vi "TI sbRIO Main (RT).vi"() -> ()   [LabVIEW 2013]
uses:
  Type Defs/Restarts Cluster.ctl
  Type Defs/Restarts Limits.ctl
  Type Defs/Controller Names.ctl
  Controls/HMI Mom Buttons.ctl
  Controls/Alarm Config.ctl
  Controls/Alarm Definition.ctl
  Controls/Alarm Profile Config.ctl
  Type Defs/App Config.ctl
  Type Defs/Actual Starts.ctl
  Type Defs/Sequence States.ctl
  Type Defs/CAN Mode.ctl
  Controls/RPi HMI Mode.ctl
  Type Defs/Controller List.ctl
  Type Defs/Pump Data Mode.ctl
  Controls/HMI Tog Buttons.ctl
  Controls/Controller Config.ctl
  SubVIs/TenHzDataArray(Global).vi
  <vilib>/FPGAPlugInAG/sbRIO-9626/niLvFpga_Open_sbRIO-9626.vi
  <vilib>/rvi/interface/common/dynamic/niFpgaDynamicAddResources.vi
  <vilib>/Utility/file.llb/Write To Spreadsheet File (DBL).vi
  SubVIs/Record Period (global).vi
  SubVIs/Record Samples (global).vi
  <vilib>/FPGAPlugInAG/Dynamic/niLvFpga_Reset_Dynamic.vi
  <vilib>/rvi/interface/common/niFpgaWaitOnOcc.vi
  <vilib>/Utility/error.llb/Error Cluster From Error Code.vi
  <vilib>/rvi/errors/niLvFpgaAdjustHostInterfaceError.vi
  <vilib>/FPGAPlugInAG/Dynamic/niLvFpga_Run_Dynamic.vi
  <vilib>/Utility/file.llb/Write To Spreadsheet File (string).vi
  <vilib>/rvi/interface/nirviOpenFPGA/nirviOpenFPGA.xnode
  FPGA/bitfiles/TI sbRIO PWM (FPGA) v1.0.lvbitx
  <vilib>/rvi/interface/nirviMethod/nirviMethod.xnode
  <vilib>/rvi/interface/nirviReadWriteControl/nirviReadWriteControl.xnode
  <vilib>/Utility/config.llb/NI_LVConfig.lvlib
  NiFpgaLv.dll
  <vilib>/NI_Real-Time Target Support.lvlib
  Real-Time/Controls/RT FIFO Mode.ctl
  <vilib>/rvi/interface/nirviCloseFPGA/nirviCloseFPGA.xnode
  Type Defs/JSON_Channel.ctl
  Type Defs/JSON_Pump.ctl
  Type Defs/JSON_Tank.ctl
  Controls/FPGA_Reference.ctl
  <vilib>/FPGAPlugInAG/sbRIO-9626/niLvFpga_Close_sbRIO-9626.vi
  <vilib>/rvi/interface/Simulation/niFpgaSimulationCallBeginRW.vi
  <vilib>/FPGAPlugInAG/sbRIO-9626/niLvFpga_Abort_sbRIO-9626.vi
panel:
  out "HMI Mom Buttons":T1
  out "TenHzPts":i32
  in  "TenHz Path":path=path "u:/TenHz/Try.csv"
  in  "Stop":bool
  in  "Alarm Tab":enum32{"Page 1", "Page 2"}(tab)
  out "Alarm Message":string
  in  "pb.Alarm OK":bool
  in  "Monitoring Tab":enum32{"Page 1", "Page 2"}(tab)
  in  "pb.E Stop":bool
  in  "Ignition Relay":T2
  in  "Power Relay":T2
  out "Voltages":dbl[](array[numeric])=[0.015201568603515625, 0.00335693359375, 0.003021240234375, 0.12260055541992188, 0.06085968017578125, 0.052234649658203125] caption="Pump\nVoltage\n(V)" format="%#.0f"
  out "Ave. Speed":dbl=7.74131899555212 format="%.1f"
  out "Temp2":dbl caption="Tank 2 Temp (C):" format="%#_2g"
  out "Temp1":dbl caption="Tank 1 Temp (C):" format="%#_2g"
  out "Pressure":dbl[](array[numeric])=[0.015201568603515625, 0.00335693359375, 0.003021240234375, 0.12260055541992188, 0.06085968017578125, 0.052234649658203125] caption="Pressure\n(kPa)" format="%#.0f"
  out "Flow":dbl[](array[numeric])=[0.0, 0.0, 0.0, 0.125, 0.0625, 0.0625] caption="Flow\n(L/H)" format="%#.0f"
  out "PumpCurrent":dbl[](array[numeric])=[0.015201568603515625, 0.00335693359375, 0.003021240234375, 0.12260055541992188, 0.06085968017578125, 0.052234649658203125] caption="Pump\nCurrent\n(RMS)" format="%#.1g"
  out "PS Actual (V):":dbl format="%.2f"
  out "ControllerCurrent":dbl[](array[numeric])=[0.015201568603515625, 0.00335693359375, 0.003021240234375, 0.12260055541992188, 0.06085968017578125, 0.052234649658203125] caption="Controller\nCurrent\n(DC)" format="%#.1g"
  out "Speed":dbl[](array[numeric]) caption="Speed\n(RPM)" format="%#_4f"
  in  "Power Supply Cmd (V):":dbl min=0.0 max=20.0 format="%#.2f"
  in  "PressureCMD":dbl caption="Pressure Cmd (kPa):" min=0.0 max=825.0 format="%#.2f"
  in  "Manual\nCMD":dbl[](array[numeric])=[0.0, 0.0, 0.0, 0.0, 0.0, 0.0] min=5.0 max=50.0 step=0.1 format="%#.2f"
  in  "pb.Zero CMDs":bool
  out "CPU Usage:":dbl=7.74131899555212 format="%.1f"
  in  "Pumps Present":T2={"Pump 1"=TRUE, "Pump 2"=TRUE, "Pump 3"=TRUE, "Pump 4"=TRUE, "Pump 5"=TRUE, "Pump 6"=TRUE}
  out "CAN CMD":dbl
  in  "Restarts Tab":enum32{"Page 1", "Page 2"}(tab)
  in  "Restarts Limits":T3={"High Limits:"=[30, 30, 30, 30, 30, 30], "Low Limits:"=[30, 30, 30, 30, 30, 30]}
  in  "pb.Rst Tot Restarts":bool
  in  "pb.Reset Restarts":bool
  in  "Inform:":string="Input email address on Email Handler program on Lab 4 PC."
  out "Restarts Cluster":T4
  out "Client?":bool
  in  "Title Tab":enum32{"Page 1", "Page 2"}(tab)
  in  "Title":string="TI Automotive sbRIO Pulse, v1.2"
  in  "Login":bool
  in  "Set Time Tab":enum32{"Page 1", "Page 2"}(tab)
  in  "pb.Set Time OK":bool
  in  "pb.Set Time Cancel":bool
  in  "New Time":dbl format="%<%H:%M:%S>t"
  in  "Reset Tab":enum32{"Page 1", "Page 2"}(tab)
  in  "pb.Reset OK":bool
  in  "pb.Reset Cancel":bool
  in  "pb.Stop Profile":bool
  in  "Save As Tab":enum32{"Page 1", "Page 2"}(tab)
  in  "New Profile Name:":string
  in  "pb.Save As OK":bool
  in  "pb.Save As Cancel":bool
  in  "Main Tab":enum32{"Main", "Data Stream", "Alarms"}(tab)
  in  "Profile:":string[][](table)=[["1", "2.0", "0.0", "0.0", "0.0", "67.6", "67.6", "67.6"], ["2", "1.0", "0.0", "0.0", "0.0", "10.0", "10.0", "10.0"]]
  in  "Controller Type:":T5
  in  "pb.FuelChange":bool
  in  "Tank 1 Fuel Type":string
  in  "Tank 2 Fuel Type":string
  in  "Stagger Time (ms):":i32
  in  "pb.Time Reset All":bool
  in  "CA Number:":string
  in  "Profile Name:":string(combo)="test"
  in  "pb.Save As":bool
  out "Current Step:":i32=2
  out "Step Time Left:":dbl=0.21101045608520508
  out "Cycles Completed:":u32=17
  in  "pb.Cycle Reset":bool
  out "Location:":string
  in  "pb.Run Profile":bool
  out "Elapsed Time:":dbl[](array[numeric])=[7.1, 7.1, 7.1, 458133.45, 458138.85000000003, 458126.75] format="%<%H:%M:%S>t"
  in  "pb.Resets":bool[](array[boolean])=[FALSE, FALSE, FALSE, FALSE, FALSE, FALSE]
  in  "pb.Sets":bool[](array[boolean])=[FALSE, FALSE, FALSE, FALSE, FALSE, FALSE]
  in  "Serial Numbers":T6
  in  "pb.TenHzSave":bool
  in  "Record Frequency:":i32=10 min=1 max=10 step=1
  in  "pb.Reset Cogs":bool
  in  "Cog Limits:":i32[](array[numeric])=[30, 30, 30, 30, 30, 30] min=0
  out "Cog Events:":i32[](array[numeric])
  out "Graph":dbl[](graph)
  in  "RPMhyst":fxp<+,25,6>=0.20000076293945312
  in  "Solenoid 3":bool caption="Fuel Solenoid 3"
  in  "Solenoid 2":bool caption="Fuel Solenoid 2"
  in  "Solenoid 1":bool caption="Fuel Solenoid 1"
  in  "3 Pulsing":bool caption="Module 3 Pulsing"
  in  "3 Pulse Duty%":dbl=60.0 caption="Module 3 Pulse Duty%" min=0.0 max=100.0 step=0.1 format="%#.2f"
  in  "2 Pulsing":bool caption="Module 2 Pulsing"
  in  "2 Pulse Duty%":dbl=60.0 caption="Module 2 Pulse Duty%" min=0.0 max=100.0 step=0.1 format="%#.2f"
  in  "1 Pulsing":bool caption="Module 1 Pulsing"
  in  "1 Pulse Duty%":dbl=60.0 caption="Module 1 Pulse Duty%" min=0.0 max=100.0 step=0.1 format="%#.2f"
  in  "Pulse Frequency":dbl=20.0 min=0.5 max=40.0 step=0.1 format="%#.2f"
  in  "SubRoutine Profile":i32[][](array[numeric]) caption="Profile #:   Cycles:" min=1 step=1
  in  "pb.Run SubRoutines":bool
  in  "Alarm Config":T7
  # "Manual Control"
  # "Monitoring"
  # "Restarts Monitor"
  # "Enter a new elapsed time."
  # "Are you sure you want to reset?"
  # "Under Development"
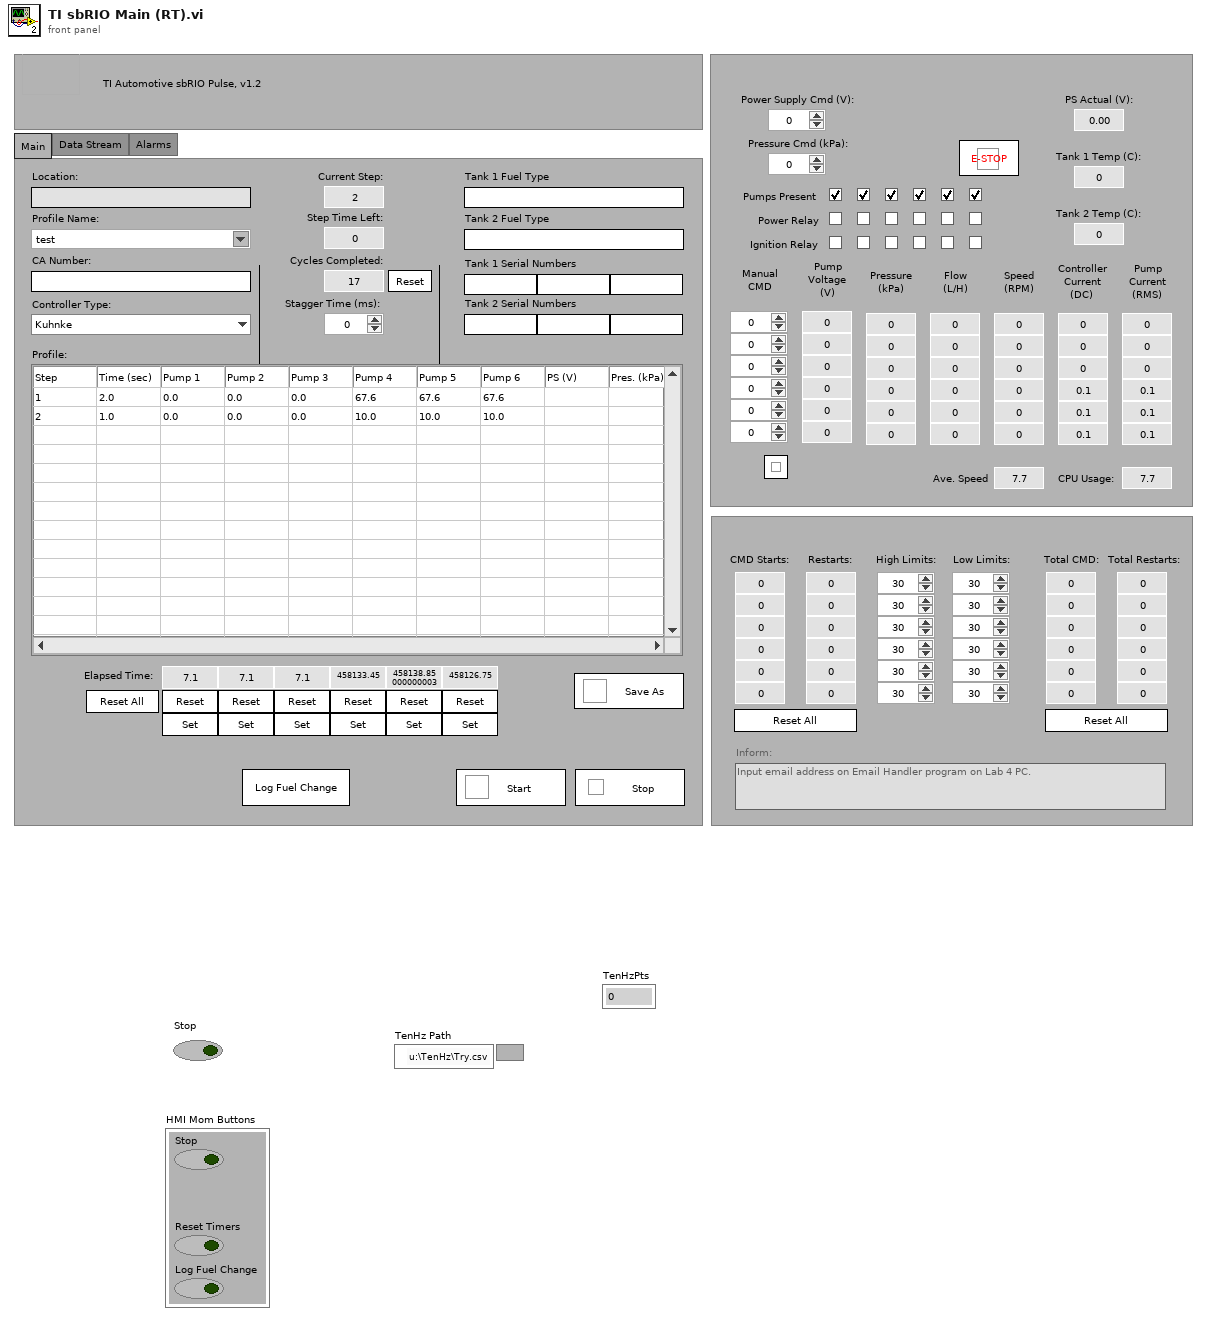
[diagram p1: front panel]
types:
  T1 = typedef "HMI Mom Buttons.ctl" = cluster{"Stop":bool, "Reset Timers":bool, "Log Fuel Change":bool}
  T2 = cluster{"Pump 1":bool, "Pump 2":bool, "Pump 3":bool, "Pump 4":bool, "Pump 5":bool, "Pump 6":bool}
  T3 = typedef "Restarts Limits.ctl" = cluster{"High Limits:":i32[], "Low Limits:":i32[]}
  T4 = typedef "Restarts Cluster.ctl" = cluster{"CMD Starts:":i32[], "Restarts:":i32[], "Total CMD:":i32[], "Total Restarts:":i32[]}
  T5 = typedef "Controller Names.ctl" = enum16{"Kuhnke", "Conti", "Helbako", "TI PWM", "PSA", "Hella Gas", "Hella Diesel", "8 Comm", "10 Comm", "8 Comm Hella", "10 Comm Hella", "8 Comm Omron", "10 Comm Omron", "8 Comm Nissan", "10 Comm Nissan"}
  T6 = cluster{"Position 1 SN":string, "Position 2 SN":string, "Position 3 SN":string, "Position 4 SN":string, "Position 5 SN":string, "Position 6 SN":string}
  T7 = typedef "Alarm Config.ctl" = cluster{"Alarms:":T8[], "Profile Sync:":T9}
  T8 = typedef "Alarm Definition.ctl" = cluster{"Description:":string, "Enabled:":bool, "Data Index:":i32, "Data Type:":string, "Low Limit:":dbl, "High Limit:":dbl, "Trip Time:":u32, "Profile Sync:":bool}
  T9 = typedef "Alarm Profile Config.ctl" = cluster{"Trip Time:":u32, "Consecutive Trips:":i32}
  T10 = typedef "Controller List.ctl" = cluster{"Controller Name":T5, "CommSeg":i32, "PWM?":bool, "Frequency":i32, "Low Command":dbl, "High Command":dbl, "Stop Command":dbl, "Command Step":dbl, "Solenoid Stop?":bool, "Controller?":bool, "Invert PWM":bool}[]
  T11 = cluster{"Controller Name":T5, "CommSeg":i32, "PWM?":bool, "Frequency":i32, "Low Command":dbl, "High Command":dbl, "Stop Command":dbl, "Command Step":dbl, "Solenoid Stop?":bool, "Controller?":bool, "Invert PWM":bool}
  T12 = typedef "RPi HMI Mode.ctl" = enum16{"Init", "Write Data", "Read from RPi", "Write to RPi"}
  T13 = typedef "CAN Mode.ctl" = enum16{"Init", "Read", "Write", "Close"}
  T14 = typedef "Sequence States.ctl" = enum16{"Main", "Init Files", "Init", "Save As", "Start Profile", "Check Step Time", "Alarm", "Run Step", "Stop Profile", "Cycle Reset", "Time Reset", "Time Reset All", "Time Set", "Tare CTs", "Save Profile", "Open Profile", "Get Profiles", "Update Screen", "Save Status", "Set Manual CMD", "Reset Restarts", "Reset Total Restarts", "Reset Cogs", "Disable Background", "Enable Background", "Get/Release Control", "Init AKLH", "Save AKLH", "Log Fuel Change", "Update Data Stream", "Init TenHz", "Read TenHz", "Remote Timer Reset", "Record Frequency Change", "Controller Change", "Get Alarms", "Init Alarms", "Save Alarms", "Init SubRoutine", "Next SubRoutine"}
  T15 = typedef "Actual Starts.ctl" = cluster{"Actual Pump Starts":i32[], "Initial Actual Starts":i32[], "Tot Act Starts":i32[], "Tot Init Act Starts":i32[]}
  T16 = typedef "App Config.ctl" = cluster{"Location":string, "Profiles Path":path, "Current Profile":string, "CA Number":string, "Cycles Completed":u32, "PWM Freq (Hz)":dbl, "Controller Type:":T5, "Inform":string, "Pumps Present":u32, "Stagger Time (ms)":i32, "Tank 1 Fuel":string, "Tank 2 Fuel":string, "Serial Numbers":cluster{"Position 1 SN":string, "Position 2 SN":string, "Poaition 3 SN":string, "Position 4 SN":string, "Position 5 SN":string, "Position 6 SN":string}, "Record TenHz":bool, "VoltCtrlRef":string, "TenHzFrequency":u32}
  T17 = cluster{"Error":errorcluster, "Profile":string[][], "App Config":T16, "Profiles":string[], "Current Step":i32, "Step Time Left":dbl, "Run Profile":bool, "Step Start Time":dbl, "Step Time":dbl, " # of Steps":i32, "Last Update":dbl, "Update Screen":bool, "Last Profile Time":dbl, "Manual CMDs":dbl[], "Client?":bool, "pb.Run Profile":bool, "pb.Resets":bool[], "pb.Sets":bool[], "Last CMDs":dbl[], "Update Profile":bool, "Elapsed Times":dbl[], "Intitial Times":dbl[], "Alarm":bool, "CT Offsets":fxp<+/-,26,7>[], "Pumps Present":cluster{"Pump 1":bool, "Pump 2":bool, "Pump 3":bool, "Pump 4":bool, "Pump 5":bool, "Pump 6":bool}, "Login":bool, "Stagger Counter":i32, "New Step":bool, "Restarts Limits":T3, "Restarts Cluster":T4, "Actual Starts":T15, "AKLH Path":path, "TenHz Path":path, "AKLH Timer":dbl, "TenHz Timer":dbl, "TenHz Active?":bool, "AKLH Last Hour":i32, "Main Tab":enum32{"Page 1", "Page 2"}, "Stop Cmd":dbl, "Tank Data":dbl[], "CogCounters":i32[], "Cog Events":i32[], "Voltage Enable":bool, "Cog Limits:":i32[], "TenHz Day":i32, "Controller":cluster{"Controller Name":T5, "CommSeg":i32, "PWM?":bool, "Frequency":i32, "Low Command":dbl, "High Command":dbl, "Stop Command":dbl, "Command Step":dbl, "Solenoid Stop?":bool, "Controller?":bool, "Invert PWM":bool}, "PS CMD":dbl, "Press CMD":dbl, "Temp CMD":dbl, "Power Relay":cluster{"Pump 1":bool, "Pump 2":bool, "Pump 3":bool, "Pump 4":bool, "Pump 5":bool, "Pump 6":bool}, "Ignition Relay":cluster{"Pump 1":bool, "Pump 2":bool, "Pump 3":bool, "Pump 4":bool, "Pump 5":bool, "Pump 6":bool}, "Controller List":T10, "Alarm Config":T7, "Alarm Config Path":path, "Trip Counters":i32[], "Previous Times":u32[], "Alarm Message":string, "Restart Alarm":bool, "Pulse Frequency":dbl, "1 Pulse Duty%":dbl, "2 Pulse Duty%":dbl, "3 Pulse Duty%":dbl, "1 Pulsing":bool, "Solenoid 1":bool, "2 Pulsing":bool, "Solenoid 2":bool, "3 Pulsing":bool, "Solenoid 3":bool, "SubRoutine Profile":i32[][], "Profile #":i32, "ReqCycles":u32, "Run Subs":bool, "SR Step":u32}
  T18 = typedef "HMI Cluster.ctl" = cluster{"Error":errorcluster, "COM Ref":refnum<visa-resource-name>, "Pump Data":T19, "Tank Data":cluster{"PS Actual (V):":dbl, "Temp1":dbl, "Temp2":dbl}, "Power Relays":cluster{"Pump 1":bool, "Pump 2":bool, "Pump 3":bool, "Pump 4":bool, "Pump 5":bool, "Pump 6":bool}, "Pump CMDs":dbl[], "HMI Header":T20, "Tank CMDs":T21, "HMI Tog Buttons":T22, "In Test":bool, "HMI Command":bool, "HMI Mom Buttons":T1, "Controller Config":T23}
  T19 = typedef "Pump Data.ctl" = cluster{"Voltages":dbl[], "PumpCurrent":dbl[], "Speed":dbl[], "ControllerCurrent":dbl[], "Pressure":dbl[], "Flow":dbl[], "Elapsed Time:":dbl[]}
  T20 = typedef "HMI Header.ctl" = cluster{"Line 1":string, "Line 2":string, "Line 3":string}
  T21 = typedef "Tank CMDs.ctl" = cluster{"PS CMD":dbl, "Press CMD":dbl, "Temp CMD":dbl}
  T22 = typedef "HMI Tog Buttons.ctl" = cluster{"Start Test":bool, "Toggle Spare 1":bool, "Toggle Spare 2":bool, "Toggle Spare 3":bool, "Toggle Spare 4":bool, "Toggle Spare 5":bool}
  T23 = typedef "Controller Config.ctl" = cluster{"Controller List":string, "Controller Type:":T5, "CMD Max":i32, "CMD Inc":i32}
  T24 = typedef "RT FIFO Mode.ctl" = enum16{"Create", "Write", "Read", "Delete"}
  T25 = typedef "FPGA_Reference.ctl" = refnum<k20>
  T26 = typedef "Pump Data Mode.ctl" = enum16{"Read", "Write Data", "Write Cal"}
  T27 = enum8{"Enabled", "Disabled", "Disabled and Grayed Out"}
  T28 = typedef "JSON_Tank.ctl" = cluster{"number":u16, "building":string, "room":string, "ipAddress":string, "profileName":string, "caNumber":string, "ctrlType":string, "mode":string, "channels":T29[], "pumps":T30[]}
  T29 = typedef "JSON_Channel.ctl" = cluster{"name":string, "tag":string, "data":string, "type":string, "unit":string}
  T30 = typedef "JSON_Pump.ctl" = cluster{"position":u8, "enabled":bool, "command":string, "channels":T29[], "elapsedTime":string}
  T31 = cluster{"Position 1 SN":string, "Position 2 SN":string, "Poaition 3 SN":string, "Position 4 SN":string, "Position 5 SN":string, "Position 6 SN":string}
  T32 = typedef "Test Action.ctl" = enum16{"Idle", "Start", "Stop", "Pump Cmd", "Pump 1 Enable", "Pump 2 Enable", "Pump 3 Enable", "Pump 4 Enable", "Pump 5 Enable", "Pump 6 Enable", "Timer 1 Reset", "Timer 2 Reset", "Timer 3 Reset", "Timer 4 Reset", "Timer 5 Reset", "Timer 6 Reset"}
  T33 = cluster{"Boolean array[0]":bool, "Boolean array[1]":bool, "Boolean array[2]":bool, "Boolean array[3]":bool, "Boolean array[4]":bool, "Boolean array[5]":bool}
  T34 = typedef "LVDateTimeRec.ctl" = cluster{"fractional second":dbl, "second":i32, "minute":i32, "hour":i32, "day of month":i32, "month":i32, "year":i32, "day of week":i32, "day of year":i32, "DST":i32}
  T35 = typedef "NI_LVConfig.lvlib/Config Data RefNum.ctl" = refnum<k1>
  T36 = cluster{dbl, dbl, dbl, dbl, dbl, dbl, dbl, dbl, dbl, dbl, dbl, dbl}
  T37 = cluster{"PS Actual (V):":dbl, "Temp1":dbl, "Temp2":dbl}
  T38 = cluster{"Location":string, "Current Profile":string, "CA Number":string}
  T39 = cluster{"PS CMD":dbl, "Press CMD":dbl, "Temp CMD":dbl}
  T40 = typedef "LVRemotePanelConnectionsTypeDef.ctl" = cluster{"VI Name":string, "Remote":string, "UserName":string, "Port":i32, "Status":enum32{"Viewing", "Waiting For Control", "Controlling"}, "Create Time":timestamp, "Status Time":timestamp, "Control End Time":timestamp}[]
  T41 = typedef "NI_Real-Time Target Support.lvlib/RT CPU Load.ctl" = cluster{"Total (%)":dbl, "Time Critical (%)":dbl, "Timed Structures (%)":dbl, "High (%)":dbl, "Above Normal (%)":dbl, "Normal (%)":dbl, "Background (%)":dbl, "Idle (%)":dbl, "ISR (%)":dbl}
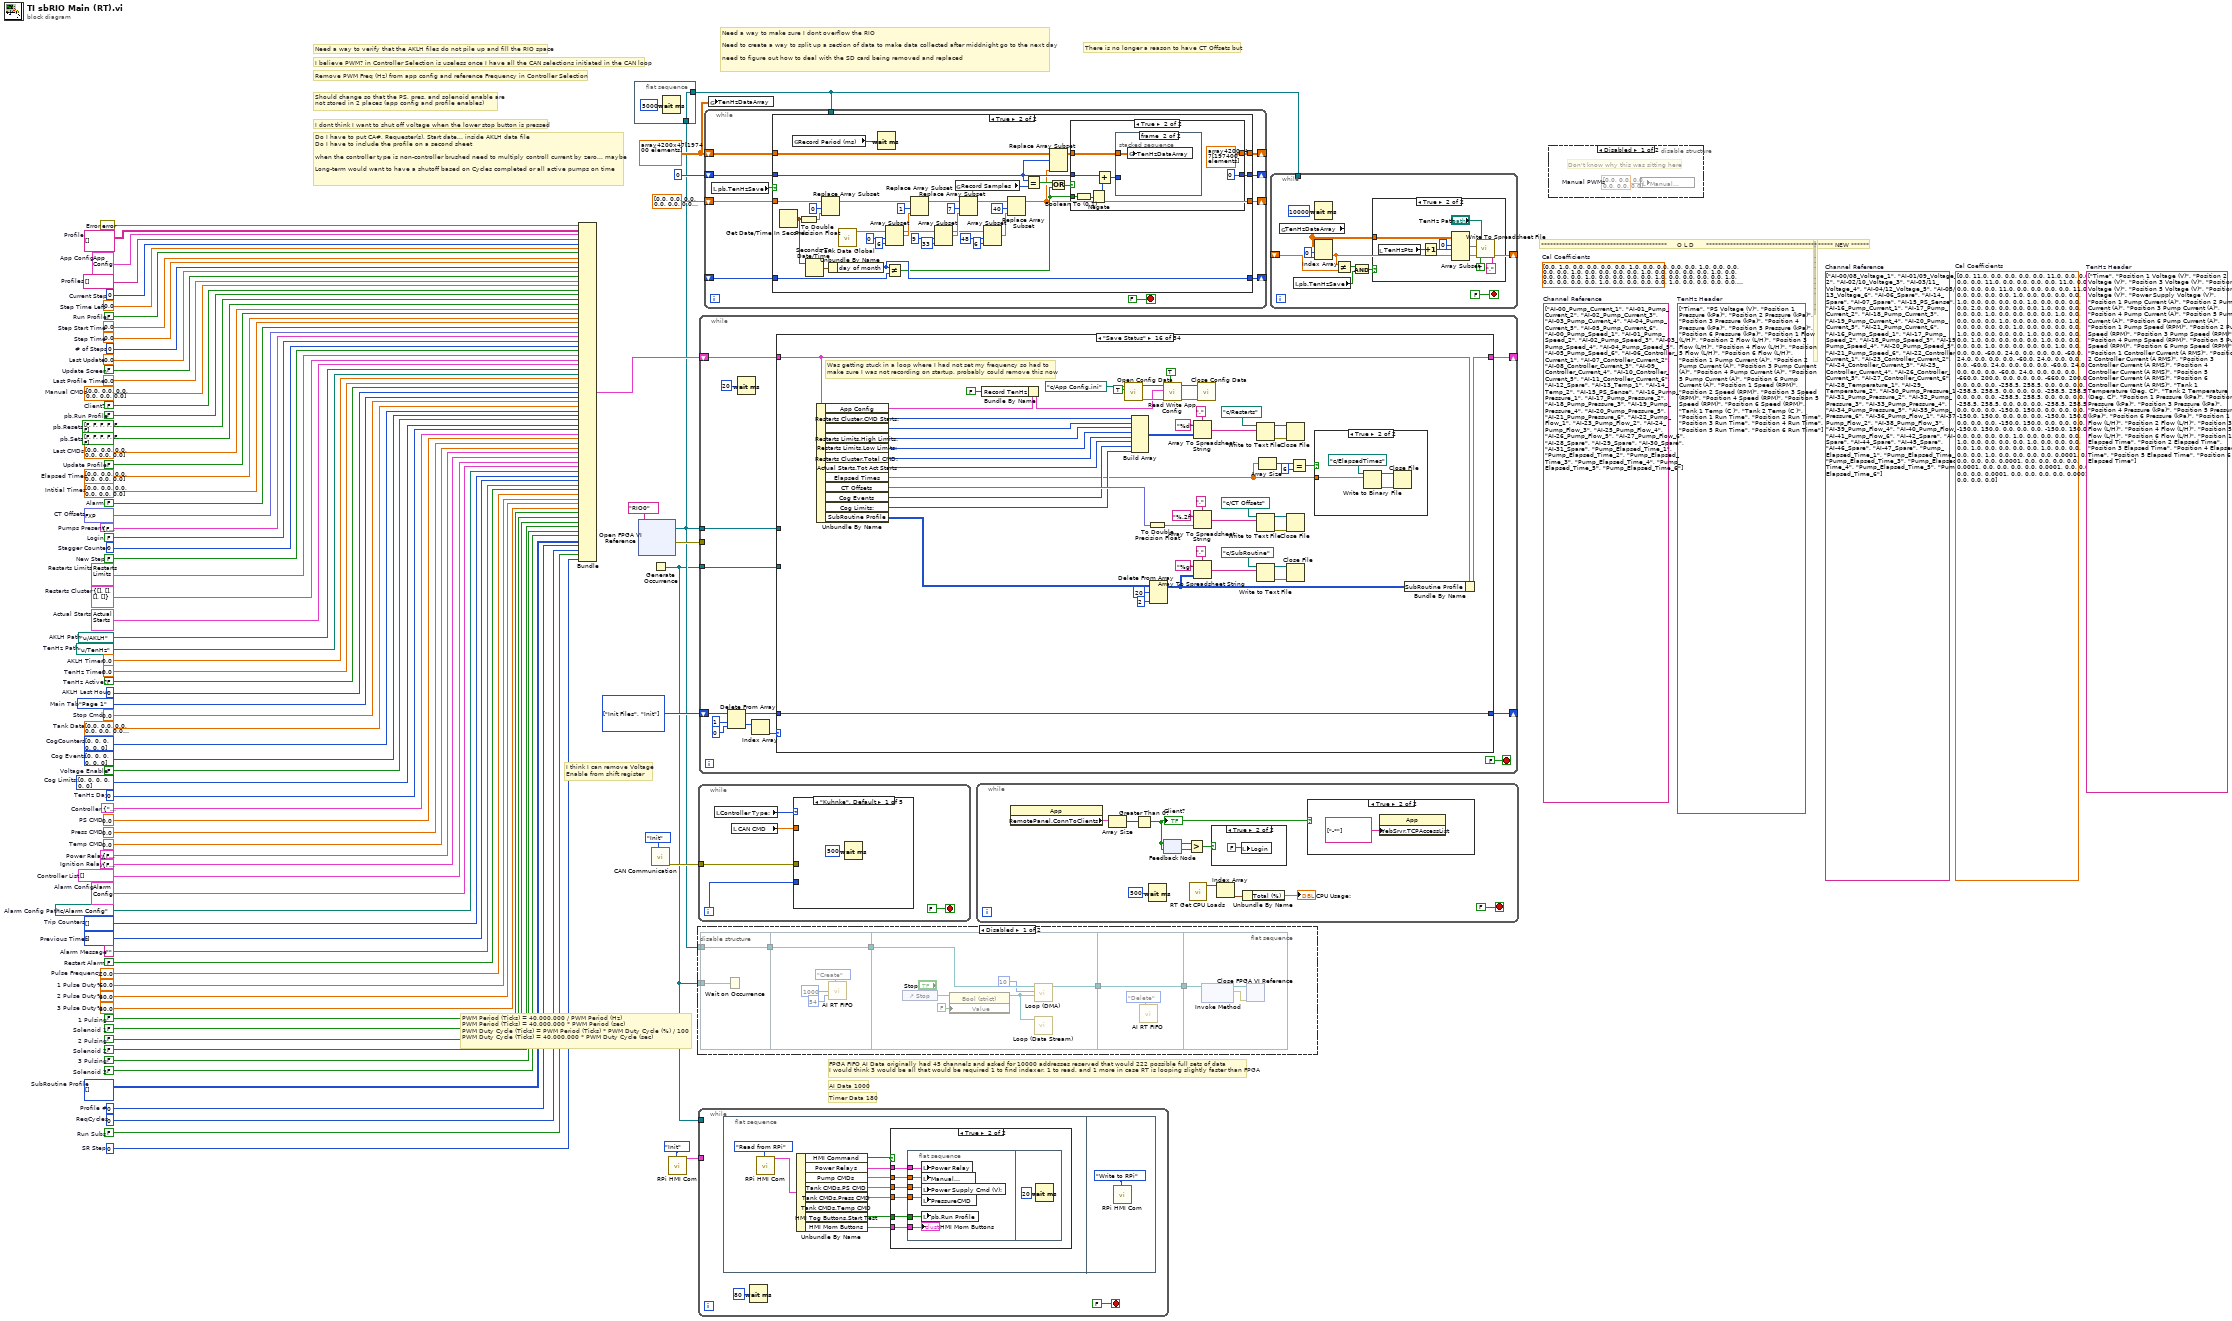
[diagram p0: block diagram]
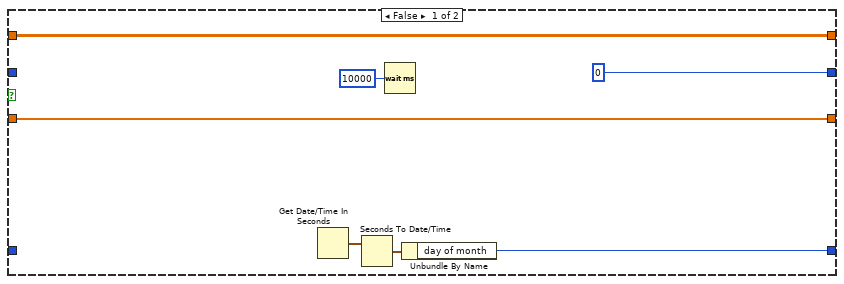
[diagram p5: hidden frame]
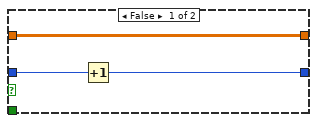
[diagram p6: hidden frame]
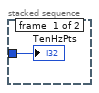
[diagram p7: hidden frame]
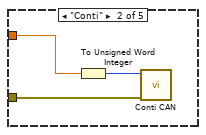
[diagram p8: hidden frame]
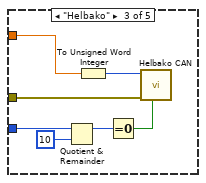
[diagram p9: hidden frame]
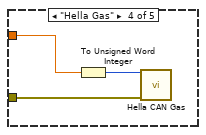
[diagram p10: hidden frame]
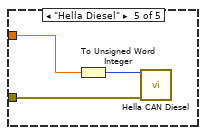
[diagram p11: hidden frame]
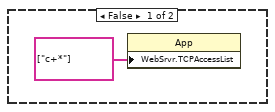
[diagram p12: hidden frame]
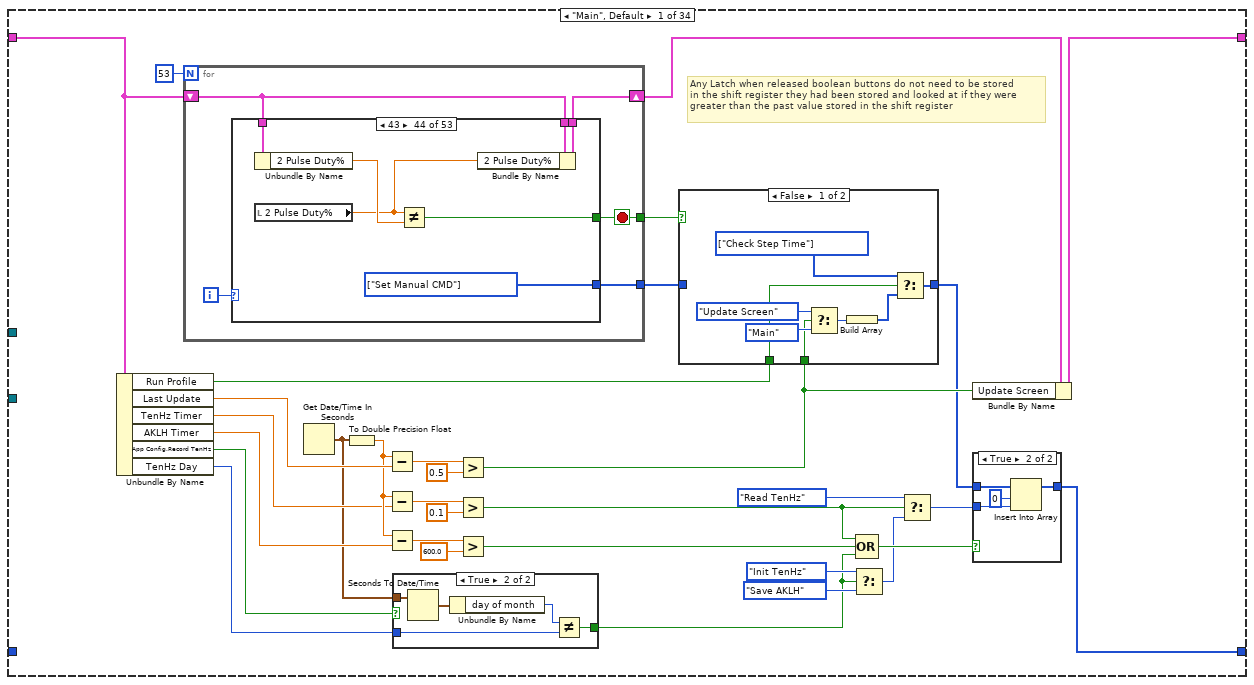
[diagram p15: hidden frame]
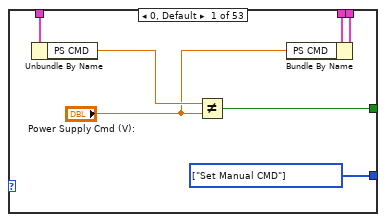
[diagram p18: hidden frame]
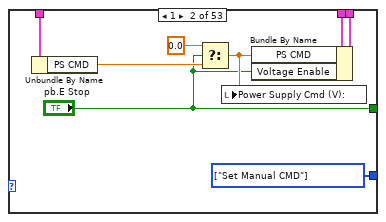
[diagram p19: hidden frame]
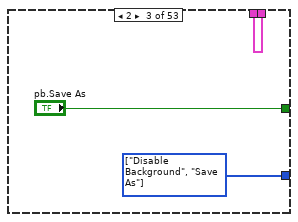
[diagram p20: hidden frame]
diagram:
  w5 = u32 0  # SR Step
  w4 = FALSE  # Run Subs
  w3 = u32 0  # ReqCycles
  w2 = 0  # Profile #
  w1 = i32[][] []  # SubRoutine Profile
  w6 = FALSE  # Solenoid 3
  w7 = FALSE  # 3 Pulsing
  w8 = FALSE  # Solenoid 2
  w9 = FALSE  # 2 Pulsing
  w10 = FALSE  # Solenoid 1
  w11 = FALSE  # 1 Pulsing
  w12 = 60.0  # 3 Pulse Duty%
  w13 = 60.0  # 2 Pulse Duty%
  w14 = 60.0  # 1 Pulse Duty%
  w15 = 20.0  # Pulse Frequency
  w16 = FALSE  # Restart Alarm
  w17 = ""  # Alarm Message
  w18 = u32[] []  # Previous Times
  w19 = i32[] []  # Trip Counters
  w20 = path "c:/Alarm Config"  # Alarm Config Path
  w21 = T7 {"Alarms:"=[{"Description:"="", "Enabled:"=FALSE, "Data Index:"=0, "Data Type:"="", "Low Limit:"=0.0, "High Limit:"=0.0, "Trip Time:"=0, "Profile Sync:"=FALSE}, {"Description:"="", "Enabled:"=FALSE, "Data Index:"=0, "Data Type:"="", "Low Limit:"=0.0, "High Limit:"=0.0, "Trip Time:"=0, "Profile Sync:"=FALSE}, {"Description:"="", "Enabled:"=FALSE, "Data Index:"=0, "Data Type:"="", "Low Limit:"=0.0, "High Limit:"=0.0, "Trip Time:"=0, "Profile Sync:"=FALSE}, {"Description:"="", "Enabled:"=FALSE, "Data Index:"=0, "Data Type:"="", "Low Limit:"=0.0, "High Limit:"=0.0, "Trip Time:"=0, "Profile Sync:"=FALSE}, {"Description:"="", "Enabled:"=FALSE, "Data Index:"=0, "Data Type:"="", "Low Limit:"=0.0, "High Limit:"=0.0, "Trip Time:"=0, "Profile Sync:"=FALSE}, {"Description:"="", "Enabled:"=FALSE, "Data Index:"=0, "Data Type:"="", "Low Limit:"=0.0, "High Limit:"=0.0, "Trip Time:"=0, "Profile Sync:"=FALSE}, {"Description:"="", "Enabled:"=FALSE, "Data Index:"=0, "Data Type:"="", "Low Limit:"=0.0, "High Limit:"=0.0, "Trip Time:"=0, "Profile Sync:"=FALSE}, {"Description:"="", "Enabled:"=FALSE, "Data Index:"=0, "Data Type:"="", "Low Limit:"=0.0, "High Limit:"=0.0, "Trip Time:"=0, "Profile Sync:"=FALSE}], "Profile Sync:"={"Trip Time:"=0, "Consecutive Trips:"=0}}  # Alarm Config
  w22 = T10 []  # Controller List
  w23 = T11 {"Controller Name"=enum."Kuhnke", "CommSeg"=2, "PWM?"=TRUE, "Frequency"=100, "Low Command"=10.0, "High Command"=100.0, "Stop Command"=10.0, "Command Step"=0.1, "Solenoid Stop?"=FALSE, "Controller?"=TRUE, "Invert PWM"=FALSE}  # Controller
  w27 = T2 {"Pump 1"=FALSE, "Pump 2"=FALSE, "Pump 3"=FALSE, "Pump 4"=FALSE, "Pump 5"=FALSE, "Pump 6"=FALSE}  # Ignition Relay
  w28 = T2 {"Pump 1"=FALSE, "Pump 2"=FALSE, "Pump 3"=FALSE, "Pump 4"=FALSE, "Pump 5"=FALSE, "Pump 6"=FALSE}  # Power Relay
  w29 = 0.0  # Temp CMD
  w30 = 0.0  # Press CMD
  w31 = 0.0  # PS CMD
  (unwired) string[] ["Time", "Position 1 Voltage (V)", "Position 2 Voltage (V)", "Position 3 Voltage (V)", "Position 4 Voltage (V)", "Position 5 Voltage (V)", "Position 6 Voltage (V)", "Power Supply Voltage (V)", "Position 1 Pump Current (A)", "Position 2 Pump Current (A)", "Position 3 Pump Current (A)", "Position 4 Pump Current (A)", "Position 5 Pump Current (A)", "Position 6 Pump Current (A)", "Position 1 Pump Speed (RPM)", "Position 2 Pump Speed (RPM)", "Position 3 Pump Speed (RPM)", "Position 4 Pump Speed (RPM)", "Position 5 Pump Speed (RPM)", "Position 6 Pump Speed (RPM)", "Position 1 Controller Current (A RMS)", "Position 2 Controller Current (A RMS)", "Position 3 Controller Current (A RMS)", "Position 4 Controller Current (A RMS)", "Position 5 Controller Current (A RMS)", "Position 6 Controller Current (A RMS)", "Tank 1 Temperature (Deg. C)", "Tank 2 Temperature (Deg. C)", "Position 1 Pressure (kPa)", "Position 2 Pressure (kPa)", "Position 3 Pressure (kPa)", "Position 4 Pressure (kPa)", "Position 5 Pressure (kPa)", "Position 6 Pressure (kPa)", "Position 1 Flow (L/H)", "Position 2 Flow (L/H)", "Position 3 Flow (L/H)", "Position 4 Flow (L/H)", "Position 5 Flow (L/H)", "Position 6 Flow (L/H)", "Position 1 Elapsed Time", "Position 2 Elapsed Time", "Position 3 Elapsed Time", "Position 4 Elapsed Time", "Position 5 Elapsed Time", "Position 6 Elapsed Time"]  # TenHz Header
  (unwired) dbl[][] [[0.0, 11.0, 0.0, 0.0, 0.0], [0.0, 11.0, 0.0, 0.0, 0.0], [0.0, 11.0, 0.0, 0.0, 0.0], [0.0, 11.0, 0.0, 0.0, 0.0], [0.0, 11.0, 0.0, 0.0, 0.0], [0.0, 11.0, 0.0, 0.0, 0.0], [0.0, 1.0, 0.0, 0.0, 0.0], [0.0, 1.0, 0.0, 0.0, 0.0], [0.0, 1.0, 0.0, 0.0, 0.0], [0.0, 2.0, 0.0, 0.0, 0.0], [0.0, 1.0, 0.0, 0.0, 0.0], [0.0, 1.0, 0.0, 0.0, 0.0], [0.0, 1.0, 0.0, 0.0, 0.0], [0.0, 1.0, 0.0, 0.0, 0.0], [0.0, 1.0, 0.0, 0.0, 0.0], [0.0, 1.0, 0.0, 0.0, 0.0], [0.0, 1.0, 0.0, 0.0, 0.0], [0.0, 1.0, 0.0, 0.0, 0.0], [0.0, 1.0, 0.0, 0.0, 0.0], [0.0, 1.0, 0.0, 0.0, 0.0], [0.0, 1.0, 0.0, 0.0, 0.0], [0.0, 1.0, 0.0, 0.0, 0.0], [-60.0, 24.0, 0.0, 0.0, 0.0], [-60.0, 24.0, 0.0, 0.0, 0.0], [-60.0, 24.0, 0.0, 0.0, 0.0], [-60.0, 24.0, 0.0, 0.0, 0.0], [-60.0, 24.0, 0.0, 0.0, 0.0], [-60.0, 24.0, 0.0, 0.0, 0.0], [-660.0, 200.0, 0.0, 0.0, 0.0], [-660.0, 200.0, 0.0, 0.0, 0.0], [-258.5, 258.5, 0.0, 0.0, 0.0], [-258.5, 258.5, 0.0, 0.0, 0.0], [-258.5, 258.5, 0.0, 0.0, 0.0], [-258.5, 258.5, 0.0, 0.0, 0.0], [-258.5, 258.5, 0.0, 0.0, 0.0], [-258.5, 258.5, 0.0, 0.0, 0.0], [-150.0, 150.0, 0.0, 0.0, 0.0], [-150.0, 150.0, 0.0, 0.0, 0.0], [-150.0, 150.0, 0.0, 0.0, 0.0], [-150.0, 150.0, 0.0, 0.0, 0.0], [-150.0, 150.0, 0.0, 0.0, 0.0], [-150.0, 150.0, 0.0, 0.0, 0.0], [0.0, 1.0, 0.0, 0.0, 0.0], [0.0, 1.0, 0.0, 0.0, 0.0], [0.0, 1.0, 0.0, 0.0, 0.0], [0.0, 1.0, 0.0, 0.0, 0.0], [0.0, 1.0, 0.0, 0.0, 0.0], [0.0, 1.0, 0.0, 0.0, 0.0], [0.0, 0.0001, 0.0, 0.0, 0.0], [0.0, 0.0001, 0.0, 0.0, 0.0], [0.0, 0.0001, 0.0, 0.0, 0.0], [0.0, 0.0001, 0.0, 0.0, 0.0], [0.0, 0.0001, 0.0, 0.0, 0.0], [0.0, 0.0001, 0.0, 0.0, 0.0]]  # Cal Coefficients
  (unwired) dbl[][] [[0.0, 1.0, 0.0, 0.0, 0.0], [0.0, 1.0, 0.0, 0.0, 0.0], [0.0, 1.0, 0.0, 0.0, 0.0], [0.0, 1.0, 0.0, 0.0, 0.0], [0.0, 1.0, 0.0, 0.0, 0.0], [0.0, 1.0, 0.0, 0.0, 0.0], [0.0, 1.0, 0.0, 0.0, 0.0], [0.0, 1.0, 0.0, 0.0, 0.0], [0.0, 1.0, 0.0, 0.0, 0.0], [0.0, 1.0, 0.0, 0.0, 0.0], [0.0, 1.0, 0.0, 0.0, 0.0], [0.0, 1.0, 0.0, 0.0, 0.0], [-60.0, 24.0, 0.0, 0.0, 0.0], [-60.0, 24.0, 0.0, 0.0, 0.0], [-60.0, 24.0, 0.0, 0.0, 0.0], [-60.0, 24.0, 0.0, 0.0, 0.0], [-60.0, 24.0, 0.0, 0.0, 0.0], [-60.0, 24.0, 0.0, 0.0, 0.0], [0.0, 1.0, 0.0, 0.0, 0.0], [-660.0, 200.0, 0.0, 0.0, 0.0], [-660.0, 200.0, 0.0, 0.0, 0.0], [0.0, 2.0, 0.0, 0.0, 0.0], [-258.5, 258.5, 0.0, 0.0, 0.0], [-258.5, 258.5, 0.0, 0.0, 0.0], [-258.5, 258.5, 0.0, 0.0, 0.0], [-258.5, 258.5, 0.0, 0.0, 0.0], [-258.5, 258.5, 0.0, 0.0, 0.0], [-258.5, 258.5, 0.0, 0.0, 0.0], [-150.0, 150.0, 0.0, 0.0, 0.0], [-150.0, 150.0, 0.0, 0.0, 0.0], [-150.0, 150.0, 0.0, 0.0, 0.0], [-150.0, 150.0, 0.0, 0.0, 0.0], [-150.0, 150.0, 0.0, 0.0, 0.0], [-150.0, 150.0, 0.0, 0.0, 0.0], [0.0, 1.0, 0.0, 0.0, 0.0], [0.0, 1.0, 0.0, 0.0, 0.0], [0.0, 1.0, 0.0, 0.0, 0.0], [0.0, 1.0, 0.0, 0.0, 0.0], [0.0, 0.0001, 0.0, 0.0, 0.0], [0.0, 0.0001, 0.0, 0.0, 0.0], [0.0, 0.0001, 0.0, 0.0, 0.0], [0.0, 0.0001, 0.0, 0.0, 0.0], [0.0, 0.0001, 0.0, 0.0, 0.0], [0.0, 0.0001, 0.0, 0.0, 0.0]]  # Cal Coefficients
  (unwired) string[] ["AI-00/08_Voltage_1", "AI-01/09_Voltage_2", "AI-02/10_Voltage_3", "AI-03/11_Voltage_4", "AI-04/12_Voltage_5", "AI-05/13_Voltage_6", "AI-06_Spare", "AI-14_Spare", "AI-07_Spare", "AI-15_PS_Sense", "AI-16_Pump_Current_1", "AI-17_Pump_Current_2", "AI-18_Pump_Current_3", "AI-19_Pump_Current_4", "AI-20_Pump_Current_5", "AI-21_Pump_Current_6", "AI-16_Pump_Speed_1", "AI-17_Pump_Speed_2", "AI-18_Pump_Speed_3", "AI-19_Pump_Speed_4", "AI-20_Pump_Speed_5", "AI-21_Pump_Speed_6", "AI-22_Controller_Current_1", "AI-23_Controller_Current_2", "AI-24_Controller_Current_3", "AI-25_Controller_Current_4", "AI-26_Controller_Current_5", "AI-27_Controller_Current_6", "AI-28_Temperature_1", "AI-29_Temperature_2", "AI-30_Pump_Pressure_1", "AI-31_Pump_Pressure_2", "AI-32_Pump_Pressure_3", "AI-33_Pump_Pressure_4", "AI-34_Pump_Pressure_5", "AI-35_Pump_Pressure_6", "AI-36_Pump_Flow_1", "AI-37_Pump_Flow_2", "AI-38_Pump_Flow_3", "AI-39_Pump_Flow_4", "AI-40_Pump_Flow_5", "AI-41_Pump_Flow_6", "AI-42_Spare", "AI-43_Spare", "AI-44_Spare", "AI-45_Spare", "AI-46_Spare", "AI-47_Spare", "Pump_Elapsed_Time_1", "Pump_Elapsed_Time_2", "Pump_Elapsed_Time_3", "Pump_Elapsed_Time_4", "Pump_Elapsed_Time_5", "Pump_Elapsed_Time_6"]  # Channel Reference
  (unwired) string[] ["Time", "PS Voltage (V)", "Position 1 Pressure (kPa)", "Position 2 Pressure (kPa)", "Position 3 Pressure (kPa)", "Position 4 Pressure (kPa)", "Position 5 Pressure (kPa)", "Position 6 Pressure (kPa)", "Position 1 Flow (L/H)", "Position 2 Flow (L/H)", "Position 3 Flow (L/H)", "Position 4 Flow (L/H)", "Position 5 Flow (L/H)", "Position 6 Flow (L/H)", "Position 1 Pump Current (A)", "Position 2 Pump Current (A)", "Position 3 Pump Current (A)", "Position 4 Pump Current (A)", "Position 5 Pump Current (A)", "Position 6 Pump Current (A)", "Position 1 Speed (RPM)", "Position 2 Speed (RPM)", "Position 3 Speed (RPM)", "Position 4 Speed (RPM)", "Position 5 Speed (RPM)", "Position 6 Speed (RPM)", "Tank 1 Temp (C )", "Tank 2 Temp (C )", "Position 1 Run Time", "Position 2 Run Time", "Position 3 Run Time", "Position 4 Run Time", "Position 5 Run Time", "Position 6 Run Time"]  # TenHz Header
  w37 = 0  # TenHz Day
  w38 = dbl[][] array4200x47[197400 elements]
  w41 = i32[] [0, 0, 0, 0, 0, 0]  # Cog Limits:
  w42 = FALSE  # Voltage Enable
  w43 = i32[] [0, 0, 0, 0, 0, 0]  # Cog Events
  w44 = i32[] [0, 0, 0, 0, 0, 0]  # CogCounters
  w46 = dbl[] [0.0, 0.0, 0.0, 0.0, 0.0, 0.0, 0.0, 0.0, 0.0, 0.0, 0.0, 0.0, 0.0, 0.0, 0.0, 0.0, 0.0, 0.0, 0.0, 0.0, 0.0, 0.0, 0.0, 0.0, 0.0, 0.0, 0.0, 0.0, 0.0, 0.0, 0.0, 0.0, 0.0, 0.0, 0.0, 0.0, 0.0, 0.0, 0.0, 0.0, 0.0, 0.0, 0.0, 0.0]  # Tank Data
  (unwired) string[] ["AI-00_Pump_Current_1", "AI-01_Pump_Current_2", "AI-02_Pump_Current_3", "AI-03_Pump_Current_4", "AI-04_Pump_Current_5", "AI-05_Pump_Current_6", "AI-00_Pump_Speed_1", "AI-01_Pump_Speed_2", "AI-02_Pump_Speed_3", "AI-03_Pump_Speed_4", "AI-04_Pump_Speed_5", "AI-05_Pump_Speed_6", "AI-06_Controller_Current_1", "AI-07_Controller_Current_2", "AI-08_Controller_Current_3", "AI-09_Controller_Current_4", "AI-10_Controller_Current_5", "AI-11_Controller_Current_6", "AI-12_Spare", "AI-13_Temp_1", "AI-14_Temp_2", "AI-15_PS_Sense", "AI-16_Pump_Pressure_1", "AI-17_Pump_Pressure_2", "AI-18_Pump_Pressure_3", "AI-19_Pump_Pressure_4", "AI-20_Pump_Pressure_5", "AI-21_Pump_Pressure_6", "AI-22_Pump_Flow_1", "AI-23_Pump_Flow_2", "AI-24_Pump_Flow_3", "AI-25_Pump_Flow_4", "AI-26_Pump_Flow_5", "AI-27_Pump_Flow_6", "AI-28_Spare", "AI-29_Spare", "AI-30_Spare", "AI-31_Spare", "Pump_Elapsed_Time_1", "Pump_Elapsed_Time_2", "Pump_Elapsed_Time_3", "Pump_Elapsed_Time_4", "Pump_Elapsed_Time_5", "Pump_Elapsed_Time_6"]  # Channel Reference
  w47 = 0.0  # Stop Cmd
  w48 = enum32{"Page 1", "Page 2"}."Page 1"  # Main Tab
  w49 = 0  # AKLH Last Hour
  w50 = FALSE  # TenHz Active?
  w51 = 0.0  # TenHz Timer
  w52 = 0.0  # AKLH Timer
  w53 = path "u:/TenHz"  # TenHz Path
  w54 = path "u:/AKLH"  # AKLH Path
  w55 = fxp<+/-,26,7>[] [0.0, 0.0, 0.0, 0.0, 0.0, 0.0]  # CT Offsets
  w56 = T14[] [enum."Init Files", enum."Init"] items=["Main", "Init Files", "Init", "Save As", "Start Profile", "Check Step Time", "Alarm", "Run Step", "Stop Profile", "Cycle Reset", "Time Reset", "Time Reset All", "Time Set", "Tare CTs", "Save Profile", "Open Profile", "Get Profiles", "Update Screen", "Save Status", "Set Manual CMD", "Reset Restarts", "Reset Total Restarts", "Reset Cogs", "Disable Background", "Enable Background", "Get/Release Control", "Init AKLH", "Save AKLH", "Log Fuel Change", "Update Data Stream", "Init TenHz", "Read TenHz", "Remote Timer Reset", "Record Frequency Change", "Controller Change", "Get Alarms", "Init Alarms", "Save Alarms", "Init SubRoutine", "Next SubRoutine"]
  w58 = T15 {"Actual Pump Starts"=[0, 0, 0, 0, 0, 0], "Initial Actual Starts"=[0, 0, 0, 0, 0, 0], "Tot Act Starts"=[0, 0, 0, 0, 0, 0], "Tot Init Act Starts"=[0, 0, 0, 0, 0, 0]}  # Actual Starts
  w59 = T4 {"CMD Starts:"=[], "Restarts:"=[], "Total CMD:"=[], "Total Restarts:"=[]}  # Restarts Cluster
  w60 = T3 {"High Limits:"=[30, 30, 30, 30, 30, 30], "Low Limits:"=[30, 30, 30, 30, 30, 30]}  # Restarts Limits
  w61 = FALSE  # New Step
  w62 = 0  # Stagger Counter
  w63 = FALSE  # Login
  w64 = T2 {"Pump 1"=FALSE, "Pump 2"=FALSE, "Pump 3"=FALSE, "Pump 4"=FALSE, "Pump 5"=FALSE, "Pump 6"=FALSE}  # Pumps Present
  w65 = FALSE  # Alarm
  w66 = dbl[] [0.0, 0.0, 0.0, 0.0, 0.0, 0.0]  # Intitial Times
  w67 = dbl[] [0.0, 0.0, 0.0, 0.0, 0.0, 0.0]  # Elapsed Times
  w68 = FALSE  # Update Profile
  w69 = dbl[] [0.0, 0.0, 0.0, 0.0, 0.0, 0.0]  # Last CMDs
  w70 = bool[] [FALSE, FALSE, FALSE, FALSE, FALSE, FALSE]  # pb.Sets
  w71 = bool[] [FALSE, FALSE, FALSE, FALSE, FALSE, FALSE]  # pb.Resets
  w72 = FALSE  # pb.Run Profile
  w73 = FALSE  # Client?
  w74 = dbl[] [0.0, 0.0, 0.0, 0.0, 0.0, 0.0]  # Manual CMDs
  w75 = 0.0  # Last Profile Time
  w76 = FALSE  # Update Screen
  w77 = 0.0  # Last Update
  w78 = 0  # # of Steps
  w79 = 0.0  # Step Time
  w80 = 0.0  # Step Start Time
  w81 = FALSE  # Run Profile
  w83 = 0  # Current Step
  w82 = 0.0  # Step Time Left
  w84 = string[] []  # Profiles
  w85 = T16 {"Location"="", "Profiles Path"=path "", "Current Profile"="", "CA Number"="", "Cycles Completed"=0, "PWM Freq (Hz)"=0.0, "Controller Type:"=enum."Kuhnke", "Inform"="", "Pumps Present"=0, "Stagger Time (ms)"=0, "Tank 1 Fuel"="", "Tank 2 Fuel"="", "Serial Numbers"={"Position 1 SN"="", "Position 2 SN"="", "Poaition 3 SN"="", "Position 4 SN"="", "Position 5 SN"="", "Position 6 SN"=""}, "Record TenHz"=FALSE, "VoltCtrlRef"="", "TenHzFrequency"=0}  # App Config
  w86 = string[][] []  # Profile
  w87 = errorcluster {"status"=FALSE, "code"=0, "source"=""}  # Error
  # "There is no longer a reason to have CT Offsets but"
  # "***** NEW ******"
  # "|\n|\n|\n|\n|\n|\n|\n|\n|\n|\n|\n|\n|\n|"
  # "******************************************     O L D      ***************************************"
  # "PWM Period (Ticks) = 40,000,000 / PWM Period (Hz)\nPWM Period (Ticks) = 40,000,000 * PWM Period (sec)\nPWM Duty Cycle (Ticks) = PWM Period (Ticks) * PWM Duty Cycle (%) / 100\nPWM Duty Cycle (Ticks) = 40,000,000 * PWM Duty Cycle (sec)"
  # "Need a way to make sure I dont overflow the RIO\n\nNeed to create a way to split up a section of data to make data collected after middnight go to the next day\n\nneed to figure out how to deal with the SD card being removed and replaced"
  # "I think I can remove Voltage\nEnable from shift register"
  # "Need a way to verify that the AKLH files do not pile up and fill the RIO space"
  # "Timer Data 180"
  # "AI Data 1000"
  # "FPGA FIFO AI Data originally had 45 channels and asked for 10000 addresses reserved that would 222 possible full sets of data\nI would think 3 would be all that would be required 1 to find indexer, 1 to read, and 1 more in case RT is looping slightly faster than FPGA"
  # "I dont think I want to shut off voltage when the lower stop button is pressed"
  # "I believe PWM? in Controller Selection is useless once I have all the CAN selections initiated in the CAN loop"
  # "Remove PWM Freq (Hz) from app config and reference Frequency in Controller Selection"
  # "Do I have to put CA#, Requester(s), Start date... inside AKLH data file\nDo I have to include the profile on a second sheet\n\nwhen the controller type is non-controller brushed need to multiply controll current by zero... maybe\n\nLong-term would want to have a shutoff based on Cycles completed or all active pumps on time"
  # "Should change so that the PS, pres, and solenoid enable are\nnot stored in 2 places (app config and profile enables)"
  n1 = Bundle("Error"=w87, "Profile"=w86, "App Config"=w85, "Profiles"=w84, "Current Step"=w83, "Step Time Left"=w82, "Run Profile"=w81, "Step Start Time"=w80, "Step Time"=w79, "# of Steps"=w78, "Last Update"=w77, "Update Screen"=w76, "Last Profile Time"=w75, "Manual CMDs"=w74, "Client?"=w73, "pb.Run Profile"=w72, "pb.Resets"=w71, "pb.Sets"=w70, "Last CMDs"=w69, "Update Profile"=w68, "Elapsed Times"=w67, "Intitial Times"=w66, "Alarm"=w65, "CT Offsets"=w55, "Pumps Present"=w64, "Login"=w63, "Stagger Counter"=w62, "New Step"=w61, "Restarts Limits"=w60, "Restarts Cluster"=w59, "Actual Starts"=w58, "AKLH Path"=w54, "TenHz Path"=w53, "AKLH Timer"=w52, "TenHz Timer"=w51, "TenHz Active?"=w50, "AKLH Last Hour"=w49, "Main Tab"=w48, "Stop Cmd"=w47, "Tank Data"=w46, "CogCounters"=w44, "Cog Events"=w43, "Voltage Enable"=w42, "Cog Limits:"=w41, "TenHz Day"=w37, "Controller"=w23, "PS CMD"=w31, "Press CMD"=w30, "Temp CMD"=w29, "Power Relay"=w28, "Ignition Relay"=w27, "Controller List"=w22, "Alarm Config"=w21, "Alarm Config Path"=w20, "Trip Counters"=w19, "Previous Times"=w18, "Alarm Message"=w17, "Restart Alarm"=w16, "Pulse Frequency"=w15, "1 Pulse Duty%"=w14, "2 Pulse Duty%"=w13, "3 Pulse Duty%"=w12, "1 Pulsing"=w11, "Solenoid 1"=w10, "2 Pulsing"=w9, "Solenoid 2"=w8, "3 Pulsing"=w7, "Solenoid 3"=w6, "SubRoutine Profile"=w1, "Profile #"=w2, "ReqCycles"=w3, "Run Subs"=w4, "SR Step"=w5) -> (w57:T17)  [unwired: 1 in]
  n2 = flat-sequence {
    tunnel: [w88] -> w45
    tunnel: w32 -> [w88]
    frame #0 {
      n3 = Wait (ms)(milliseconds to wait=u32 5000) -> ()  [unwired: 1 out]
    }
  }
  n4 = xnode "Open FPGA VI Reference"("resource name"=tag "RIO0") -> ("FPGA VI Reference Out"=w32:refnum<k20>, "error out"=w36:errorcluster)  [unwired: 1 in]
  n5 = call "CAN Communication.vi"("CAN Mode"=CAN_Mode."Init") -> ("Error OUT"=w34:errorcluster)  [unwired: 10 in]
  n6 = Generate Occurrence() -> (w24:refnum<k4>)
  n7 = call "RPi HMI Com.vi"("RPi HMI Mode"=RPi_HMI_Mode."Init") -> ("HMI Cluster"=w25:T18)  [unwired: 18 in]
  n8 = disable-structure shown="Disabled" {
    disable-tunnel: w32 -> [w91 _]
    disable-tunnel: w24 -> [w90 _]
    frame Disabled {
      n9 = flat-sequence {
        tunnel: w90 -> [w97]
        tunnel: [w96] -> w95
        tunnel: w91 -> [w96]
        tunnel: [w101] -> w94
        tunnel: w95 -> [w101]
        tunnel: w94 -> [w107]
        tunnel: [w106] -> w93
        tunnel: [w109] -> w92
        tunnel: w93 -> [w109]
        tunnel: w92 -> [w112]
        frame #0 {
          n10 = Wait on Occurrence(2:w97) -> ()  [unwired: 2 in, 1 out]
        }
        frame #1 {
          n11 = call "AI RT FIFO.vi"("Mode"=RT_FIFO_Mode."Create", "Buffer Size"=1000, "# of elements"=54) -> ()  [unwired: 10 in, 3 out]
        }
        frame #2 {
          n12 = control-ref of="Stop"() -> (w104:refnum<vi>)
          n13 = property class="Bool (strict)"(reference=w104, "Value"=FALSE) -> (reference out=w103:refnum<vi>)  [unwired: 1 in, 1 out]
          n14 = call "Loop (DMA).vi"("Stop"=w103, "Sample Rate"=u32 10, "FPGA Ref"=w107) -> ("FPGA Ref OUT"=w106:T25)  [unwired: 7 in, 1 out]
          n15 = call "Loop (Data Stream).vi"("Stop"=w103) -> ()  [unwired: 10 in, 1 out]
        }
        frame #3 {
          n16 = call "AI RT FIFO.vi"("Mode"=RT_FIFO_Mode."Delete") -> ()  [unwired: 12 in, 3 out]
        }
        frame #4 {
          n17 = xnode "Invoke Method"("FPGA VI Reference In"=w112) -> ("FPGA VI Reference Out"=w110:T25, "error out"=w111:errorcluster)  [unwired: 1 in]
          n18 = xnode "Close FPGA VI Reference"("FPGA VI Reference In"=w110, "error in"=w111) -> ()  [unwired: 1 out]
        }
      }
    }
    frame Enabled {
    }
  }
  n19 = while {
    tunnel: w34 -> [w116]
    i -> [w113]
    stop <- FALSE stop-if-true
    n20 = local read "Controller Type:"() -> (w114:T5)
    n21 = local read "CAN CMD"() -> (w115:dbl)
    n22 = case shown="\"Kuhnke\", Default" w114 {
      tunnel: w116 -> [_ w121 w126 w130 w134]
      tunnel: w115 -> [_ w120 w128 w131 w132]
      tunnel: w113 -> [_ _ w125 _ _]
      frame "Kuhnke", Default {
        n23 = Wait (ms)(milliseconds to wait=u32 500) -> ()  [unwired: 1 out]
      }
      frame "Conti" {
        n24 = To Unsigned Word Integer(number=w120) -> (unsigned 16bit integer=w119:u16)
        n25 = call "Conti CAN.vi"("Error IN"=w121, "CMD"=w119) -> ()  [unwired: 9 in, 1 out]
      }
      frame "Helbako" {
        n26 = Quotient & Remainder(x=w125, y=10) -> (x-y*floor(x/y)=w123:i32)  [unwired: 1 out]
        n27 = To Unsigned Word Integer(number=w128) -> (unsigned 16bit integer=w127:u16)
        n28 = Equal To 0?(x=w123) -> (x = 0?=w122:bool)
        n29 = call "Helbako CAN.vi"("Split-timer"=w122, "Error IN"=w126, "CMD"=w127) -> ()  [unwired: 8 in, 1 out]
      }
      frame "Hella Gas" {
        n30 = To Unsigned Word Integer(number=w131) -> (unsigned 16bit integer=w129:u16)
        n31 = call "Hella CAN Gas.vi"("Pressure Command (kPa)"=w129, "Error In"=w130) -> ()  [unwired: 12 in, 2 out]
      }
      frame "Hella Diesel" {
        n32 = To Unsigned Word Integer(number=w132) -> (unsigned 16bit integer=w133:u16)
        n33 = call "Hella CAN Diesel.vi"("Command (kPa)"=w133, "Error In"=w134) -> ()  [unwired: 13 in, 1 out]
      }
    }
  }
  n34 = while {
    tunnel: w25 -> [_]
    tunnel: w24 -> [_]
    stop <- FALSE stop-if-true
    n35 = flat-sequence {
      frame #0 {
        n36 = call "RPi HMI Com.vi"("RPi HMI Mode"=RPi_HMI_Mode."Read from RPi") -> ("HMI Cluster"=w144:T18)  [unwired: 18 in]
        n37 = Unbundle By Name(w144) -> ("HMI Command"=w143:bool, "Power Relays"=w142:T2, "Pump CMDs"=w141:dbl[], "Tank CMDs.PS CMD"=w140:dbl, "Tank CMDs.Press CMD"=w139:dbl, "HMI Tog Buttons.Start Test"=w138:bool, "HMI Mom Buttons"=w137:T1)  [unwired: 1 out]
        n38 = case shown="True" w143 {
          tunnel: w142 -> [_ w151]
          tunnel: w141 -> [_ w150]
          tunnel: w140 -> [_ w149]
          tunnel: w139 -> [_ w148]
          tunnel: w138 -> [_ w147]
          tunnel: w137 -> [_ w146]
          frame False {
          }
          frame True {
            n39 = flat-sequence {
              tunnel: w151 -> [w157]
              tunnel: w150 -> [w156]
              tunnel: w149 -> [w155]
              tunnel: w148 -> [w154]
              tunnel: w147 -> [w153]
              tunnel: w146 -> [w152]
              frame #0 {
                n40 = local write "Power Relay"(w157) -> ()
                n41 = local write "Manual\nCMD"(w156) -> ()
                n42 = local write "Power Supply Cmd (V):"(w155) -> ()
                n43 = local write "PressureCMD"(w154) -> ()
                n44 = local write "pb.Run Profile"(w153) -> ()
                "HMI Mom Buttons" <- w152
              }
              frame #1 {
                n45 = Wait (ms)(milliseconds to wait=u32 20) -> ()  [unwired: 1 out]
              }
            }
          }
        }
      }
      frame #1 {
        n46 = call "RPi HMI Com.vi"("RPi HMI Mode"=RPi_HMI_Mode."Write to RPi") -> ()  [unwired: 18 in, 1 out]
      }
    }
    n47 = Wait (ms)(milliseconds to wait=u32 80) -> ()  [unwired: 1 out]
  }
  n48 = while {
    shift-right: [w169] -> _
    shift-left: w56 -> [w167]
    shift-right: [w170] -> _
    shift-left: w57 -> [w171]
    tunnel: w32 -> [w168]
    tunnel: w24 -> [w160]
    tunnel: w36 -> [_]
    stop <- FALSE stop-if-true
    n49 = Delete From Array(array=w167, length=1, index=0 ("length")) -> (deleted portion=w163:T14[], array with subset deleted=w166:T14[])
    n50 = Wait (ms)(milliseconds to wait=u32 20) -> ()  [unwired: 1 out]
    n51 = Index Array(array=w163) -> (element=w162:T14)  [unwired: 1 in]
    n52 = case shown="\"Save Status\"" w162 {
      selector: w162 -> [_ _ _ _ _ _ _ _ _ _ _ _ _ _ _ _ _ _ w1322 _ _ _ _ _ _ _ _ _ _ _ _ _ _ _]
      tunnel: [w204 w661 w791 w854 w874 w894 w902 w918 w933 w953 w976 w1020 w1097 w1210 w1239 w1261 w1312 w1321 w1333 w1401 w1449 w1470 w1525 w1569 w1588 w1627 w1732 w1741 w1756 w1835 w1871 w1884 w1945 w1972] -> w170
      tunnel: w171 -> [w201 w662 w789 w855 w875 w894 w903 w919 w934 w954 w977 w1021 w1167 w1199 w1240 w1262 w1312 w1321 w1323 w1402 w1448 w1467 w1525 w1569 w1589 w1628 w1733 w1741 w1757 w1819 w1871 w1885 w1946 w1973]
      tunnel: [w190 w684 w795 w850 w878 w895 w896 w907 w932 w947 w974 w1003 w1165 w1204 w1241 w1293 w1311 w1317 w1324 w1418 w1438 w1468 w1529 w1567 w1591 w1620 w1720 w1740 w1755 w1834 w1870 w1889 w1941 w1968] -> w169
      tunnel: w168 -> [_ _ w793 _ _ _ _ _ _ _ _ w1011 w1100 w1208 _ _ _ w1320 w1327 _ w1441 w1469 w1519 _ _ _ _ _ _ w1798 _ w1886 _ _]
      tunnel: w166 -> [_ w684 _ w849 w878 w895 w897 w908 _ _ _ w1004 w1164 w1206 _ w1293 w1311 w1318 _ _ _ w1468 w1529 w1567 w1591 w1621 w1721 w1740 w1755 w1834 w1870 w1889 w1941 w1968]
      tunnel: w160 -> [_ _ w779 _ _ _ _ _ _ _ _ _ _ _ _ _ _ _ _ _ _ _ _ _ _ _ _ _ _ _ _ _ _ _]
      frame "Main", Default {
        # "Any Latch when released boolean buttons do not need to be stored\nin the shift register they had been stored and looked at if they were\ngreater than the past value stored in the shift register"
        n53 = Unbundle By Name(w201) -> ("Run Profile"=w199:bool, "Last Update"=w203:dbl, "TenHz Timer"=w187:dbl, "AKLH Timer"=w186:dbl, "App Config.Record TenHz"=w178:bool, "TenHz Day"=w177:i32)
        n54 = for {
          N: 53 -> [_]
          shift-right: [w219] -> w202
          shift-left: w201 -> [w218]
          tunnel: [w217] -> w198
          tunnel: [w216] -> w200
          i -> [w220]
          stop <- w216 stop-if-true
          n55 = case shown="43" w220 {
            tunnel: w218 -> [w227 w234 w236 w244 w247 w249 w257 w264 w272 w279 w286 w294 w297 w305 w312 w319 w326 w327 w333 w334 w344 w351 w358 w360 w369 w370 w374 w377 w384 w391 w398 w406 w414 w416 w420 w512 w518 w526 w530 w539 w549 w558 w565 w572 w579 w586 w593 w600 w607 w614 w621 w626 w639]
            tunnel: [w226 w233 w236 w243 w247 w249 w256 w263 w271 w278 w285 w293 w297 w304 w311 w318 w325 w327 w333 w334 w343 w350 w357 w360 w368 w370 w374 w377 w383 w390 w397 w405 w413 w416 w421 w511 w517 w525 w529 w539 w548 w557 w564 w571 w578 w585 w592 w599 w606 w613 w620 w625 w638] -> w219
            tunnel: [w223 "pb.E Stop" "pb.Save As" w242 "pb.Stop Profile" "pb.Cycle Reset" w255 w262 w268 w275 w282 w287 "pb.Zero CMDs" w301 w308 w315 w322 "pb.Reset Restarts" w331 "pb.Time Reset All" w342 w349 w356 "pb.Rst Tot Restarts" w365 "pb.FuelChange" FALSE ("Restarts Alarm") FALSE ("Restarts Alarm") w379 w388 w393 w403 w409 "pb.Reset Cogs" w419 w509 w514 w522 w532 w535 w551 w556 w563 w570 w577 w584 w591 w598 w605 w612 w619 w631 w643] -> w216
            tunnel: w218 -> [w225 w232 _ w241 _ _ w254 w261 w270 w277 w284 w292 _ w303 w310 w317 w324 _ w332 _ w341 w348 w355 _ w367 _ _ _ w382 w389 w396 w407 w415 _ w423 w510 w519 w524 w531 _ w550 w559 w566 w573 w580 w587 w594 w601 w608 w615 w622 w627 w640]
            tunnel: [w222 w235 w237 w239 w248 w251 w252 w259 w267 w273 w280 w290 w298 w299 w307 w314 w321 w329 w330 w336 w340 w347 w354 w362 w364 w372 w373 w376 w385 w392 w399 w400 w408 w418 w425 w506 w513 w523 w533 w540 w552 w553 w561 w568 w575 w582 w589 w596 w603 w610 w617 w630 w637] -> w217
            frame 0, Default {
              w222 = T14[] [enum."Set Manual CMD"] items=["Main", "Init Files", "Init", "Save As", "Start Profile", "Check Step Time", "Alarm", "Run Step", "Stop Profile", "Cycle Reset", "Time Reset", "Time Reset All", "Time Set", "Tare CTs", "Save Profile", "Open Profile", "Get Profiles", "Update Screen", "Save Status", "Set Manual CMD", "Reset Restarts", "Reset Total Restarts", "Reset Cogs", "Disable Background", "Enable Background", "Get/Release Control", "Init AKLH", "Save AKLH", "Log Fuel Change", "Update Data Stream", "Init TenHz", "Read TenHz", "Remote Timer Reset", "Record Frequency Change", "Controller Change", "Get Alarms", "Init Alarms", "Save Alarms", "Init SubRoutine", "Next SubRoutine"]
              n56 = Unbundle By Name(w225) -> ("PS CMD"=w224:dbl)
              n57 = Not Equal?(x=w224, y="Power Supply Cmd (V):") -> (x != y?=w223:bool)
              n58 = Bundle By Name(cluster=w227, "PS CMD"="Power Supply Cmd (V):") -> (w226:T17)
            }
            frame 1 {
              w235 = T14[] [enum."Set Manual CMD"] items=["Main", "Init Files", "Init", "Save As", "Start Profile", "Check Step Time", "Alarm", "Run Step", "Stop Profile", "Cycle Reset", "Time Reset", "Time Reset All", "Time Set", "Tare CTs", "Save Profile", "Open Profile", "Get Profiles", "Update Screen", "Save Status", "Set Manual CMD", "Reset Restarts", "Reset Total Restarts", "Reset Cogs", "Disable Background", "Enable Background", "Get/Release Control", "Init AKLH", "Save AKLH", "Log Fuel Change", "Update Data Stream", "Init TenHz", "Read TenHz", "Remote Timer Reset", "Record Frequency Change", "Controller Change", "Get Alarms", "Init Alarms", "Save Alarms", "Init SubRoutine", "Next SubRoutine"]
              n59 = Unbundle By Name(w232) -> ("PS CMD"=w231:dbl)
              n60 = Select(t=0.0, s="pb.E Stop", f=w231) -> (s? t:f=w229:dbl)
              n61 = local write "Power Supply Cmd (V):"(w229) -> ()
              n62 = Bundle By Name(cluster=w234, "PS CMD"=w229, "Voltage Enable"="pb.E Stop") -> (w233:T17)
            }
            frame 2 {
              w237 = T14[] [enum."Disable Background", enum."Save As"] items=["Main", "Init Files", "Init", "Save As", "Start Profile", "Check Step Time", "Alarm", "Run Step", "Stop Profile", "Cycle Reset", "Time Reset", "Time Reset All", "Time Set", "Tare CTs", "Save Profile", "Open Profile", "Get Profiles", "Update Screen", "Save Status", "Set Manual CMD", "Reset Restarts", "Reset Total Restarts", "Reset Cogs", "Disable Background", "Enable Background", "Get/Release Control", "Init AKLH", "Save AKLH", "Log Fuel Change", "Update Data Stream", "Init TenHz", "Read TenHz", "Remote Timer Reset", "Record Frequency Change", "Controller Change", "Get Alarms", "Init Alarms", "Save Alarms", "Init SubRoutine", "Next SubRoutine"]
            }
            frame 3 {
              w239 = T14[] [enum."Start Profile"] items=["Main", "Init Files", "Init", "Save As", "Start Profile", "Check Step Time", "Alarm", "Run Step", "Stop Profile", "Cycle Reset", "Time Reset", "Time Reset All", "Time Set", "Tare CTs", "Save Profile", "Open Profile", "Get Profiles", "Update Screen", "Save Status", "Set Manual CMD", "Reset Restarts", "Reset Total Restarts", "Reset Cogs", "Disable Background", "Enable Background", "Get/Release Control", "Init AKLH", "Save AKLH", "Log Fuel Change", "Update Data Stream", "Init TenHz", "Read TenHz", "Remote Timer Reset", "Record Frequency Change", "Controller Change", "Get Alarms", "Init Alarms", "Save Alarms", "Init SubRoutine", "Next SubRoutine"]
              n63 = Unbundle By Name(w241) -> ("pb.Run Profile"=w245:bool)
              n64 = Greater?(x="pb.Run Profile", y=w245) -> (0:w242:bool)
              n65 = Bundle By Name(cluster=w244, "pb.Run Profile"="pb.Run Profile") -> (w243:T17)
            }
            frame 4 {
              w248 = T14[] [enum."Stop Profile"] items=["Main", "Init Files", "Init", "Save As", "Start Profile", "Check Step Time", "Alarm", "Run Step", "Stop Profile", "Cycle Reset", "Time Reset", "Time Reset All", "Time Set", "Tare CTs", "Save Profile", "Open Profile", "Get Profiles", "Update Screen", "Save Status", "Set Manual CMD", "Reset Restarts", "Reset Total Restarts", "Reset Cogs", "Disable Background", "Enable Background", "Get/Release Control", "Init AKLH", "Save AKLH", "Log Fuel Change", "Update Data Stream", "Init TenHz", "Read TenHz", "Remote Timer Reset", "Record Frequency Change", "Controller Change", "Get Alarms", "Init Alarms", "Save Alarms", "Init SubRoutine", "Next SubRoutine"]
            }
            frame 5 {
              w251 = T14[] [enum."Disable Background", enum."Cycle Reset"] items=["Main", "Init Files", "Init", "Save As", "Start Profile", "Check Step Time", "Alarm", "Run Step", "Stop Profile", "Cycle Reset", "Time Reset", "Time Reset All", "Time Set", "Tare CTs", "Save Profile", "Open Profile", "Get Profiles", "Update Screen", "Save Status", "Set Manual CMD", "Reset Restarts", "Reset Total Restarts", "Reset Cogs", "Disable Background", "Enable Background", "Get/Release Control", "Init AKLH", "Save AKLH", "Log Fuel Change", "Update Data Stream", "Init TenHz", "Read TenHz", "Remote Timer Reset", "Record Frequency Change", "Controller Change", "Get Alarms", "Init Alarms", "Save Alarms", "Init SubRoutine", "Next SubRoutine"]
            }
            frame 6 {
              w252 = T14[] [enum."Disable Background", enum."Time Reset"] items=["Main", "Init Files", "Init", "Save As", "Start Profile", "Check Step Time", "Alarm", "Run Step", "Stop Profile", "Cycle Reset", "Time Reset", "Time Reset All", "Time Set", "Tare CTs", "Save Profile", "Open Profile", "Get Profiles", "Update Screen", "Save Status", "Set Manual CMD", "Reset Restarts", "Reset Total Restarts", "Reset Cogs", "Disable Background", "Enable Background", "Get/Release Control", "Init AKLH", "Save AKLH", "Log Fuel Change", "Update Data Stream", "Init TenHz", "Read TenHz", "Remote Timer Reset", "Record Frequency Change", "Controller Change", "Get Alarms", "Init Alarms", "Save Alarms", "Init SubRoutine", "Next SubRoutine"]
              n66 = Unbundle By Name(w254) -> ("pb.Resets"=w258:bool[])
              n67 = Greater?(x="pb.Resets", y=w258) -> (0:w255:bool)
              n68 = Bundle By Name(cluster=w257, "pb.Resets"="pb.Resets") -> (w256:T17)
            }
            frame 7 {
              w259 = T14[] [enum."Disable Background", enum."Time Set"] items=["Main", "Init Files", "Init", "Save As", "Start Profile", "Check Step Time", "Alarm", "Run Step", "Stop Profile", "Cycle Reset", "Time Reset", "Time Reset All", "Time Set", "Tare CTs", "Save Profile", "Open Profile", "Get Profiles", "Update Screen", "Save Status", "Set Manual CMD", "Reset Restarts", "Reset Total Restarts", "Reset Cogs", "Disable Background", "Enable Background", "Get/Release Control", "Init AKLH", "Save AKLH", "Log Fuel Change", "Update Data Stream", "Init TenHz", "Read TenHz", "Remote Timer Reset", "Record Frequency Change", "Controller Change", "Get Alarms", "Init Alarms", "Save Alarms", "Init SubRoutine", "Next SubRoutine"]
              n69 = Unbundle By Name(w261) -> ("pb.Sets"=w265:bool[])
              n70 = Greater?(x="pb.Sets", y=w265) -> (0:w262:bool)
              n71 = Bundle By Name(cluster=w264, "pb.Sets"="pb.Sets") -> (w263:T17)
            }
            frame 8 {
              w267 = T14[] [enum."Save Profile"] items=["Main", "Init Files", "Init", "Save As", "Start Profile", "Check Step Time", "Alarm", "Run Step", "Stop Profile", "Cycle Reset", "Time Reset", "Time Reset All", "Time Set", "Tare CTs", "Save Profile", "Open Profile", "Get Profiles", "Update Screen", "Save Status", "Set Manual CMD", "Reset Restarts", "Reset Total Restarts", "Reset Cogs", "Disable Background", "Enable Background", "Get/Release Control", "Init AKLH", "Save AKLH", "Log Fuel Change", "Update Data Stream", "Init TenHz", "Read TenHz", "Remote Timer Reset", "Record Frequency Change", "Controller Change", "Get Alarms", "Init Alarms", "Save Alarms", "Init SubRoutine", "Next SubRoutine"]
              n72 = Unbundle By Name(w270) -> ("Profile"=w269:string[][])
              n73 = Not Equal?(x=w269, y="Profile:") -> (x != y?=w268:bool)
              n74 = Bundle By Name(cluster=w272, "Profile"="Profile:") -> (w271:T17)
            }
            frame 9 {
              w273 = T14[] [enum."Open Profile"] items=["Main", "Init Files", "Init", "Save As", "Start Profile", "Check Step Time", "Alarm", "Run Step", "Stop Profile", "Cycle Reset", "Time Reset", "Time Reset All", "Time Set", "Tare CTs", "Save Profile", "Open Profile", "Get Profiles", "Update Screen", "Save Status", "Set Manual CMD", "Reset Restarts", "Reset Total Restarts", "Reset Cogs", "Disable Background", "Enable Background", "Get/Release Control", "Init AKLH", "Save AKLH", "Log Fuel Change", "Update Data Stream", "Init TenHz", "Read TenHz", "Remote Timer Reset", "Record Frequency Change", "Controller Change", "Get Alarms", "Init Alarms", "Save Alarms", "Init SubRoutine", "Next SubRoutine"]
              n75 = Unbundle By Name(w277) -> ("App Config.Current Profile"=w276:string)
              n76 = Not Equal?(x=w276, y="Profile Name:") -> (x != y?=w275:bool)
              n77 = Bundle By Name(cluster=w279, "App Config.Current Profile"="Profile Name:") -> (w278:T17)
            }
            frame 10 {
              w280 = T14[] [enum."Set Manual CMD"] items=["Main", "Init Files", "Init", "Save As", "Start Profile", "Check Step Time", "Alarm", "Run Step", "Stop Profile", "Cycle Reset", "Time Reset", "Time Reset All", "Time Set", "Tare CTs", "Save Profile", "Open Profile", "Get Profiles", "Update Screen", "Save Status", "Set Manual CMD", "Reset Restarts", "Reset Total Restarts", "Reset Cogs", "Disable Background", "Enable Background", "Get/Release Control", "Init AKLH", "Save AKLH", "Log Fuel Change", "Update Data Stream", "Init TenHz", "Read TenHz", "Remote Timer Reset", "Record Frequency Change", "Controller Change", "Get Alarms", "Init Alarms", "Save Alarms", "Init SubRoutine", "Next SubRoutine"]
              n78 = Unbundle By Name(w284) -> ("Manual CMDs"=w283:dbl[])
              n79 = Not Equal?(x=w283, y="Manual\nCMD") -> (x != y?=w282:bool)
              n80 = Bundle By Name(cluster=w286, "Manual CMDs"="Manual\nCMD") -> (w285:T17)
            }
            frame 11 {
              w290 = T14[] [enum."Get/Release Control"] items=["Main", "Init Files", "Init", "Save As", "Start Profile", "Check Step Time", "Alarm", "Run Step", "Stop Profile", "Cycle Reset", "Time Reset", "Time Reset All", "Time Set", "Tare CTs", "Save Profile", "Open Profile", "Get Profiles", "Update Screen", "Save Status", "Set Manual CMD", "Reset Restarts", "Reset Total Restarts", "Reset Cogs", "Disable Background", "Enable Background", "Get/Release Control", "Init AKLH", "Save AKLH", "Log Fuel Change", "Update Data Stream", "Init TenHz", "Read TenHz", "Remote Timer Reset", "Record Frequency Change", "Controller Change", "Get Alarms", "Init Alarms", "Save Alarms", "Init SubRoutine", "Next SubRoutine"]
              n81 = Unbundle By Name(w292) -> ("Client?"=w288:bool, "Profiles"=w291:string[])
              n82 = local read "Client?"() -> (w289:bool)
              n83 = Greater?(x=w289, y=w288) -> (0:w287:bool)
              n84 = case shown="True" w287 {
                tunnel: w291 -> [_ w295]
                frame False {
                }
                frame True {
                  n85 = property on="Profile Name:" class="CmbBox"("Strings[]"=w295) -> ()  [unwired: 2 in, 2 out]
                }
              }
              n86 = Bundle By Name(cluster=w294, "Client?"=w289) -> (w293:T17)
            }
            frame 12 {
              w298 = T14[] [enum."Stop Profile"] items=["Main", "Init Files", "Init", "Save As", "Start Profile", "Check Step Time", "Alarm", "Run Step", "Stop Profile", "Cycle Reset", "Time Reset", "Time Reset All", "Time Set", "Tare CTs", "Save Profile", "Open Profile", "Get Profiles", "Update Screen", "Save Status", "Set Manual CMD", "Reset Restarts", "Reset Total Restarts", "Reset Cogs", "Disable Background", "Enable Background", "Get/Release Control", "Init AKLH", "Save AKLH", "Log Fuel Change", "Update Data Stream", "Init TenHz", "Read TenHz", "Remote Timer Reset", "Record Frequency Change", "Controller Change", "Get Alarms", "Init Alarms", "Save Alarms", "Init SubRoutine", "Next SubRoutine"]
            }
            frame 13 {
              w299 = T14[] [enum."Save Status"] items=["Main", "Init Files", "Init", "Save As", "Start Profile", "Check Step Time", "Alarm", "Run Step", "Stop Profile", "Cycle Reset", "Time Reset", "Time Reset All", "Time Set", "Tare CTs", "Save Profile", "Open Profile", "Get Profiles", "Update Screen", "Save Status", "Set Manual CMD", "Reset Restarts", "Reset Total Restarts", "Reset Cogs", "Disable Background", "Enable Background", "Get/Release Control", "Init AKLH", "Save AKLH", "Log Fuel Change", "Update Data Stream", "Init TenHz", "Read TenHz", "Remote Timer Reset", "Record Frequency Change", "Controller Change", "Get Alarms", "Init Alarms", "Save Alarms", "Init SubRoutine", "Next SubRoutine"]
              n87 = Unbundle By Name(w303) -> ("App Config.CA Number"=w302:string)
              n88 = Not Equal?(x=w302, y="CA Number:") -> (x != y?=w301:bool)
              n89 = Bundle By Name(cluster=w305, "App Config.CA Number"="CA Number:") -> (w304:T17)
            }
            frame 14 {
              w307 = T14[] [enum."Save Status", enum."Controller Change"] items=["Main", "Init Files", "Init", "Save As", "Start Profile", "Check Step Time", "Alarm", "Run Step", "Stop Profile", "Cycle Reset", "Time Reset", "Time Reset All", "Time Set", "Tare CTs", "Save Profile", "Open Profile", "Get Profiles", "Update Screen", "Save Status", "Set Manual CMD", "Reset Restarts", "Reset Total Restarts", "Reset Cogs", "Disable Background", "Enable Background", "Get/Release Control", "Init AKLH", "Save AKLH", "Log Fuel Change", "Update Data Stream", "Init TenHz", "Read TenHz", "Remote Timer Reset", "Record Frequency Change", "Controller Change", "Get Alarms", "Init Alarms", "Save Alarms", "Init SubRoutine", "Next SubRoutine"]
              n90 = Unbundle By Name(w310) -> ("App Config.Controller Type:"=w309:T5)
              n91 = Not Equal?(x=w309, y="Controller Type:") -> (x != y?=w308:bool)
              n92 = Bundle By Name(cluster=w312, "App Config.Controller Type:"="Controller Type:") -> (w311:T17)
            }
            frame 15 {
              w314 = T14[] [enum."Save Status"] items=["Main", "Init Files", "Init", "Save As", "Start Profile", "Check Step Time", "Alarm", "Run Step", "Stop Profile", "Cycle Reset", "Time Reset", "Time Reset All", "Time Set", "Tare CTs", "Save Profile", "Open Profile", "Get Profiles", "Update Screen", "Save Status", "Set Manual CMD", "Reset Restarts", "Reset Total Restarts", "Reset Cogs", "Disable Background", "Enable Background", "Get/Release Control", "Init AKLH", "Save AKLH", "Log Fuel Change", "Update Data Stream", "Init TenHz", "Read TenHz", "Remote Timer Reset", "Record Frequency Change", "Controller Change", "Get Alarms", "Init Alarms", "Save Alarms", "Init SubRoutine", "Next SubRoutine"]
              n93 = Unbundle By Name(w317) -> ("Restarts Limits"=w316:T3)
              n94 = Not Equal?(x=w316, y="Restarts Limits") -> (x != y?=w315:bool)
              n95 = Bundle By Name(cluster=w319, "Restarts Limits"="Restarts Limits") -> (w318:T17)
            }
            frame 16 {
              w321 = T14[] [enum."Save Status"] items=["Main", "Init Files", "Init", "Save As", "Start Profile", "Check Step Time", "Alarm", "Run Step", "Stop Profile", "Cycle Reset", "Time Reset", "Time Reset All", "Time Set", "Tare CTs", "Save Profile", "Open Profile", "Get Profiles", "Update Screen", "Save Status", "Set Manual CMD", "Reset Restarts", "Reset Total Restarts", "Reset Cogs", "Disable Background", "Enable Background", "Get/Release Control", "Init AKLH", "Save AKLH", "Log Fuel Change", "Update Data Stream", "Init TenHz", "Read TenHz", "Remote Timer Reset", "Record Frequency Change", "Controller Change", "Get Alarms", "Init Alarms", "Save Alarms", "Init SubRoutine", "Next SubRoutine"]
              n96 = Unbundle By Name(w324) -> ("App Config.Inform"=w323:string)
              n97 = Not Equal?(x=w323, y="Inform:") -> (x != y?=w322:bool)
              n98 = Bundle By Name(cluster=w326, "App Config.Inform"="Inform:") -> (w325:T17)
            }
            frame 17 {
              w329 = T14[] [enum."Disable Background", enum."Reset Restarts"] items=["Main", "Init Files", "Init", "Save As", "Start Profile", "Check Step Time", "Alarm", "Run Step", "Stop Profile", "Cycle Reset", "Time Reset", "Time Reset All", "Time Set", "Tare CTs", "Save Profile", "Open Profile", "Get Profiles", "Update Screen", "Save Status", "Set Manual CMD", "Reset Restarts", "Reset Total Restarts", "Reset Cogs", "Disable Background", "Enable Background", "Get/Release Control", "Init AKLH", "Save AKLH", "Log Fuel Change", "Update Data Stream", "Init TenHz", "Read TenHz", "Remote Timer Reset", "Record Frequency Change", "Controller Change", "Get Alarms", "Init Alarms", "Save Alarms", "Init SubRoutine", "Next SubRoutine"]
            }
            frame 18 {
              w330 = T14[] [enum."Stop Profile", enum."Disable Background", enum."Alarm"] items=["Main", "Init Files", "Init", "Save As", "Start Profile", "Check Step Time", "Alarm", "Run Step", "Stop Profile", "Cycle Reset", "Time Reset", "Time Reset All", "Time Set", "Tare CTs", "Save Profile", "Open Profile", "Get Profiles", "Update Screen", "Save Status", "Set Manual CMD", "Reset Restarts", "Reset Total Restarts", "Reset Cogs", "Disable Background", "Enable Background", "Get/Release Control", "Init AKLH", "Save AKLH", "Log Fuel Change", "Update Data Stream", "Init TenHz", "Read TenHz", "Remote Timer Reset", "Record Frequency Change", "Controller Change", "Get Alarms", "Init Alarms", "Save Alarms", "Init SubRoutine", "Next SubRoutine"]
              n99 = Unbundle By Name(w332) -> ("Alarm"=w331:bool)
            }
            frame 19 {
              w336 = T14[] [enum."Disable Background", enum."Time Reset All"] items=["Main", "Init Files", "Init", "Save As", "Start Profile", "Check Step Time", "Alarm", "Run Step", "Stop Profile", "Cycle Reset", "Time Reset", "Time Reset All", "Time Set", "Tare CTs", "Save Profile", "Open Profile", "Get Profiles", "Update Screen", "Save Status", "Set Manual CMD", "Reset Restarts", "Reset Total Restarts", "Reset Cogs", "Disable Background", "Enable Background", "Get/Release Control", "Init AKLH", "Save AKLH", "Log Fuel Change", "Update Data Stream", "Init TenHz", "Read TenHz", "Remote Timer Reset", "Record Frequency Change", "Controller Change", "Get Alarms", "Init Alarms", "Save Alarms", "Init SubRoutine", "Next SubRoutine"]
            }
            frame 20 {
              w340 = T14[] [enum."Save Status"] items=["Main", "Init Files", "Init", "Save As", "Start Profile", "Check Step Time", "Alarm", "Run Step", "Stop Profile", "Cycle Reset", "Time Reset", "Time Reset All", "Time Set", "Tare CTs", "Save Profile", "Open Profile", "Get Profiles", "Update Screen", "Save Status", "Set Manual CMD", "Reset Restarts", "Reset Total Restarts", "Reset Cogs", "Disable Background", "Enable Background", "Get/Release Control", "Init AKLH", "Save AKLH", "Log Fuel Change", "Update Data Stream", "Init TenHz", "Read TenHz", "Remote Timer Reset", "Record Frequency Change", "Controller Change", "Get Alarms", "Init Alarms", "Save Alarms", "Init SubRoutine", "Next SubRoutine"]
              n100 = Unbundle By Name(w341) -> ("App Config.Pumps Present"=w345:u32)
              n101 = Cluster To Array(cluster="Pumps Present") -> (array=w339:bool[])
              n102 = Boolean Array To Number(Boolean array=w339) -> (number=w337:u32)
              n103 = Not Equal?(x=w337, y=w345) -> (x != y?=w342:bool)
              n104 = Bundle By Name(cluster=w344, "App Config.Pumps Present"=w337) -> (w343:T17)
            }
            frame 21 {
              w347 = T14[] [enum."Get/Release Control"] items=["Main", "Init Files", "Init", "Save As", "Start Profile", "Check Step Time", "Alarm", "Run Step", "Stop Profile", "Cycle Reset", "Time Reset", "Time Reset All", "Time Set", "Tare CTs", "Save Profile", "Open Profile", "Get Profiles", "Update Screen", "Save Status", "Set Manual CMD", "Reset Restarts", "Reset Total Restarts", "Reset Cogs", "Disable Background", "Enable Background", "Get/Release Control", "Init AKLH", "Save AKLH", "Log Fuel Change", "Update Data Stream", "Init TenHz", "Read TenHz", "Remote Timer Reset", "Record Frequency Change", "Controller Change", "Get Alarms", "Init Alarms", "Save Alarms", "Init SubRoutine", "Next SubRoutine"]
              n105 = Unbundle By Name(w348) -> ("Login"=w352:bool)
              n106 = Not Equal?(x="Login", y=w352) -> (x != y?=w349:bool)
              n107 = Bundle By Name(cluster=w351, "Login"="Login") -> (w350:T17)
            }
            frame 22 {
              w354 = T14[] [enum."Save Status"] items=["Main", "Init Files", "Init", "Save As", "Start Profile", "Check Step Time", "Alarm", "Run Step", "Stop Profile", "Cycle Reset", "Time Reset", "Time Reset All", "Time Set", "Tare CTs", "Save Profile", "Open Profile", "Get Profiles", "Update Screen", "Save Status", "Set Manual CMD", "Reset Restarts", "Reset Total Restarts", "Reset Cogs", "Disable Background", "Enable Background", "Get/Release Control", "Init AKLH", "Save AKLH", "Log Fuel Change", "Update Data Stream", "Init TenHz", "Read TenHz", "Remote Timer Reset", "Record Frequency Change", "Controller Change", "Get Alarms", "Init Alarms", "Save Alarms", "Init SubRoutine", "Next SubRoutine"]
              n108 = Unbundle By Name(w355) -> ("App Config.Stagger Time (ms)"=w359:i32)
              n109 = Not Equal?(x="Stagger Time (ms):", y=w359) -> (x != y?=w356:bool)
              n110 = Bundle By Name(cluster=w358, "App Config.Stagger Time (ms)"="Stagger Time (ms):") -> (w357:T17)
            }
            frame 23 {
              w362 = T14[] [enum."Disable Background", enum."Reset Total Restarts"] items=["Main", "Init Files", "Init", "Save As", "Start Profile", "Check Step Time", "Alarm", "Run Step", "Stop Profile", "Cycle Reset", "Time Reset", "Time Reset All", "Time Set", "Tare CTs", "Save Profile", "Open Profile", "Get Profiles", "Update Screen", "Save Status", "Set Manual CMD", "Reset Restarts", "Reset Total Restarts", "Reset Cogs", "Disable Background", "Enable Background", "Get/Release Control", "Init AKLH", "Save AKLH", "Log Fuel Change", "Update Data Stream", "Init TenHz", "Read TenHz", "Remote Timer Reset", "Record Frequency Change", "Controller Change", "Get Alarms", "Init Alarms", "Save Alarms", "Init SubRoutine", "Next SubRoutine"]
            }
            frame 24 {
              w364 = T14[] [enum."Set Manual CMD"] items=["Main", "Init Files", "Init", "Save As", "Start Profile", "Check Step Time", "Alarm", "Run Step", "Stop Profile", "Cycle Reset", "Time Reset", "Time Reset All", "Time Set", "Tare CTs", "Save Profile", "Open Profile", "Get Profiles", "Update Screen", "Save Status", "Set Manual CMD", "Reset Restarts", "Reset Total Restarts", "Reset Cogs", "Disable Background", "Enable Background", "Get/Release Control", "Init AKLH", "Save AKLH", "Log Fuel Change", "Update Data Stream", "Init TenHz", "Read TenHz", "Remote Timer Reset", "Record Frequency Change", "Controller Change", "Get Alarms", "Init Alarms", "Save Alarms", "Init SubRoutine", "Next SubRoutine"]
              n111 = Unbundle By Name(w367) -> ("Press CMD"=w366:dbl)
              n112 = Not Equal?(x=w366, y="PressureCMD") -> (x != y?=w365:bool)
              n113 = Bundle By Name(cluster=w369, "Press CMD"="PressureCMD") -> (w368:T17)
            }
            frame 25 {
              w372 = T14[] [enum."Log Fuel Change"] items=["Main", "Init Files", "Init", "Save As", "Start Profile", "Check Step Time", "Alarm", "Run Step", "Stop Profile", "Cycle Reset", "Time Reset", "Time Reset All", "Time Set", "Tare CTs", "Save Profile", "Open Profile", "Get Profiles", "Update Screen", "Save Status", "Set Manual CMD", "Reset Restarts", "Reset Total Restarts", "Reset Cogs", "Disable Background", "Enable Background", "Get/Release Control", "Init AKLH", "Save AKLH", "Log Fuel Change", "Update Data Stream", "Init TenHz", "Read TenHz", "Remote Timer Reset", "Record Frequency Change", "Controller Change", "Get Alarms", "Init Alarms", "Save Alarms", "Init SubRoutine", "Next SubRoutine"]
            }
            frame 26 {
              w373 = T14[] [] items=["Main", "Init Files", "Init", "Save As", "Start Profile", "Check Step Time", "Alarm", "Run Step", "Stop Profile", "Cycle Reset", "Time Reset", "Time Reset All", "Time Set", "Tare CTs", "Save Profile", "Open Profile", "Get Profiles", "Update Screen", "Save Status", "Set Manual CMD", "Reset Restarts", "Reset Total Restarts", "Reset Cogs", "Disable Background", "Enable Background", "Get/Release Control", "Init AKLH", "Save AKLH", "Log Fuel Change", "Update Data Stream", "Init TenHz", "Read TenHz", "Remote Timer Reset", "Record Frequency Change", "Controller Change", "Get Alarms", "Init Alarms", "Save Alarms", "Init SubRoutine", "Next SubRoutine"]
            }
            frame 27 {
              w376 = T14[] [] items=["Main", "Init Files", "Init", "Save As", "Start Profile", "Check Step Time", "Alarm", "Run Step", "Stop Profile", "Cycle Reset", "Time Reset", "Time Reset All", "Time Set", "Tare CTs", "Save Profile", "Open Profile", "Get Profiles", "Update Screen", "Save Status", "Set Manual CMD", "Reset Restarts", "Reset Total Restarts", "Reset Cogs", "Disable Background", "Enable Background", "Get/Release Control", "Init AKLH", "Save AKLH", "Log Fuel Change", "Update Data Stream", "Init TenHz", "Read TenHz", "Remote Timer Reset", "Record Frequency Change", "Controller Change", "Get Alarms", "Init Alarms", "Save Alarms", "Init SubRoutine", "Next SubRoutine"]
            }
            frame 28 {
              w385 = T14[] [enum."Save Status"] items=["Main", "Init Files", "Init", "Save As", "Start Profile", "Check Step Time", "Alarm", "Run Step", "Stop Profile", "Cycle Reset", "Time Reset", "Time Reset All", "Time Set", "Tare CTs", "Save Profile", "Open Profile", "Get Profiles", "Update Screen", "Save Status", "Set Manual CMD", "Reset Restarts", "Reset Total Restarts", "Reset Cogs", "Disable Background", "Enable Background", "Get/Release Control", "Init AKLH", "Save AKLH", "Log Fuel Change", "Update Data Stream", "Init TenHz", "Read TenHz", "Remote Timer Reset", "Record Frequency Change", "Controller Change", "Get Alarms", "Init Alarms", "Save Alarms", "Init SubRoutine", "Next SubRoutine"]
              n114 = Unbundle By Name(w382) -> ("App Config.Tank 1 Fuel"=w381:string)
              n115 = Not Equal?(x=w381, y="Tank 1 Fuel Type") -> (x != y?=w379:bool)
              n116 = Bundle By Name(cluster=w384, "App Config.Tank 1 Fuel"="Tank 1 Fuel Type") -> (w383:T17)
            }
            frame 29 {
              w392 = T14[] [enum."Save Status"] items=["Main", "Init Files", "Init", "Save As", "Start Profile", "Check Step Time", "Alarm", "Run Step", "Stop Profile", "Cycle Reset", "Time Reset", "Time Reset All", "Time Set", "Tare CTs", "Save Profile", "Open Profile", "Get Profiles", "Update Screen", "Save Status", "Set Manual CMD", "Reset Restarts", "Reset Total Restarts", "Reset Cogs", "Disable Background", "Enable Background", "Get/Release Control", "Init AKLH", "Save AKLH", "Log Fuel Change", "Update Data Stream", "Init TenHz", "Read TenHz", "Remote Timer Reset", "Record Frequency Change", "Controller Change", "Get Alarms", "Init Alarms", "Save Alarms", "Init SubRoutine", "Next SubRoutine"]
              n117 = Unbundle By Name(w389) -> ("App Config.Tank 2 Fuel"=w387:string)
              n118 = Not Equal?(x=w387, y="Tank 2 Fuel Type") -> (x != y?=w388:bool)
              n119 = Bundle By Name(cluster=w391, "App Config.Tank 2 Fuel"="Tank 2 Fuel Type") -> (w390:T17)
            }
            frame 30 {
              w399 = T14[] [enum."Save Status"] items=["Main", "Init Files", "Init", "Save As", "Start Profile", "Check Step Time", "Alarm", "Run Step", "Stop Profile", "Cycle Reset", "Time Reset", "Time Reset All", "Time Set", "Tare CTs", "Save Profile", "Open Profile", "Get Profiles", "Update Screen", "Save Status", "Set Manual CMD", "Reset Restarts", "Reset Total Restarts", "Reset Cogs", "Disable Background", "Enable Background", "Get/Release Control", "Init AKLH", "Save AKLH", "Log Fuel Change", "Update Data Stream", "Init TenHz", "Read TenHz", "Remote Timer Reset", "Record Frequency Change", "Controller Change", "Get Alarms", "Init Alarms", "Save Alarms", "Init SubRoutine", "Next SubRoutine"]
              n120 = Unbundle By Name(w396) -> ("App Config.Serial Numbers"=w395:T31)
              n121 = Not Equal?(x=w395, y="Serial Numbers") -> (x != y?=w393:bool)
              n122 = Bundle By Name(cluster=w398, "App Config.Serial Numbers"="Serial Numbers") -> (w397:T17)
            }
            frame 31 {
              w400 = T14[] [enum."Save Status"] items=["Main", "Init Files", "Init", "Save As", "Start Profile", "Check Step Time", "Alarm", "Run Step", "Stop Profile", "Cycle Reset", "Time Reset", "Time Reset All", "Time Set", "Tare CTs", "Save Profile", "Open Profile", "Get Profiles", "Update Screen", "Save Status", "Set Manual CMD", "Reset Restarts", "Reset Total Restarts", "Reset Cogs", "Disable Background", "Enable Background", "Get/Release Control", "Init AKLH", "Save AKLH", "Log Fuel Change", "Update Data Stream", "Init TenHz", "Read TenHz", "Remote Timer Reset", "Record Frequency Change", "Controller Change", "Get Alarms", "Init Alarms", "Save Alarms", "Init SubRoutine", "Next SubRoutine"]
              n123 = Unbundle By Name(w407) -> ("Cog Limits:"=w402:i32[])
              n124 = Not Equal?(x="Cog Limits:", y=w402) -> (x != y?=w404:bool[])
              n125 = Or Array Elements(Boolean array=w404) -> (logical OR=w403:bool)
              n126 = Bundle By Name(cluster=w406, "Cog Limits:"="Cog Limits:") -> (w405:T17)
            }
            frame 32 {
              w408 = T14[] [enum."Save Status"] items=["Main", "Init Files", "Init", "Save As", "Start Profile", "Check Step Time", "Alarm", "Run Step", "Stop Profile", "Cycle Reset", "Time Reset", "Time Reset All", "Time Set", "Tare CTs", "Save Profile", "Open Profile", "Get Profiles", "Update Screen", "Save Status", "Set Manual CMD", "Reset Restarts", "Reset Total Restarts", "Reset Cogs", "Disable Background", "Enable Background", "Get/Release Control", "Init AKLH", "Save AKLH", "Log Fuel Change", "Update Data Stream", "Init TenHz", "Read TenHz", "Remote Timer Reset", "Record Frequency Change", "Controller Change", "Get Alarms", "Init Alarms", "Save Alarms", "Init SubRoutine", "Next SubRoutine"]
              n127 = local read "Cog Events:"() -> (w411:i32[])
              n128 = Unbundle By Name(w415) -> ("Cog Events"=w412:i32[])
              n129 = Not Equal?(x=w411, y=w412) -> (x != y?=w410:bool[])
              n130 = Bundle By Name(cluster=w414, "Cog Events"=w411) -> (w413:T17)
              n131 = Or Array Elements(Boolean array=w410) -> (logical OR=w409:bool)
            }
            frame 33 {
              w418 = T14[] [enum."Disable Background", enum."Reset Cogs"] items=["Main", "Init Files", "Init", "Save As", "Start Profile", "Check Step Time", "Alarm", "Run Step", "Stop Profile", "Cycle Reset", "Time Reset", "Time Reset All", "Time Set", "Tare CTs", "Save Profile", "Open Profile", "Get Profiles", "Update Screen", "Save Status", "Set Manual CMD", "Reset Restarts", "Reset Total Restarts", "Reset Cogs", "Disable Background", "Enable Background", "Get/Release Control", "Init AKLH", "Save AKLH", "Log Fuel Change", "Update Data Stream", "Init TenHz", "Read TenHz", "Remote Timer Reset", "Record Frequency Change", "Controller Change", "Get Alarms", "Init Alarms", "Save Alarms", "Init SubRoutine", "Next SubRoutine"]
            }
            frame 34 {
              n132 = call "Test Action Global.vi"() -> ("Data OUT"=w422:dbl, "Test Action OUT"=w424:T32)  [unwired: 10 in]
              n133 = case shown="\"Pump Cmd\"" w424 {
                selector: w424 -> [_ _ _ _ w451 w481]
                tunnel: [w426 w431 w433 w437 w444 w484] -> w425
                tunnel: w423 -> [_ _ _ _ w456 w483]
                tunnel: w422 -> [_ _ _ w442 w452 w482]
                tunnel: [w427 w432 w434 w440 w454 w480] -> w421
                tunnel: w420 -> [w427 w432 w434 w441 w455 w479]
                tunnel: [FALSE TRUE TRUE TRUE TRUE w476] -> w419
                frame "Idle", Default {
                  w426 = T14[] [] items=["Main", "Init Files", "Init", "Save As", "Start Profile", "Check Step Time", "Alarm", "Run Step", "Stop Profile", "Cycle Reset", "Time Reset", "Time Reset All", "Time Set", "Tare CTs", "Save Profile", "Open Profile", "Get Profiles", "Update Screen", "Save Status", "Set Manual CMD", "Reset Restarts", "Reset Total Restarts", "Reset Cogs", "Disable Background", "Enable Background", "Get/Release Control", "Init AKLH", "Save AKLH", "Log Fuel Change", "Update Data Stream", "Init TenHz", "Read TenHz", "Remote Timer Reset", "Record Frequency Change", "Controller Change", "Get Alarms", "Init Alarms", "Save Alarms", "Init SubRoutine", "Next SubRoutine"]
                }
                frame "Start" {
                  w431 = T14[] [enum."Start Profile"] items=["Main", "Init Files", "Init", "Save As", "Start Profile", "Check Step Time", "Alarm", "Run Step", "Stop Profile", "Cycle Reset", "Time Reset", "Time Reset All", "Time Set", "Tare CTs", "Save Profile", "Open Profile", "Get Profiles", "Update Screen", "Save Status", "Set Manual CMD", "Reset Restarts", "Reset Total Restarts", "Reset Cogs", "Disable Background", "Enable Background", "Get/Release Control", "Init AKLH", "Save AKLH", "Log Fuel Change", "Update Data Stream", "Init TenHz", "Read TenHz", "Remote Timer Reset", "Record Frequency Change", "Controller Change", "Get Alarms", "Init Alarms", "Save Alarms", "Init SubRoutine", "Next SubRoutine"]
                  n134 = local write "pb.Run Profile"(TRUE ("pb.Run Profile")) -> ()
                }
                frame "Stop" {
                  w433 = T14[] [enum."Stop Profile"] items=["Main", "Init Files", "Init", "Save As", "Start Profile", "Check Step Time", "Alarm", "Run Step", "Stop Profile", "Cycle Reset", "Time Reset", "Time Reset All", "Time Set", "Tare CTs", "Save Profile", "Open Profile", "Get Profiles", "Update Screen", "Save Status", "Set Manual CMD", "Reset Restarts", "Reset Total Restarts", "Reset Cogs", "Disable Background", "Enable Background", "Get/Release Control", "Init AKLH", "Save AKLH", "Log Fuel Change", "Update Data Stream", "Init TenHz", "Read TenHz", "Remote Timer Reset", "Record Frequency Change", "Controller Change", "Get Alarms", "Init Alarms", "Save Alarms", "Init SubRoutine", "Next SubRoutine"]
                }
                frame "Pump Cmd" {
                  w437 = T14[] [enum."Set Manual CMD"] items=["Main", "Init Files", "Init", "Save As", "Start Profile", "Check Step Time", "Alarm", "Run Step", "Stop Profile", "Cycle Reset", "Time Reset", "Time Reset All", "Time Set", "Tare CTs", "Save Profile", "Open Profile", "Get Profiles", "Update Screen", "Save Status", "Set Manual CMD", "Reset Restarts", "Reset Total Restarts", "Reset Cogs", "Disable Background", "Enable Background", "Get/Release Control", "Init AKLH", "Save AKLH", "Log Fuel Change", "Update Data Stream", "Init TenHz", "Read TenHz", "Remote Timer Reset", "Record Frequency Change", "Controller Change", "Get Alarms", "Init Alarms", "Save Alarms", "Init SubRoutine", "Next SubRoutine"]
                  n135 = Initialize Array(w442, 6 ("dimension size")) -> (w436:dbl[])
                  n136 = Bundle By Name(cluster=w441, "Manual CMDs"=w436) -> (w440:T17)
                  n137 = local write "Manual\nCMD"(w436) -> ()
                }
                frame "Pump 1 Enable".."Pump 6 Enable" {
                  w444 = T14[] [enum."Update Screen", enum."Save Status"] items=["Main", "Init Files", "Init", "Save As", "Start Profile", "Check Step Time", "Alarm", "Run Step", "Stop Profile", "Cycle Reset", "Time Reset", "Time Reset All", "Time Set", "Tare CTs", "Save Profile", "Open Profile", "Get Profiles", "Update Screen", "Save Status", "Set Manual CMD", "Reset Restarts", "Reset Total Restarts", "Reset Cogs", "Disable Background", "Enable Background", "Get/Release Control", "Init AKLH", "Save AKLH", "Log Fuel Change", "Update Data Stream", "Init TenHz", "Read TenHz", "Remote Timer Reset", "Record Frequency Change", "Controller Change", "Get Alarms", "Init Alarms", "Save Alarms", "Init SubRoutine", "Next SubRoutine"]
                  n138 = Unbundle By Name(w456) -> ("App Config.Pumps Present"=w453:u32)
                  n139 = case shown="\"Pump 1 Enable\", Default" w451 {
                    tunnel: w452 -> [w459 w462 w465 w468 w471 w474]
                    tunnel: [w458 w461 w464 w467 w470 w473] -> w450
                    tunnel: [0 ("index") 1 ("index") 2 ("index") 3 ("index") 4 ("index") 5 ("index")] -> w449
                    frame "Pump 1 Enable", Default {
                      n140 = Greater Than 0?(x=w459) -> (x > 0?=w458:bool)
                    }
                    frame "Pump 2 Enable" {
                      n141 = Greater Than 0?(x=w462) -> (x > 0?=w461:bool)
                    }
                    frame "Pump 3 Enable" {
                      n142 = Greater Than 0?(x=w465) -> (x > 0?=w464:bool)
                    }
                    frame "Pump 4 Enable" {
                      n143 = Greater Than 0?(x=w468) -> (x > 0?=w467:bool)
                    }
                    frame "Pump 5 Enable" {
                      n144 = Greater Than 0?(x=w471) -> (x > 0?=w470:bool)
                    }
                    frame "Pump 6 Enable" {
                      n145 = Greater Than 0?(x=w474) -> (x > 0?=w473:bool)
                    }
                  }
                  n146 = Number To Boolean Array(number=w453) -> (Boolean array=w448:bool[])
                  n147 = Replace Array Subset(array=w448, new element=w450, index=w449) -> (w447:bool[])
                  n148 = Array To Cluster(array=w447) -> (cluster=w446:T33)
                  n149 = local write "Pumps Present"(w446) -> ()
                  n150 = Boolean Array To Number(Boolean array=w447) -> (number=w445:u32)
                  n151 = Bundle By Name(cluster=w455, "App Config.Pumps Present"=w445) -> (w454:T17)
                }
                frame "Timer 1 Reset".."Timer 6 Reset" {
                  w484 = T14[] [enum."Remote Timer Reset"] items=["Main", "Init Files", "Init", "Save As", "Start Profile", "Check Step Time", "Alarm", "Run Step", "Stop Profile", "Cycle Reset", "Time Reset", "Time Reset All", "Time Set", "Tare CTs", "Save Profile", "Open Profile", "Get Profiles", "Update Screen", "Save Status", "Set Manual CMD", "Reset Restarts", "Reset Total Restarts", "Reset Cogs", "Disable Background", "Enable Background", "Get/Release Control", "Init AKLH", "Save AKLH", "Log Fuel Change", "Update Data Stream", "Init TenHz", "Read TenHz", "Remote Timer Reset", "Record Frequency Change", "Controller Change", "Get Alarms", "Init Alarms", "Save Alarms", "Init SubRoutine", "Next SubRoutine"]
                  n152 = Unbundle By Name(w483) -> ("pb.Resets"=w478:bool[])
                  n153 = case shown="\"Timer 1 Reset\", Default" w481 {
                    tunnel: w482 -> [w487 w490 w493 w496 w499 w502]
                    tunnel: [w486 w489 w492 w495 w498 w501] -> w476
                    tunnel: [0 ("index") 1 ("index") 2 ("index") 3 ("index") 4 ("index") 5 ("index")] -> w475
                    frame "Timer 1 Reset", Default {
                      n154 = Greater Than 0?(x=w487) -> (x > 0?=w486:bool)
                    }
                    frame "Timer 2 Reset" {
                      n155 = Greater Than 0?(x=w490) -> (x > 0?=w489:bool)
                    }
                    frame "Timer 3 Reset" {
                      n156 = Greater Than 0?(x=w493) -> (x > 0?=w492:bool)
                    }
                    frame "Timer 4 Reset" {
                      n157 = Greater Than 0?(x=w496) -> (x > 0?=w495:bool)
                    }
                    frame "Timer 5 Reset" {
                      n158 = Greater Than 0?(x=w499) -> (x > 0?=w498:bool)
                    }
                    frame "Timer 6 Reset" {
                      n159 = Greater Than 0?(x=w502) -> (x > 0?=w501:bool)
                    }
                  }
                  n160 = Replace Array Subset(array=w478, new element=w476, index=w475) -> (w477:bool[])
                  n161 = Bundle By Name(cluster=w479, "pb.Resets"=w477) -> (w480:T17)
                }
              }
            }
            frame 35 {
              w504 = T14[] [enum."Save Status", enum."Init TenHz"] items=["Main", "Init Files", "Init", "Save As", "Start Profile", "Check Step Time", "Alarm", "Run Step", "Stop Profile", "Cycle Reset", "Time Reset", "Time Reset All", "Time Set", "Tare CTs", "Save Profile", "Open Profile", "Get Profiles", "Update Screen", "Save Status", "Set Manual CMD", "Reset Restarts", "Reset Total Restarts", "Reset Cogs", "Disable Background", "Enable Background", "Get/Release Control", "Init AKLH", "Save AKLH", "Log Fuel Change", "Update Data Stream", "Init TenHz", "Read TenHz", "Remote Timer Reset", "Record Frequency Change", "Controller Change", "Get Alarms", "Init Alarms", "Save Alarms", "Init SubRoutine", "Next SubRoutine"]
              w505 = T14[] [enum."Save Status"] items=["Main", "Init Files", "Init", "Save As", "Start Profile", "Check Step Time", "Alarm", "Run Step", "Stop Profile", "Cycle Reset", "Time Reset", "Time Reset All", "Time Set", "Tare CTs", "Save Profile", "Open Profile", "Get Profiles", "Update Screen", "Save Status", "Set Manual CMD", "Reset Restarts", "Reset Total Restarts", "Reset Cogs", "Disable Background", "Enable Background", "Get/Release Control", "Init AKLH", "Save AKLH", "Log Fuel Change", "Update Data Stream", "Init TenHz", "Read TenHz", "Remote Timer Reset", "Record Frequency Change", "Controller Change", "Get Alarms", "Init Alarms", "Save Alarms", "Init SubRoutine", "Next SubRoutine"]
              n162 = Unbundle By Name(w510) -> ("TenHz Active?"=w508:bool)
              n163 = Not Equal?(x=w508, y="pb.TenHzSave") -> (x != y?=w509:bool)
              n164 = Greater?(x="pb.TenHzSave", y=w508) -> (0:w507:bool)
              n165 = Bundle By Name(cluster=w512, "TenHz Active?"="pb.TenHzSave") -> (w511:T17)
              n166 = Select(t=w504, s=w507, f=w505) -> (s? t:f=w506:T14[])
            }
            frame 36 {
              w513 = T14[] [enum."Record Frequency Change", enum."Save Status"] items=["Main", "Init Files", "Init", "Save As", "Start Profile", "Check Step Time", "Alarm", "Run Step", "Stop Profile", "Cycle Reset", "Time Reset", "Time Reset All", "Time Set", "Tare CTs", "Save Profile", "Open Profile", "Get Profiles", "Update Screen", "Save Status", "Set Manual CMD", "Reset Restarts", "Reset Total Restarts", "Reset Cogs", "Disable Background", "Enable Background", "Get/Release Control", "Init AKLH", "Save AKLH", "Log Fuel Change", "Update Data Stream", "Init TenHz", "Read TenHz", "Remote Timer Reset", "Record Frequency Change", "Controller Change", "Get Alarms", "Init Alarms", "Save Alarms", "Init SubRoutine", "Next SubRoutine"]
              n167 = Unbundle By Name(w519) -> ("App Config.TenHzFrequency"=w516:u32)
              n168 = Not Equal?(x="Record Frequency:", y=w516) -> (x != y?=w514:bool)
              n169 = Bundle By Name(cluster=w518, "App Config.TenHzFrequency"="Record Frequency:") -> (w517:T17)
            }
            frame 37 {
              w523 = T14[] [enum."Set Manual CMD", enum."Save Status"] items=["Main", "Init Files", "Init", "Save As", "Start Profile", "Check Step Time", "Alarm", "Run Step", "Stop Profile", "Cycle Reset", "Time Reset", "Time Reset All", "Time Set", "Tare CTs", "Save Profile", "Open Profile", "Get Profiles", "Update Screen", "Save Status", "Set Manual CMD", "Reset Restarts", "Reset Total Restarts", "Reset Cogs", "Disable Background", "Enable Background", "Get/Release Control", "Init AKLH", "Save AKLH", "Log Fuel Change", "Update Data Stream", "Init TenHz", "Read TenHz", "Remote Timer Reset", "Record Frequency Change", "Controller Change", "Get Alarms", "Init Alarms", "Save Alarms", "Init SubRoutine", "Next SubRoutine"]
              n170 = Unbundle By Name(w524) -> ("Power Relay"=w521:T2)
              n171 = Not Equal?(x="Power Relay", y=w521) -> (x != y?=w522:bool)
              n172 = Bundle By Name(cluster=w526, "Power Relay"="Power Relay") -> (w525:T17)
            }
            frame 38 {
              w533 = T14[] [enum."Set Manual CMD", enum."Save Status"] items=["Main", "Init Files", "Init", "Save As", "Start Profile", "Check Step Time", "Alarm", "Run Step", "Stop Profile", "Cycle Reset", "Time Reset", "Time Reset All", "Time Set", "Tare CTs", "Save Profile", "Open Profile", "Get Profiles", "Update Screen", "Save Status", "Set Manual CMD", "Reset Restarts", "Reset Total Restarts", "Reset Cogs", "Disable Background", "Enable Background", "Get/Release Control", "Init AKLH", "Save AKLH", "Log Fuel Change", "Update Data Stream", "Init TenHz", "Read TenHz", "Remote Timer Reset", "Record Frequency Change", "Controller Change", "Get Alarms", "Init Alarms", "Save Alarms", "Init SubRoutine", "Next SubRoutine"]
              n173 = Unbundle By Name(w531) -> ("Ignition Relay"=w528:T2)
              n174 = Not Equal?(x="Ignition Relay", y=w528) -> (x != y?=w532:bool)
              n175 = Bundle By Name(cluster=w530, "Ignition Relay"="Ignition Relay") -> (w529:T17)
            }
            frame 39 {
              n176 = local read "HMI Mom Buttons"() -> (w534:T1)
              n177 = flat-sequence {
                tunnel: w534 -> [_]
                frame #0 {
                  n178 = local write "HMI Mom Buttons"(T1 {"Stop"=FALSE, "Reset Timers"=FALSE, "Log Fuel Change"=FALSE} ("HMI Mom Buttons")) -> ()
                }
              }
              n179 = Cluster To Array(cluster=w534) -> (array=w538:bool[])
              n180 = Search 1D Array(1D array=w538, element=TRUE) -> (index of element=w536:i32)  [unwired: 1 in]
              n181 = case shown="0" w536 {
                tunnel: [w542 w543 w544 w545] -> w540
                frame -1, Default {
                  w542 = T14[] [] items=["Main", "Init Files", "Init", "Save As", "Start Profile", "Check Step Time", "Alarm", "Run Step", "Stop Profile", "Cycle Reset", "Time Reset", "Time Reset All", "Time Set", "Tare CTs", "Save Profile", "Open Profile", "Get Profiles", "Update Screen", "Save Status", "Set Manual CMD", "Reset Restarts", "Reset Total Restarts", "Reset Cogs", "Disable Background", "Enable Background", "Get/Release Control", "Init AKLH", "Save AKLH", "Log Fuel Change", "Update Data Stream", "Init TenHz", "Read TenHz", "Remote Timer Reset", "Record Frequency Change", "Controller Change", "Get Alarms", "Init Alarms", "Save Alarms", "Init SubRoutine", "Next SubRoutine"]
                }
                frame 0 {
                  w543 = T14[] [enum."Stop Profile"] items=["Main", "Init Files", "Init", "Save As", "Start Profile", "Check Step Time", "Alarm", "Run Step", "Stop Profile", "Cycle Reset", "Time Reset", "Time Reset All", "Time Set", "Tare CTs", "Save Profile", "Open Profile", "Get Profiles", "Update Screen", "Save Status", "Set Manual CMD", "Reset Restarts", "Reset Total Restarts", "Reset Cogs", "Disable Background", "Enable Background", "Get/Release Control", "Init AKLH", "Save AKLH", "Log Fuel Change", "Update Data Stream", "Init TenHz", "Read TenHz", "Remote Timer Reset", "Record Frequency Change", "Controller Change", "Get Alarms", "Init Alarms", "Save Alarms", "Init SubRoutine", "Next SubRoutine"]
                }
                frame 1 {
                  w544 = T14[] [enum."Remote Timer Reset"] items=["Main", "Init Files", "Init", "Save As", "Start Profile", "Check Step Time", "Alarm", "Run Step", "Stop Profile", "Cycle Reset", "Time Reset", "Time Reset All", "Time Set", "Tare CTs", "Save Profile", "Open Profile", "Get Profiles", "Update Screen", "Save Status", "Set Manual CMD", "Reset Restarts", "Reset Total Restarts", "Reset Cogs", "Disable Background", "Enable Background", "Get/Release Control", "Init AKLH", "Save AKLH", "Log Fuel Change", "Update Data Stream", "Init TenHz", "Read TenHz", "Remote Timer Reset", "Record Frequency Change", "Controller Change", "Get Alarms", "Init Alarms", "Save Alarms", "Init SubRoutine", "Next SubRoutine"]
                }
                frame 2 {
                  w545 = T14[] [enum."Log Fuel Change"] items=["Main", "Init Files", "Init", "Save As", "Start Profile", "Check Step Time", "Alarm", "Run Step", "Stop Profile", "Cycle Reset", "Time Reset", "Time Reset All", "Time Set", "Tare CTs", "Save Profile", "Open Profile", "Get Profiles", "Update Screen", "Save Status", "Set Manual CMD", "Reset Restarts", "Reset Total Restarts", "Reset Cogs", "Disable Background", "Enable Background", "Get/Release Control", "Init AKLH", "Save AKLH", "Log Fuel Change", "Update Data Stream", "Init TenHz", "Read TenHz", "Remote Timer Reset", "Record Frequency Change", "Controller Change", "Get Alarms", "Init Alarms", "Save Alarms", "Init SubRoutine", "Next SubRoutine"]
                }
              }
              n182 = Greater Or Equal To 0?(x=w536) -> (x >= 0?=w535:bool)
            }
            frame 40 {
              w552 = T14[] [enum."Save Alarms"] items=["Main", "Init Files", "Init", "Save As", "Start Profile", "Check Step Time", "Alarm", "Run Step", "Stop Profile", "Cycle Reset", "Time Reset", "Time Reset All", "Time Set", "Tare CTs", "Save Profile", "Open Profile", "Get Profiles", "Update Screen", "Save Status", "Set Manual CMD", "Reset Restarts", "Reset Total Restarts", "Reset Cogs", "Disable Background", "Enable Background", "Get/Release Control", "Init AKLH", "Save AKLH", "Log Fuel Change", "Update Data Stream", "Init TenHz", "Read TenHz", "Remote Timer Reset", "Record Frequency Change", "Controller Change", "Get Alarms", "Init Alarms", "Save Alarms", "Init SubRoutine", "Next SubRoutine"]
              n183 = Unbundle By Name(w550) -> ("Alarm Config"=w547:T7)
              n184 = Not Equal?(x="Alarm Config", y=w547) -> (x != y?=w551:bool)
              n185 = Bundle By Name(cluster=w549, "Alarm Config"="Alarm Config") -> (w548:T17)
            }
            frame 41 {
              w553 = T14[] [enum."Set Manual CMD"] items=["Main", "Init Files", "Init", "Save As", "Start Profile", "Check Step Time", "Alarm", "Run Step", "Stop Profile", "Cycle Reset", "Time Reset", "Time Reset All", "Time Set", "Tare CTs", "Save Profile", "Open Profile", "Get Profiles", "Update Screen", "Save Status", "Set Manual CMD", "Reset Restarts", "Reset Total Restarts", "Reset Cogs", "Disable Background", "Enable Background", "Get/Release Control", "Init AKLH", "Save AKLH", "Log Fuel Change", "Update Data Stream", "Init TenHz", "Read TenHz", "Remote Timer Reset", "Record Frequency Change", "Controller Change", "Get Alarms", "Init Alarms", "Save Alarms", "Init SubRoutine", "Next SubRoutine"]
              n186 = Unbundle By Name(w559) -> ("Pulse Frequency"=w555:dbl)
              n187 = local read "Pulse Frequency"() -> (w554:dbl)
              n188 = Not Equal?(x=w554, y=w555) -> (x != y?=w556:bool)
              n189 = Bundle By Name(cluster=w558, "Pulse Frequency"=w554) -> (w557:T17)
            }
            frame 42 {
              w561 = T14[] [enum."Set Manual CMD"] items=["Main", "Init Files", "Init", "Save As", "Start Profile", "Check Step Time", "Alarm", "Run Step", "Stop Profile", "Cycle Reset", "Time Reset", "Time Reset All", "Time Set", "Tare CTs", "Save Profile", "Open Profile", "Get Profiles", "Update Screen", "Save Status", "Set Manual CMD", "Reset Restarts", "Reset Total Restarts", "Reset Cogs", "Disable Background", "Enable Background", "Get/Release Control", "Init AKLH", "Save AKLH", "Log Fuel Change", "Update Data Stream", "Init TenHz", "Read TenHz", "Remote Timer Reset", "Record Frequency Change", "Controller Change", "Get Alarms", "Init Alarms", "Save Alarms", "Init SubRoutine", "Next SubRoutine"]
              n190 = Unbundle By Name(w566) -> ("1 Pulse Duty%"=w562:dbl)
              n191 = local read "1 Pulse Duty%"() -> (w560:dbl)
              n192 = Not Equal?(x=w560, y=w562) -> (x != y?=w563:bool)
              n193 = Bundle By Name(cluster=w565, "1 Pulse Duty%"=w560) -> (w564:T17)
            }
            frame 43 {
              w568 = T14[] [enum."Set Manual CMD"] items=["Main", "Init Files", "Init", "Save As", "Start Profile", "Check Step Time", "Alarm", "Run Step", "Stop Profile", "Cycle Reset", "Time Reset", "Time Reset All", "Time Set", "Tare CTs", "Save Profile", "Open Profile", "Get Profiles", "Update Screen", "Save Status", "Set Manual CMD", "Reset Restarts", "Reset Total Restarts", "Reset Cogs", "Disable Background", "Enable Background", "Get/Release Control", "Init AKLH", "Save AKLH", "Log Fuel Change", "Update Data Stream", "Init TenHz", "Read TenHz", "Remote Timer Reset", "Record Frequency Change", "Controller Change", "Get Alarms", "Init Alarms", "Save Alarms", "Init SubRoutine", "Next SubRoutine"]
              n194 = Unbundle By Name(w573) -> ("2 Pulse Duty%"=w569:dbl)
              n195 = local read "2 Pulse Duty%"() -> (w567:dbl)
              n196 = Not Equal?(x=w567, y=w569) -> (x != y?=w570:bool)
              n197 = Bundle By Name(cluster=w572, "2 Pulse Duty%"=w567) -> (w571:T17)
            }
            frame 44 {
              w575 = T14[] [enum."Set Manual CMD"] items=["Main", "Init Files", "Init", "Save As", "Start Profile", "Check Step Time", "Alarm", "Run Step", "Stop Profile", "Cycle Reset", "Time Reset", "Time Reset All", "Time Set", "Tare CTs", "Save Profile", "Open Profile", "Get Profiles", "Update Screen", "Save Status", "Set Manual CMD", "Reset Restarts", "Reset Total Restarts", "Reset Cogs", "Disable Background", "Enable Background", "Get/Release Control", "Init AKLH", "Save AKLH", "Log Fuel Change", "Update Data Stream", "Init TenHz", "Read TenHz", "Remote Timer Reset", "Record Frequency Change", "Controller Change", "Get Alarms", "Init Alarms", "Save Alarms", "Init SubRoutine", "Next SubRoutine"]
              n198 = Unbundle By Name(w580) -> ("3 Pulse Duty%"=w576:dbl)
              n199 = local read "3 Pulse Duty%"() -> (w574:dbl)
              n200 = Not Equal?(x=w574, y=w576) -> (x != y?=w577:bool)
              n201 = Bundle By Name(cluster=w579, "3 Pulse Duty%"=w574) -> (w578:T17)
            }
            frame 45 {
              w582 = T14[] [enum."Set Manual CMD"] items=["Main", "Init Files", "Init", "Save As", "Start Profile", "Check Step Time", "Alarm", "Run Step", "Stop Profile", "Cycle Reset", "Time Reset", "Time Reset All", "Time Set", "Tare CTs", "Save Profile", "Open Profile", "Get Profiles", "Update Screen", "Save Status", "Set Manual CMD", "Reset Restarts", "Reset Total Restarts", "Reset Cogs", "Disable Background", "Enable Background", "Get/Release Control", "Init AKLH", "Save AKLH", "Log Fuel Change", "Update Data Stream", "Init TenHz", "Read TenHz", "Remote Timer Reset", "Record Frequency Change", "Controller Change", "Get Alarms", "Init Alarms", "Save Alarms", "Init SubRoutine", "Next SubRoutine"]
              n202 = Unbundle By Name(w587) -> ("1 Pulsing"=w583:bool)
              n203 = local read "1 Pulsing"() -> (w581:bool)
              n204 = Not Equal?(x=w581, y=w583) -> (x != y?=w584:bool)
              n205 = Bundle By Name(cluster=w586, "1 Pulsing"=w581) -> (w585:T17)
            }
            frame 46 {
              w589 = T14[] [enum."Set Manual CMD"] items=["Main", "Init Files", "Init", "Save As", "Start Profile", "Check Step Time", "Alarm", "Run Step", "Stop Profile", "Cycle Reset", "Time Reset", "Time Reset All", "Time Set", "Tare CTs", "Save Profile", "Open Profile", "Get Profiles", "Update Screen", "Save Status", "Set Manual CMD", "Reset Restarts", "Reset Total Restarts", "Reset Cogs", "Disable Background", "Enable Background", "Get/Release Control", "Init AKLH", "Save AKLH", "Log Fuel Change", "Update Data Stream", "Init TenHz", "Read TenHz", "Remote Timer Reset", "Record Frequency Change", "Controller Change", "Get Alarms", "Init Alarms", "Save Alarms", "Init SubRoutine", "Next SubRoutine"]
              n206 = Unbundle By Name(w594) -> ("Solenoid 1"=w590:bool)
              n207 = local read "Solenoid 1"() -> (w588:bool)
              n208 = Not Equal?(x=w588, y=w590) -> (x != y?=w591:bool)
              n209 = Bundle By Name(cluster=w593, "Solenoid 1"=w588) -> (w592:T17)
            }
            frame 47 {
              w596 = T14[] [enum."Set Manual CMD"] items=["Main", "Init Files", "Init", "Save As", "Start Profile", "Check Step Time", "Alarm", "Run Step", "Stop Profile", "Cycle Reset", "Time Reset", "Time Reset All", "Time Set", "Tare CTs", "Save Profile", "Open Profile", "Get Profiles", "Update Screen", "Save Status", "Set Manual CMD", "Reset Restarts", "Reset Total Restarts", "Reset Cogs", "Disable Background", "Enable Background", "Get/Release Control", "Init AKLH", "Save AKLH", "Log Fuel Change", "Update Data Stream", "Init TenHz", "Read TenHz", "Remote Timer Reset", "Record Frequency Change", "Controller Change", "Get Alarms", "Init Alarms", "Save Alarms", "Init SubRoutine", "Next SubRoutine"]
              n210 = Unbundle By Name(w601) -> ("2 Pulsing"=w597:bool)
              n211 = local read "2 Pulsing"() -> (w595:bool)
              n212 = Not Equal?(x=w595, y=w597) -> (x != y?=w598:bool)
              n213 = Bundle By Name(cluster=w600, "2 Pulsing"=w595) -> (w599:T17)
            }
            frame 48 {
              w603 = T14[] [enum."Set Manual CMD"] items=["Main", "Init Files", "Init", "Save As", "Start Profile", "Check Step Time", "Alarm", "Run Step", "Stop Profile", "Cycle Reset", "Time Reset", "Time Reset All", "Time Set", "Tare CTs", "Save Profile", "Open Profile", "Get Profiles", "Update Screen", "Save Status", "Set Manual CMD", "Reset Restarts", "Reset Total Restarts", "Reset Cogs", "Disable Background", "Enable Background", "Get/Release Control", "Init AKLH", "Save AKLH", "Log Fuel Change", "Update Data Stream", "Init TenHz", "Read TenHz", "Remote Timer Reset", "Record Frequency Change", "Controller Change", "Get Alarms", "Init Alarms", "Save Alarms", "Init SubRoutine", "Next SubRoutine"]
              n214 = Unbundle By Name(w608) -> ("Solenoid 2"=w604:bool)
              n215 = local read "Solenoid 2"() -> (w602:bool)
              n216 = Not Equal?(x=w602, y=w604) -> (x != y?=w605:bool)
              n217 = Bundle By Name(cluster=w607, "Solenoid 2"=w602) -> (w606:T17)
            }
            frame 49 {
              w610 = T14[] [enum."Set Manual CMD"] items=["Main", "Init Files", "Init", "Save As", "Start Profile", "Check Step Time", "Alarm", "Run Step", "Stop Profile", "Cycle Reset", "Time Reset", "Time Reset All", "Time Set", "Tare CTs", "Save Profile", "Open Profile", "Get Profiles", "Update Screen", "Save Status", "Set Manual CMD", "Reset Restarts", "Reset Total Restarts", "Reset Cogs", "Disable Background", "Enable Background", "Get/Release Control", "Init AKLH", "Save AKLH", "Log Fuel Change", "Update Data Stream", "Init TenHz", "Read TenHz", "Remote Timer Reset", "Record Frequency Change", "Controller Change", "Get Alarms", "Init Alarms", "Save Alarms", "Init SubRoutine", "Next SubRoutine"]
              n218 = Unbundle By Name(w615) -> ("3 Pulsing"=w611:bool)
              n219 = local read "3 Pulsing"() -> (w609:bool)
              n220 = Not Equal?(x=w609, y=w611) -> (x != y?=w612:bool)
              n221 = Bundle By Name(cluster=w614, "3 Pulsing"=w609) -> (w613:T17)
            }
            frame 50 {
              w617 = T14[] [enum."Set Manual CMD"] items=["Main", "Init Files", "Init", "Save As", "Start Profile", "Check Step Time", "Alarm", "Run Step", "Stop Profile", "Cycle Reset", "Time Reset", "Time Reset All", "Time Set", "Tare CTs", "Save Profile", "Open Profile", "Get Profiles", "Update Screen", "Save Status", "Set Manual CMD", "Reset Restarts", "Reset Total Restarts", "Reset Cogs", "Disable Background", "Enable Background", "Get/Release Control", "Init AKLH", "Save AKLH", "Log Fuel Change", "Update Data Stream", "Init TenHz", "Read TenHz", "Remote Timer Reset", "Record Frequency Change", "Controller Change", "Get Alarms", "Init Alarms", "Save Alarms", "Init SubRoutine", "Next SubRoutine"]
              n222 = Unbundle By Name(w622) -> ("Solenoid 3"=w618:bool)
              n223 = local read "Solenoid 3"() -> (w616:bool)
              n224 = Not Equal?(x=w616, y=w618) -> (x != y?=w619:bool)
              n225 = Bundle By Name(cluster=w621, "Solenoid 3"=w616) -> (w620:T17)
            }
            frame 51 {
              w628 = T14[] [enum."Init SubRoutine", enum."Save Status"] items=["Main", "Init Files", "Init", "Save As", "Start Profile", "Check Step Time", "Alarm", "Run Step", "Stop Profile", "Cycle Reset", "Time Reset", "Time Reset All", "Time Set", "Tare CTs", "Save Profile", "Open Profile", "Get Profiles", "Update Screen", "Save Status", "Set Manual CMD", "Reset Restarts", "Reset Total Restarts", "Reset Cogs", "Disable Background", "Enable Background", "Get/Release Control", "Init AKLH", "Save AKLH", "Log Fuel Change", "Update Data Stream", "Init TenHz", "Read TenHz", "Remote Timer Reset", "Record Frequency Change", "Controller Change", "Get Alarms", "Init Alarms", "Save Alarms", "Init SubRoutine", "Next SubRoutine"]
              w629 = T14[] [enum."Save Status"] items=["Main", "Init Files", "Init", "Save As", "Start Profile", "Check Step Time", "Alarm", "Run Step", "Stop Profile", "Cycle Reset", "Time Reset", "Time Reset All", "Time Set", "Tare CTs", "Save Profile", "Open Profile", "Get Profiles", "Update Screen", "Save Status", "Set Manual CMD", "Reset Restarts", "Reset Total Restarts", "Reset Cogs", "Disable Background", "Enable Background", "Get/Release Control", "Init AKLH", "Save AKLH", "Log Fuel Change", "Update Data Stream", "Init TenHz", "Read TenHz", "Remote Timer Reset", "Record Frequency Change", "Controller Change", "Get Alarms", "Init Alarms", "Save Alarms", "Init SubRoutine", "Next SubRoutine"]
              w633 = 0 ("index (row)")
              n226 = Unbundle By Name(w627) -> ("SubRoutine Profile"=w624:i32[][])
              n227 = Index Array(array=w624, index (row)=w633, index (col)=w633) -> (element=w635:i32)
              n228 = Index Array(array="SubRoutine Profile", index (row)=w633, index (col)=w633) -> (element=w634:i32)
              n229 = Not Equal?(x=w624, y="SubRoutine Profile") -> (x != y?=w632:bool[][])
              n230 = Bundle By Name(cluster=w626, "SubRoutine Profile"="SubRoutine Profile") -> (w625:T17)
              n231 = Not Equal?(x=w635, y=w634) -> (x != y?=w636:bool)
              n232 = Or Array Elements(Boolean array=w632) -> (logical OR=w631:bool)
              n233 = Select(t=w628, s=w636, f=w629) -> (s? t:f=w630:T14[])
            }
            frame 52 {
              w637 = T14[] [enum."Init SubRoutine"] items=["Main", "Init Files", "Init", "Save As", "Start Profile", "Check Step Time", "Alarm", "Run Step", "Stop Profile", "Cycle Reset", "Time Reset", "Time Reset All", "Time Set", "Tare CTs", "Save Profile", "Open Profile", "Get Profiles", "Update Screen", "Save Status", "Set Manual CMD", "Reset Restarts", "Reset Total Restarts", "Reset Cogs", "Disable Background", "Enable Background", "Get/Release Control", "Init AKLH", "Save AKLH", "Log Fuel Change", "Update Data Stream", "Init TenHz", "Read TenHz", "Remote Timer Reset", "Record Frequency Change", "Controller Change", "Get Alarms", "Init Alarms", "Save Alarms", "Init SubRoutine", "Next SubRoutine"]
              n234 = Unbundle By Name(w640) -> ("Run Subs"=w641:bool)
              n235 = Greater?(x="pb.Run SubRoutines", y=w641) -> (0:w643:bool)
              n236 = Bundle By Name(cluster=w639, "Run Subs"="pb.Run SubRoutines") -> (w638:T17)
            }
          }
        }
        n237 = Get Date/Time In Seconds() -> (seconds since 1Jan1904=w179:timestamp)
        n238 = To Double Precision Float(number=w179) -> (double precision float=w189:dbl)
        n239 = Subtract(x=w189, y=w203) -> (x-y=w193:dbl)
        n240 = Subtract(x=w189, y=w187) -> (x-y=w194:dbl)
        n241 = Subtract(x=w189, y=w186) -> (x-y=w195:dbl)
        n242 = case shown="True" w178 {
          selector: w178 -> [w205 _]
          tunnel: w179 -> [_ w209]
          tunnel: w177 -> [_ w207]
          tunnel: [w205 w206] -> w173
          frame False {
          }
          frame True {
            n243 = Seconds To Date/Time(time stamp (now)=w209) -> (date time rec=w210:T34)  [unwired: 1 in]
            n244 = Unbundle By Name(w210) -> ("day of month"=w208:i32)
            n245 = Not Equal?(x=w208, y=w207) -> (x != y?=w206:bool)
          }
        }
        n246 = Greater?(x=w193, y=0.5) -> (0:w197:bool)
        n247 = Greater?(x=w194, y=0.1) -> (0:w182:bool)
        n248 = Greater?(x=w195, y=600.0) -> (0:w181:bool)
        n249 = case shown="False" w200 {
          tunnel: w199 -> [w651 _]
          tunnel: [w645 w652] -> w191
          tunnel: w198 -> [_ w652]
          tunnel: w197 -> [w644 _]
          frame False {
            w648 = T14[] [enum."Check Step Time"] items=["Main", "Init Files", "Init", "Save As", "Start Profile", "Check Step Time", "Alarm", "Run Step", "Stop Profile", "Cycle Reset", "Time Reset", "Time Reset All", "Time Set", "Tare CTs", "Save Profile", "Open Profile", "Get Profiles", "Update Screen", "Save Status", "Set Manual CMD", "Reset Restarts", "Reset Total Restarts", "Reset Cogs", "Disable Background", "Enable Background", "Get/Release Control", "Init AKLH", "Save AKLH", "Log Fuel Change", "Update Data Stream", "Init TenHz", "Read TenHz", "Remote Timer Reset", "Record Frequency Change", "Controller Change", "Get Alarms", "Init Alarms", "Save Alarms", "Init SubRoutine", "Next SubRoutine"]
            n250 = Select(t=Sequence_States."Update Screen", s=w644, f=Sequence_States."Main") -> (s? t:f=w647:T14)
            n251 = Build Array(w647) -> (w646:T14[])
            n252 = Select(t=w648, s=w651, f=w646) -> (s? t:f=w645:T14[])
          }
          frame True {
          }
        }
        n253 = Select(t=Sequence_States."Init TenHz", s=w173, f=Sequence_States."Save AKLH") -> (s? t:f=w175:T14)
        n254 = Compound Arithmetic op=OR(w182, w181, w173) -> (w180:bool)
        n255 = Select(t=Sequence_States."Read TenHz", s=w182, f=w175) -> (s? t:f=w188:T14)
        n256 = Bundle By Name(cluster=w202, "Update Screen"=w197) -> (w204:T17)
        n257 = case shown="True" w180 {
          tunnel: w191 -> [w211 w215]
          tunnel: w188 -> [_ w214]
          tunnel: [w211 w212] -> w190
          frame False {
          }
          frame True {
            n258 = Insert Into Array(array=w215, index=0, new element=w214) -> (w212:T14[])
          }
        }
      }
      frame "Init Files" {
        # "changed tick divider to 1 as I was\nalready taking care of scaling\ntime when I do a data read that\nway data is only modified in one spot"
        n259 = Unbundle By Name(w662) -> ("App Config"=w680:T16, "AKLH Path"=w666:path, "TenHz Path"=w667:path)
        n260 = disable-structure shown="Enabled" {
          disable-tunnel: [w695 dbl[][] [[0.0, 1.0], [0.0, 1.0], [0.0, 1.0], [0.0, 1.0], [0.0, 1.0], [0.0, 1.0], [0.0, 1.0], [0.0, 1.0], [0.0, 1.0], [0.0, 1.0], [0.0, 1.0], [0.0, 1.0], [0.0, 1.0], [0.0, 1.0], [0.0, 1.0], [0.0, 1.0], [0.0, 1.0], [0.0, 1.0], [0.0, 1.0], [0.0, 1.0], [0.0, 1.0], [0.0, 1.0], [0.0, 1.0], [0.0, 1.0], [0.0, 1.0], [0.0, 1.0], [0.0, 1.0], [0.0, 1.0], [0.0, 1.0], [0.0, 1.0], [0.0, 1.0], [0.0, 1.0], [0.0, 1.0], [0.0, 1.0], [0.0, 1.0], [0.0, 1.0], [0.0, 1.0], [0.0, 1.0], [0.0, 1.0], [0.0, 1.0], [0.0, 1.0], [0.0, 1.0], [0.0, 1.0], [0.0, 1.0], [0.0, 1.0], [0.0, 1.0], [0.0, 1.0], [0.0, 1.0], [0.0, 1.0], [0.0, 1.0], [0.0, 1.0], [0.0, 1.0], [0.0, 1.0], [0.0, 1.0]]] -> w659
          frame Disabled {
            w686 = dbl[][] [[0.0, 11.0, 0.0, 0.0, 0.0], [0.0, 11.0, 0.0, 0.0, 0.0], [0.0, 11.0, 0.0, 0.0, 0.0], [0.0, 11.0, 0.0, 0.0, 0.0], [0.0, 11.0, 0.0, 0.0, 0.0], [0.0, 11.0, 0.0, 0.0, 0.0], [0.0, 1.0, 0.0, 0.0, 0.0], [0.0, 1.0, 0.0, 0.0, 0.0], [0.0, 1.0, 0.0, 0.0, 0.0], [0.0, 2.0, 0.0, 0.0, 0.0], [0.0, 1.0, 0.0, 0.0, 0.0], [0.0, 1.0, 0.0, 0.0, 0.0], [0.0, 1.0, 0.0, 0.0, 0.0], [0.0, 1.0, 0.0, 0.0, 0.0], [0.0, 1.0, 0.0, 0.0, 0.0], [0.0, 1.0, 0.0, 0.0, 0.0], [0.0, 1.0, 0.0, 0.0, 0.0], [0.0, 1.0, 0.0, 0.0, 0.0], [0.0, 1.0, 0.0, 0.0, 0.0], [0.0, 1.0, 0.0, 0.0, 0.0], [0.0, 1.0, 0.0, 0.0, 0.0], [0.0, 1.0, 0.0, 0.0, 0.0], [-60.0, 24.0, 0.0, 0.0, 0.0], [-60.0, 24.0, 0.0, 0.0, 0.0], [-60.0, 24.0, 0.0, 0.0, 0.0], [-60.0, 24.0, 0.0, 0.0, 0.0], [-60.0, 24.0, 0.0, 0.0, 0.0], [-60.0, 24.0, 0.0, 0.0, 0.0], [-660.0, 200.0, 0.0, 0.0, 0.0], [-660.0, 200.0, 0.0, 0.0, 0.0], [-258.5, 258.5, 0.0, 0.0, 0.0], [-258.5, 258.5, 0.0, 0.0, 0.0], [-258.5, 258.5, 0.0, 0.0, 0.0], [-258.5, 258.5, 0.0, 0.0, 0.0], [-258.5, 258.5, 0.0, 0.0, 0.0], [-258.5, 258.5, 0.0, 0.0, 0.0], [-150.0, 150.0, 0.0, 0.0, 0.0], [-150.0, 150.0, 0.0, 0.0, 0.0], [-150.0, 150.0, 0.0, 0.0, 0.0], [-150.0, 150.0, 0.0, 0.0, 0.0], [-150.0, 150.0, 0.0, 0.0, 0.0], [-150.0, 150.0, 0.0, 0.0, 0.0], [0.0, 1.0, 0.0, 0.0, 0.0], [0.0, 1.0, 0.0, 0.0, 0.0], [0.0, 1.0, 0.0, 0.0, 0.0], [0.0, 1.0, 0.0, 0.0, 0.0], [0.0, 1.0, 0.0, 0.0, 0.0], [0.0, 1.0, 0.0, 0.0, 0.0], [0.0, 0.0001, 0.0, 0.0, 0.0], [0.0, 0.0001, 0.0, 0.0, 0.0], [0.0, 0.0001, 0.0, 0.0, 0.0], [0.0, 0.0001, 0.0, 0.0, 0.0], [0.0, 0.0001, 0.0, 0.0, 0.0], [0.0, 0.0001, 0.0, 0.0, 0.0]]  # Cal Coefficients
            # "This is 10.30.189.0"
            n261 = String To IP() -> (0:w692:u32)  [unwired: 1 in]
            n262 = Subtract(x=w692, y=u32 169786624) -> (x-y=w691:u32)
            n263 = Number To Decimal String(number=w691) -> (decimal integer string=w690:string)  [unwired: 1 in]
            n264 = Concatenate Strings("c:\\" ("string"), w690, ".cal" ("string")) -> (w687:string)
            n265 = String To Path(string=w687) -> ()  [unwired: 1 out]
            n266 = call "Get Cal Coefficients.vi"("Path"=path "c:/160.cal") -> ("Error"=w694:bool, "Cal Coefficients"=w696:dbl[][])  [unwired: 9 in]
            n267 = case shown="False" w694 {
              tunnel: w696 -> [_ w700]
              tunnel: [w697 w699] -> w695
              tunnel: w686 -> [w697 w698]
              frame True {
              }
              frame False {
                n268 = for {
                  tunnel: w700 -> [w702] mode=indexing
                  shift-right: [w703] -> w699
                  shift-left: w698 -> [w704]
                  i -> [w701]
                  n269 = Index Array(array=w702) -> (element #1=w715:dbl, element #2=w714:dbl, element #3=w713:dbl, element #4=w709:dbl, element #5=w708:dbl)  [unwired: 5 in]
                  n270 = Equal To 0?(x=w715) -> (x = 0?=w712:bool)
                  n271 = Equal To 0?(x=w714) -> (x = 0?=w711:bool)
                  n272 = Equal To 0?(x=w713) -> (x = 0?=w710:bool)
                  n273 = Equal To 0?(x=w709) -> (x = 0?=w707:bool)
                  n274 = Equal To 0?(x=w708) -> (x = 0?=w706:bool)
                  n275 = Compound Arithmetic op=AND(w712, w711, w710, w707, w706) -> (w705:bool)
                  n276 = case shown="False" w705 {
                    tunnel: w704 -> [w719 w720]
                    tunnel: [w718 w720] -> w703
                    tunnel: w702 -> [w717 _]
                    tunnel: w701 -> [w716 _]
                    frame False {
                      n277 = Replace Array Subset(array=w719, new element=w717, index (row)=w716) -> (w718:dbl[][])  [unwired: 1 in]
                    }
                    frame True {
                    }
                  }
                }
              }
            }
          }
          frame Enabled {
          }
        }
        n278 = Build Array(w666, w667) -> (w665:path[])
        n279 = call <vilib>:"Open Config Data.vi"("configuration file path"=path "c:/App Config.ini") -> ("error out"=w682:errorcluster, "file created?"=w678:bool, "refnum"=w683:T35)  [unwired: 8 in]
        n280 = case shown="False" w678 {
          tunnel: w683 -> [w738 w742]
          tunnel: w682 -> [w736 _]
          tunnel: w680 -> [w733 w749]
          tunnel: [w734 w747] -> w679
          frame False {
            # "Read App Config.ini"
            n281 = call "Read Write App Config.vi"("Error IN"=w736, "App Config IN"=w733, "Refnum in"=w738) -> ("Error OUT"=w735:errorcluster, "App Config OUT"=w734:T16, "Refnum out"=w737:T35)  [unwired: 6 in]
            n282 = call <vilib>:"Close Config Data.vi"("error in (no error)"=w735, "refnum"=w737) -> ("error out"=w739:errorcluster)  [unwired: 8 in, 1 out]
            n283 = call <vilib>:"Clear Errors.vi"("error in (no error)"=w739) -> ()  [unwired: 6 in, 1 out]
          }
          frame True {
            # "Doesn't exists, so create."
            n284 = Bundle By Name(cluster=w749, "Profiles Path"=path "c:/Profiles", "PWM Freq (Hz)"=100.0, "Pumps Present"=u32 63, "TenHzFrequency"=u32 1) -> (w747:T16)
            n285 = call "Read Write App Config.vi"("Write (F)"=TRUE, "App Config IN"=w747, "Refnum in"=w742) -> ("Error OUT"=w745:errorcluster, "Refnum out"=w746:T35)  [unwired: 6 in, 1 out]
            n286 = call <vilib>:"Close Config Data.vi"("error in (no error)"=w745, "refnum"=w746) -> ()  [unwired: 8 in, 2 out]
          }
        }
        n287 = for {
          tunnel: w665 -> [w723] mode=indexing
          tunnel: [w722] -> w664 mode=indexing
          n288 = call <vilib>:"Check if File or Folder Exists.vi"("path"=w723) -> ("error out"=w727:errorcluster, "file or folder exists?"=w726:bool, "dup path"=w728:path)  [unwired: 8 in]
          n289 = case shown="False" w726 {
            tunnel: w728 -> [w731 w732]
            tunnel: w727 -> [w729 _]
            tunnel: [w730 w732] -> w724
            frame False {
              n290 = Create Folder(path (use dialog)=w731, error in=w729) -> (created path=w730:path)  [unwired: 1 in, 2 out]
            }
            frame True {
            }
          }
          n291 = Build Path(base path=w724, name or relative path="StartingPoint.csv") -> (appended path=w722:path)
        }
        n292 = Index Array(array=w664) -> (element #1=w663:path, element #2=w655:path)  [unwired: 2 in]
        n293 = call "Tank Data Global.vi"("Pump Data Mode"=Pump_Data_Mode."Write Cal", "Cal Coefficients"=w659) -> ()  [unwired: 9 in, 1 out]
        n294 = call "Get Restarts Data.vi"("Path"=path "c:/Restarts" ("file (use dialog)")) -> ("Cogging Data"=w658:cluster{"CogEvents":i32[], "CogLimits":i32[]}, "Restarts Limits"=w671:T3, "Actual Starts"=w672:T15, "Restarts Cluster"=w673:T4)  [unwired: 7 in]
        n295 = call "Get Elapsed Times.vi"("Path"=path "c:/ElapsedTimes" ("file (use dialog)")) -> ("Elapsed Times"=w669:dbl[])  [unwired: 9 in, 1 out]
        n296 = call "Get CT Offsets.vi"("Path"=path "c:/CT Offsets" ("file (use dialog)")) -> ("CT Offsets"=w674:fxp<+,24,6>[])  [unwired: 10 in]
        n297 = call "Get SubRoutines.vi"("Path"=path "c:/SubRoutine") -> ("SubRoutine Profile"=w653:i32[][])  [unwired: 10 in]
        n298 = call "Elapsed Time Global.vi"("Write (F)"=TRUE, "Tick Divider"=1.0, "Initial Times IN"=w669) -> ()  [unwired: 8 in, 1 out]
        n299 = Unbundle(w658) -> ("CogEvents"=w656:i32[], "CogLimits"=w657:i32[])
        n300 = Bundle By Name(cluster=w662, "SubRoutine Profile"=w653, "AKLH Path"=w663, "TenHz Path"=w655, "App Config"=w679, "Restarts Cluster"=w673, "Actual Starts"=w672, "Restarts Limits"=w671, "Intitial Times"=w669, "CT Offsets"=w674, "Cog Events"=w656, "Cog Limits:"=w657) -> (w661:T17)
        n301 = local write "Cog Events:"(w656) -> ()
        n302 = local write "Cog Limits:"(w657) -> ()
      }
      frame "Init" {
        (unwired) fxp<+/-,16,9> 74.5546875 ("PumpCurrentM")
        w772 = T10 [{"Controller Name"=enum."Kuhnke", "CommSeg"=2, "PWM?"=TRUE, "Frequency"=100, "Low Command"=10.0, "High Command"=100.0, "Stop Command"=10.0, "Command Step"=0.1, "Solenoid Stop?"=FALSE, "Controller?"=FALSE, "Invert PWM"=TRUE}, {"Controller Name"=enum."Conti", "CommSeg"=2, "PWM?"=FALSE, "Frequency"=100, "Low Command"=0.0, "High Command"=800.0, "Stop Command"=0.0, "Command Step"=1.0, "Solenoid Stop?"=FALSE, "Controller?"=FALSE, "Invert PWM"=FALSE}, {"Controller Name"=enum."Helbako", "CommSeg"=2, "PWM?"=FALSE, "Frequency"=100, "Low Command"=0.0, "High Command"=100.0, "Stop Command"=0.0, "Command Step"=0.1, "Solenoid Stop?"=FALSE, "Controller?"=FALSE, "Invert PWM"=FALSE}, {"Controller Name"=enum."TI PWM", "CommSeg"=2, "PWM?"=TRUE, "Frequency"=100, "Low Command"=0.0, "High Command"=100.0, "Stop Command"=0.0, "Command Step"=0.1, "Solenoid Stop?"=FALSE, "Controller?"=FALSE, "Invert PWM"=FALSE}, {"Controller Name"=enum."PSA", "CommSeg"=2, "PWM?"=TRUE, "Frequency"=100, "Low Command"=5.0, "High Command"=95.0, "Stop Command"=5.0, "Command Step"=0.1, "Solenoid Stop?"=FALSE, "Controller?"=FALSE, "Invert PWM"=FALSE}, {"Controller Name"=enum."Hella Gas", "CommSeg"=2, "PWM?"=FALSE, "Frequency"=100, "Low Command"=0.0, "High Command"=800.0, "Stop Command"=0.0, "Command Step"=1.0, "Solenoid Stop?"=TRUE, "Controller?"=FALSE, "Invert PWM"=FALSE}, {"Controller Name"=enum."Hella Diesel", "CommSeg"=2, "PWM?"=FALSE, "Frequency"=100, "Low Command"=370.0, "High Command"=461.0, "Stop Command"=370.0, "Command Step"=1.0, "Solenoid Stop?"=TRUE, "Controller?"=FALSE, "Invert PWM"=FALSE}, {"Controller Name"=enum."8 Comm", "CommSeg"=8, "PWM?"=FALSE, "Frequency"=100, "Low Command"=0.0, "High Command"=1.0, "Stop Command"=0.0, "Command Step"=1.0, "Solenoid Stop?"=FALSE, "Controller?"=FALSE, "Invert PWM"=FALSE}, {"Controller Name"=enum."10 Comm", "CommSeg"=10, "PWM?"=FALSE, "Frequency"=100, "Low Command"=0.0, "High Command"=1.0, "Stop Command"=0.0, "Command Step"=1.0, "Solenoid Stop?"=FALSE, "Controller?"=FALSE, "Invert PWM"=FALSE}, {"Controller Name"=enum."8 Comm Hella", "CommSeg"=8, "PWM?"=TRUE, "Frequency"=150, "Low Command"=0.0, "High Command"=50.0, "Stop Command"=80.0, "Command Step"=0.1, "Solenoid Stop?"=FALSE, "Controller?"=FALSE, "Invert PWM"=FALSE}, {"Controller Name"=enum."10 Comm Hella", "CommSeg"=10, "PWM?"=TRUE, "Frequency"=150, "Low Command"=0.0, "High Command"=50.0, "Stop Command"=80.0, "Command Step"=0.1, "Solenoid Stop?"=FALSE, "Controller?"=FALSE, "Invert PWM"=FALSE}, {"Controller Name"=enum."8 Comm Omron", "CommSeg"=8, "PWM?"=TRUE, "Frequency"=150, "Low Command"=5.0, "High Command"=50.0, "Stop Command"=75.0, "Command Step"=0.1, "Solenoid Stop?"=FALSE, "Controller?"=FALSE, "Invert PWM"=FALSE}, {"Controller Name"=enum."10 Comm Omron", "CommSeg"=10, "PWM?"=TRUE, "Frequency"=150, "Low Command"=5.0, "High Command"=50.0, "Stop Command"=75.0, "Command Step"=0.1, "Solenoid Stop?"=FALSE, "Controller?"=FALSE, "Invert PWM"=FALSE}, {"Controller Name"=enum."8 Comm Nissan", "CommSeg"=8, "PWM?"=TRUE, "Frequency"=10, "Low Command"=50.0, "High Command"=90.0, "Stop Command"=50.0, "Command Step"=0.1, "Solenoid Stop?"=TRUE, "Controller?"=FALSE, "Invert PWM"=FALSE}, {"Controller Name"=enum."10 Comm Nissan", "CommSeg"=10, "PWM?"=TRUE, "Frequency"=10, "Low Command"=50.0, "High Command"=90.0, "Stop Command"=50.0, "Command Step"=0.1, "Solenoid Stop?"=TRUE, "Controller?"=FALSE, "Invert PWM"=FALSE}]  # Controller List
        w794 = T14[] [enum."Init AKLH", enum."Init TenHz", enum."Get Profiles", enum."Enable Background", enum."Get/Release Control", enum."Record Frequency Change", enum."Get Alarms"] items=["Main", "Init Files", "Init", "Save As", "Start Profile", "Check Step Time", "Alarm", "Run Step", "Stop Profile", "Cycle Reset", "Time Reset", "Time Reset All", "Time Set", "Tare CTs", "Save Profile", "Open Profile", "Get Profiles", "Update Screen", "Save Status", "Set Manual CMD", "Reset Restarts", "Reset Total Restarts", "Reset Cogs", "Disable Background", "Enable Background", "Get/Release Control", "Init AKLH", "Save AKLH", "Log Fuel Change", "Update Data Stream", "Init TenHz", "Read TenHz", "Remote Timer Reset", "Record Frequency Change", "Controller Change", "Get Alarms", "Init Alarms", "Save Alarms", "Init SubRoutine", "Next SubRoutine"]
        w796 = T14[] [enum."Init AKLH", enum."Get Profiles", enum."Enable Background", enum."Get/Release Control", enum."Record Frequency Change", enum."Get Alarms"] items=["Main", "Init Files", "Init", "Save As", "Start Profile", "Check Step Time", "Alarm", "Run Step", "Stop Profile", "Cycle Reset", "Time Reset", "Time Reset All", "Time Set", "Tare CTs", "Save Profile", "Open Profile", "Get Profiles", "Update Screen", "Save Status", "Set Manual CMD", "Reset Restarts", "Reset Total Restarts", "Reset Cogs", "Disable Background", "Enable Background", "Get/Release Control", "Init AKLH", "Save AKLH", "Log Fuel Change", "Update Data Stream", "Init TenHz", "Read TenHz", "Remote Timer Reset", "Record Frequency Change", "Controller Change", "Get Alarms", "Init Alarms", "Save Alarms", "Init SubRoutine", "Next SubRoutine"]
        w797 = 40000000.0  # 40 MHz
        n303 = Unbundle By Name(w789) -> ("App Config.TenHzFrequency"=w784:u32, "App Config.Profiles Path"=w788:path, "App Config.Record TenHz"=w781:bool, "App Config.Controller Type:"=w798:T5)
        n304 = local write "pb.Run Profile"(FALSE ("pb.Run Profile")) -> ()
        n305 = local write "Main Tab"(enum32{"Main", "Data Stream", "Alarms"}."Main" ("Main Tab")) -> ()
        n306 = Index Array(array=w772, index=w798) -> (element=w783:T11)
        n307 = local write "Record Frequency:"(w784) -> ()
        n308 = local write "pb.TenHzSave"(w781) -> ()
        n309 = Unbundle By Name(w783) -> ("High Command"=w787:dbl, "Low Command"=w786:dbl, "Command Step"=w785:dbl, "Stop Command"=w790:dbl, "Frequency"=w782:i32, "Controller Name"=w764:T5)
        n310 = xnode "Invoke Method"("FPGA VI Reference In"=w793) -> ("FPGA VI Reference Out"=w792:refnum<k20>)  [unwired: 1 in, 1 out]
        n311 = property on="Manual CMD" class="DigNum (strict)"("Maximum"=w787, "Minimum"=w786, "Increment"=w785) -> ()  [unwired: 2 in, 2 out]
        n312 = Divide(x=w797, y=w782) -> (x/y=w763:dbl)
        n313 = Divide(x=w763, y=100.0) -> (x/y=w761:dbl)
        n314 = case shown="\"Kuhnke\"" w764 {
          tunnel: w761 -> [_ w816 w825 w830 w835]
          tunnel: [0 w815 w824 w829 w834] -> w760
          tunnel: [9 w814 9 w828 w833] -> w758
          tunnel: [4 w814 4 w828 w833] -> w757
          tunnel: [0 w814 0 w828 w833] -> w756
          tunnel: [230 w814 230 w828 w833] -> w755
          tunnel: [2147483647 w814 2147483647 w828 w833] -> w754
          tunnel: [0.0 w812 w817 w827 w831] -> w752
          frame Default {
          }
          frame "Kuhnke" {
            w814 = 0
            w812 = 10.0 ("y")
            n315 = Multiply(x=w816, y=w812) -> (x*y=w813:dbl)
            n316 = To Long Integer(number=w813) -> (32bit integer=w815:i32)
          }
          frame "PSA" {
            w817 = 5.0 ("y")
            n317 = Multiply(x=w825, y=w817) -> (x*y=w818:dbl)
            n318 = To Long Integer(number=w818) -> (32bit integer=w824:i32)
          }
          frame "8 Comm Hella", "10 Comm Hella" {
            w828 = 0
            w827 = 80.0 ("y")
            n319 = Multiply(x=w830, y=w827) -> (x*y=w826:dbl)
            n320 = To Long Integer(number=w826) -> (32bit integer=w829:i32)
          }
          frame "8 Comm Omron", "10 Comm Omron" {
            w833 = 0
            w831 = 75.0 ("y")
            n321 = Multiply(x=w835, y=w831) -> (x*y=w832:dbl)
            n322 = To Long Integer(number=w832) -> (32bit integer=w834:i32)
          }
        }
        n323 = To Unsigned Long Integer(number=w763) -> (unsigned 32bit integer=w804:u32)
        n324 = xnode "Read/Write Control"("FPGA VI Reference In"=w792, "PWM Period (Ticks)"=w804, "Loop Timer (uSec)"=u32 100, "Threshold"=fxp<+/-,24,6> 1.5, "Kuhnke Window"=33 ("Period Delta"), "Consec Samples"=500, "Current Scale"=fxp<+,16,5> 24.0, "Current Offset"=fxp<+/-,18,7> -60.0, "Speed Hysteresis"=fxp<+,23,5> 1.0, "Arm Level"=w758, "Disarm Level"=w757, "Spike Window"=w756, "Min Window"=w755, "Max Window"=w754, "Duty (Ticks) 1"=w760, "Duty (Ticks) 2"=w760, "Duty (Ticks) 3"=w760, "Duty (Ticks) 4"=w760, "Duty (Ticks) 5"=w760, "Duty (Ticks) 6"=w760, "PS Control"=FALSE, "Current Offsets"=fxp<+/-,24,7>[] [0.0, 0.0, 0.0, 0.0, 0.0, 0.0]) -> ("FPGA VI Reference Out"=w776:refnum<k20>, "error out"=w775:errorcluster)  [unwired: 1 in]
        n325 = call <vilib>:"Check if File or Folder Exists.vi"("path"=w788) -> ("file or folder exists?"=w803:bool, "dup path"=w802:path)  [unwired: 8 in, 1 out]
        n326 = disable-structure shown="Enabled" {
          disable-tunnel: w776 -> [w839 w841]
          disable-tunnel: w775 -> [w838 w840]
          disable-tunnel: [w837 w841] -> w774
          disable-tunnel: [w836 w840] -> w773
          frame Disabled {
            n327 = call "Init FPGA.vi"("error in (no error)"=w838, "FPGA Ref"=w839) -> ("error out"=w836:errorcluster, "FPGA Ref OUT"=w837:T25)  [unwired: 8 in]
          }
          frame Enabled {
          }
        }
        n328 = Initialize Array(w752, 6 ("dimension size")) -> (w751:dbl[])
        n329 = case shown="False" w803 {
          tunnel: w802 -> [w847 _]
          frame False {
            n330 = Create Folder(path (use dialog)=w847) -> ()  [unwired: 2 in, 3 out]
          }
          frame True {
          }
        }
        n331 = xnode "Invoke Method"("FPGA VI Reference In"=w774, "error in"=w773, "Wait Until Done (F)"=FALSE) -> ("FPGA VI Reference Out"=w780:refnum<k20>, "error out"=w778:errorcluster)
        n332 = Bundle By Name(cluster=w789, "Controller List"=w772, "Stop Cmd"=w790, "Manual CMDs"=w751, "Last CMDs"=w751) -> (w791:T17)
        n333 = local write "Manual\nCMD"(w751) -> ()
        n334 = flat-sequence {
          tunnel: w780 -> [w842]
          tunnel: w779 -> [w843]
          tunnel: w778 -> [w844]
          tunnel: [w843] -> w777
          frame #0 {
            n335 = disable-structure shown="Disabled" {
              disable-tunnel: w844 -> [w846 _]
              disable-tunnel: w842 -> [w845 _]
              frame Disabled {
                n336 = call "Init ADCs.vi"("Error IN"=w846, "FPGA Ref"=w845) -> ()  [unwired: 7 in, 3 out]
              }
              frame Enabled {
              }
            }
          }
        }
        n337 = Set Occurrence(w777) -> ()
        n338 = Select(t=w794, s=w781, f=w796) -> (s? t:f=w795:T14[])
      }
      frame "Get Alarms" {
        n339 = Unbundle By Name(w855) -> ("Alarm Config"=w856:T7, "Alarm Config Path"=w853:path)
        n340 = call <vilib>:"Check if File or Folder Exists.vi"("path"=w853) -> ("file or folder exists?"=w858:bool, "dup path"=w857:path)  [unwired: 8 in, 1 out]
        n341 = case shown="False" w858 {
          tunnel: w857 -> [w863 w868]
          tunnel: w856 -> [_ w866]
          tunnel: [w860 w864] -> w848
          frame False {
            w860 = T7 {"Alarms:"=[{"Description:"="", "Enabled:"=FALSE, "Data Index:"=0, "Data Type:"="", "Low Limit:"=0.0, "High Limit:"=0.0, "Trip Time:"=0, "Profile Sync:"=FALSE}, {"Description:"="", "Enabled:"=FALSE, "Data Index:"=0, "Data Type:"="", "Low Limit:"=0.0, "High Limit:"=0.0, "Trip Time:"=0, "Profile Sync:"=FALSE}, {"Description:"="", "Enabled:"=FALSE, "Data Index:"=0, "Data Type:"="", "Low Limit:"=0.0, "High Limit:"=0.0, "Trip Time:"=0, "Profile Sync:"=FALSE}, {"Description:"="", "Enabled:"=FALSE, "Data Index:"=0, "Data Type:"="", "Low Limit:"=0.0, "High Limit:"=0.0, "Trip Time:"=0, "Profile Sync:"=FALSE}, {"Description:"="", "Enabled:"=FALSE, "Data Index:"=0, "Data Type:"="", "Low Limit:"=0.0, "High Limit:"=0.0, "Trip Time:"=0, "Profile Sync:"=FALSE}, {"Description:"="", "Enabled:"=FALSE, "Data Index:"=0, "Data Type:"="", "Low Limit:"=0.0, "High Limit:"=0.0, "Trip Time:"=0, "Profile Sync:"=FALSE}, {"Description:"="", "Enabled:"=FALSE, "Data Index:"=0, "Data Type:"="", "Low Limit:"=0.0, "High Limit:"=0.0, "Trip Time:"=0, "Profile Sync:"=FALSE}, {"Description:"="", "Enabled:"=FALSE, "Data Index:"=0, "Data Type:"="", "Low Limit:"=0.0, "High Limit:"=0.0, "Trip Time:"=0, "Profile Sync:"=FALSE}], "Profile Sync:"={"Trip Time:"=0, "Consecutive Trips:"=0}} ("Alarm Config")
            n342 = Flatten To JSON(anything=w860) -> (JSON string=w859:string)  [unwired: 2 in, 1 out]
            n343 = Write to Text File(file (use dialog)=w863, text=w859) -> (refnum out=w862:refnum<file>, error out=w861:errorcluster)  [unwired: 2 in, 1 out]
            n344 = Close File(refnum=w862, error in=w861) -> ()  [unwired: 2 out]
          }
          frame True {
            n345 = Read from Text File(file (use dialog)=w868) -> (refnum out=w865:refnum<file>, text=w867:string)  [unwired: 3 in, 2 out]
            n346 = Close File(refnum=w865) -> ()  [unwired: 1 in, 2 out]
            n347 = Unflatten From JSON(JSON string=w867, type and defaults=w866) -> (value=w864:T7)  [unwired: 5 in, 1 out]
          }
        }
        n348 = Bundle By Name(cluster=w855, "Alarm Config"=w848) -> (w854:T17)
        n349 = local write "Alarm Config"(w848) -> ()
        n350 = Insert Into Array(array=w849, index=0, new element=Sequence_States."Init Alarms") -> (w850:T14[])
      }
      frame "Init Alarms" {
        # "Initialize alarm arrays."
        n351 = Unbundle By Name(w875) -> ("Alarm Config.Alarms:"=w877:T8[])
        n352 = for {
          tunnel: w877 -> [w884] mode=indexing
          shift-right: [w880] -> w871
          shift-left: 0 -> [w879]
          n353 = Unbundle By Name(w884) -> ("Data Type:"=w883:string, "Enabled:"=w882:bool)
          n354 = case shown="\"Pump\", Default" w883 {
            tunnel: [6 1] -> w881
            frame "Pump", Default {
            }
            frame "Tank" {
            }
          }
          n355 = case shown="True" w882 {
            tunnel: w881 -> [_ w888]
            tunnel: [w885 w887] -> w880
            tunnel: w879 -> [w885 w886]
            frame False {
            }
            frame True {
              n356 = Add(x=w888, y=w886) -> (x+y=w887:i32)
            }
          }
        }
        n357 = Tick Count (ms)() -> (millisecond timer value=w872:u32)
        n358 = Initialize Array(0, w871) -> (w870:i32[])
        n359 = Initialize Array(w872, w871) -> (w869:u32[])
        n360 = Bundle By Name(cluster=w875, "Trip Counters"=w870, "Previous Times"=w869) -> (w874:T17)
      }
      frame "Save Alarms" {
        n361 = Unbundle By Name(w894) -> ("Alarm Config Path"=w892:path, "Alarm Config"=w893:T7)
        n362 = Flatten To JSON(anything=w893) -> (JSON string=w891:string)  [unwired: 2 in, 1 out]
        n363 = Write to Text File(file (use dialog)=w892, text=w891) -> ()  [unwired: 2 in, 3 out]
      }
      frame "Get Profiles" {
        n364 = Unbundle By Name(w903) -> ("App Config.Profiles Path"=w904:path)
        n365 = List Folder(path=w904) -> (filenames=w901:string[], error out=w900:errorcluster)  [unwired: 3 in, 2 out]
        n366 = call <vilib>:"Clear Errors.vi"("error in (no error)"=w900) -> ()  [unwired: 6 in, 1 out]
        n367 = property on="Profile Name:" class="CmbBox"("Strings[]"=w901) -> ()  [unwired: 2 in, 2 out]
        n368 = Bundle By Name(cluster=w903, "Profiles"=w901) -> (w902:T17)
        n369 = Insert Into Array(array=w897, index=0, new element=Sequence_States."Open Profile") -> (w896:T14[])
      }
      frame "Open Profile" {
        w906 = T14[] [enum."Update Screen", enum."Save Status"] items=["Main", "Init Files", "Init", "Save As", "Start Profile", "Check Step Time", "Alarm", "Run Step", "Stop Profile", "Cycle Reset", "Time Reset", "Time Reset All", "Time Set", "Tare CTs", "Save Profile", "Open Profile", "Get Profiles", "Update Screen", "Save Status", "Set Manual CMD", "Reset Restarts", "Reset Total Restarts", "Reset Cogs", "Disable Background", "Enable Background", "Get/Release Control", "Init AKLH", "Save AKLH", "Log Fuel Change", "Update Data Stream", "Init TenHz", "Read TenHz", "Remote Timer Reset", "Record Frequency Change", "Controller Change", "Get Alarms", "Init Alarms", "Save Alarms", "Init SubRoutine", "Next SubRoutine"]
        n370 = Unbundle By Name(w919) -> ("App Config.Profiles Path"=w921:path, "App Config.Current Profile"=w920:string)
        n371 = Build Path(base path=w921, name or relative path=w920) -> (appended path=w916:path)
        n372 = Read from Text File(file (use dialog)=w916) -> (refnum out=w914:refnum<file>, text=w915:string, error out=w913:errorcluster)  [unwired: 3 in, 1 out]
        n373 = Close File(refnum=w914, error in=w913) -> (error out=w912:errorcluster)  [unwired: 1 out]
        n374 = case shown="No Error" w912 {
          tunnel: w915 -> [w923 _]
          tunnel: [w924 string[][] []] -> w905
          frame No Error {
            n375 = Spreadsheet String To Array(delimiter (Tab)=",", format string="%s", spreadsheet string=w923, array type (2D Dbl)=string[][] []) -> (array=w924:string[][])
          }
          frame Error {
          }
        }
        n376 = Array Size(array=w905) -> (size(s)=w917:i32[])
        n377 = Index Array(array=w917) -> (element=w910:i32)  [unwired: 1 in]
        n378 = Bundle By Name(cluster=w919, "Profile"=w905, "# of Steps"=w910, "Update Profile"=TRUE) -> (w918:T17)
        n379 = Insert Into Array(array=w908, index=0, new element=w906) -> (w907:T14[])
      }
      frame "Save Profile" {
        n380 = Unbundle By Name(w934) -> ("App Config.Profiles Path"=w938:path, "App Config.Current Profile"=w936:string, "Profile"=w937:string[][])
        n381 = Empty String/Path?(string/path=w936) -> (empty?=w935:bool)
        n382 = case shown="False" w935 {
          tunnel: w938 -> [w943 _]
          tunnel: w936 -> [w942 _]
          tunnel: w937 -> [w941 _]
          tunnel: [w940 string[][] [] ("Profile OUT")] -> w930
          tunnel: [w939 w944] -> w932
          frame False {
            w939 = T14[] [enum."Update Screen"] items=["Main", "Init Files", "Init", "Save As", "Start Profile", "Check Step Time", "Alarm", "Run Step", "Stop Profile", "Cycle Reset", "Time Reset", "Time Reset All", "Time Set", "Tare CTs", "Save Profile", "Open Profile", "Get Profiles", "Update Screen", "Save Status", "Set Manual CMD", "Reset Restarts", "Reset Total Restarts", "Reset Cogs", "Disable Background", "Enable Background", "Get/Release Control", "Init AKLH", "Save AKLH", "Log Fuel Change", "Update Data Stream", "Init TenHz", "Read TenHz", "Remote Timer Reset", "Record Frequency Change", "Controller Change", "Get Alarms", "Init Alarms", "Save Alarms", "Init SubRoutine", "Next SubRoutine"]
            n383 = call "Save Profile.vi"("Profile"=w941, "Current Profile"=w942, "Profiles Path"=w943) -> ("Profile OUT"=w940:string[][])  [unwired: 8 in]
          }
          frame True {
            w944 = T14[] [enum."Main"] items=["Main", "Init Files", "Init", "Save As", "Start Profile", "Check Step Time", "Alarm", "Run Step", "Stop Profile", "Cycle Reset", "Time Reset", "Time Reset All", "Time Set", "Tare CTs", "Save Profile", "Open Profile", "Get Profiles", "Update Screen", "Save Status", "Set Manual CMD", "Reset Restarts", "Reset Total Restarts", "Reset Cogs", "Disable Background", "Enable Background", "Get/Release Control", "Init AKLH", "Save AKLH", "Log Fuel Change", "Update Data Stream", "Init TenHz", "Read TenHz", "Remote Timer Reset", "Record Frequency Change", "Controller Change", "Get Alarms", "Init Alarms", "Save Alarms", "Init SubRoutine", "Next SubRoutine"]
          }
        }
        n384 = Array Size(array=w930) -> (size(s)=w931:i32[])
        n385 = Index Array(array=w931) -> (element=w929:i32)  [unwired: 1 in]
        n386 = Bundle By Name(cluster=w934, "Profile"=w930, "# of Steps"=w929, "Update Profile"=TRUE) -> (w933:T17)
      }
      frame "Start Profile" {
        w947 = T14[] [enum."Init Alarms", enum."Check Step Time"] items=["Main", "Init Files", "Init", "Save As", "Start Profile", "Check Step Time", "Alarm", "Run Step", "Stop Profile", "Cycle Reset", "Time Reset", "Time Reset All", "Time Set", "Tare CTs", "Save Profile", "Open Profile", "Get Profiles", "Update Screen", "Save Status", "Set Manual CMD", "Reset Restarts", "Reset Total Restarts", "Reset Cogs", "Disable Background", "Enable Background", "Get/Release Control", "Init AKLH", "Save AKLH", "Log Fuel Change", "Update Data Stream", "Init TenHz", "Read TenHz", "Remote Timer Reset", "Record Frequency Change", "Controller Change", "Get Alarms", "Init Alarms", "Save Alarms", "Init SubRoutine", "Next SubRoutine"]
        w946 = 0 ("Current Step")
        n387 = property on="Main Tab" class="TabCtl (strict)"("DisabledEnum"=T27."Disabled" ("Disabled")) -> ()  [unwired: 2 in, 2 out]
        n388 = Get Date/Time In Seconds() -> (seconds since 1Jan1904=w951:timestamp)
        n389 = To Double Precision Float(number=w951) -> (double precision float=w950:dbl)
        n390 = Bundle By Name(cluster=w954, "Run Profile"=TRUE, "Step Start Time"=w950, "Last Profile Time"=w950, "Step Time"=0.0, "Current Step"=w946, "Stagger Counter"=w946) -> (w953:T17)
      }
      frame "Check Step Time" {
        # "Time elapsed since\nstart of step."
        n391 = Unbundle By Name(w977) -> ("Step Start Time"=w980:dbl, "Step Time"=w978:dbl, "Current Step"=w973:i32, "App Config.Stagger Time (ms)"=w956:i32, "Stagger Counter"=w962:i32, "Update Screen"=w971:bool)
        n392 = Get Date/Time In Seconds() -> (seconds since 1Jan1904=w979:timestamp)
        n393 = Increment(x=w962) -> (x+1=w957:i32)
        n394 = To Double Precision Float(number=w979) -> (double precision float=w970:dbl)
        n395 = Multiply(x=w956, y=w957) -> (x*y=w968:i32)
        n396 = Subtract(x=w970, y=w980) -> (x-y=w967:dbl)
        n397 = To Double Precision Float(number=w968) -> (double precision float=w961:dbl)
        n398 = Divide(x=w961, y=1000.0) -> (x/y=w959:dbl)
        n399 = Not Equal To 0?(x=w956) -> (x != 0?=w955:bool)
        n400 = Greater Or Equal?(x=w967, y=w959) -> (x >= y?=w966:bool)
        n401 = Less Or Equal?(x=w962, y=4) -> (x <= y?=w964:bool)
        n402 = Subtract(x=w978, y=w967) -> (x-y=w975:dbl)
        n403 = Compound Arithmetic op=AND(w966, w964, w955) -> (w963:bool)
        n404 = Less Or Equal To 0?(x=w975) -> (x <= 0?=w958:bool)
        n405 = case shown="True" w958 {
          tunnel: [w985 w996] -> w974
          tunnel: w973 -> [w986 w998]
          tunnel: [w986 w997] -> w972
          tunnel: w971 -> [w984 _]
          tunnel: [w981 0 ("Stagger Counter")] -> w969
          tunnel: w963 -> [w983 _]
          tunnel: w962 -> [w982 _]
          frame False {
            # "There's time left.  Update screen."
            n406 = case shown="True" w983 {
              tunnel: [w991 w994] -> w985
              tunnel: w984 -> [w990 _]
              tunnel: w982 -> [w987 w993]
              tunnel: [w987 w992] -> w981
              frame False {
                w988 = T14[] [enum."Main"] items=["Main", "Init Files", "Init", "Save As", "Start Profile", "Check Step Time", "Alarm", "Run Step", "Stop Profile", "Cycle Reset", "Time Reset", "Time Reset All", "Time Set", "Tare CTs", "Save Profile", "Open Profile", "Get Profiles", "Update Screen", "Save Status", "Set Manual CMD", "Reset Restarts", "Reset Total Restarts", "Reset Cogs", "Disable Background", "Enable Background", "Get/Release Control", "Init AKLH", "Save AKLH", "Log Fuel Change", "Update Data Stream", "Init TenHz", "Read TenHz", "Remote Timer Reset", "Record Frequency Change", "Controller Change", "Get Alarms", "Init Alarms", "Save Alarms", "Init SubRoutine", "Next SubRoutine"]
                w989 = T14[] [enum."Update Screen"] items=["Main", "Init Files", "Init", "Save As", "Start Profile", "Check Step Time", "Alarm", "Run Step", "Stop Profile", "Cycle Reset", "Time Reset", "Time Reset All", "Time Set", "Tare CTs", "Save Profile", "Open Profile", "Get Profiles", "Update Screen", "Save Status", "Set Manual CMD", "Reset Restarts", "Reset Total Restarts", "Reset Cogs", "Disable Background", "Enable Background", "Get/Release Control", "Init AKLH", "Save AKLH", "Log Fuel Change", "Update Data Stream", "Init TenHz", "Read TenHz", "Remote Timer Reset", "Record Frequency Change", "Controller Change", "Get Alarms", "Init Alarms", "Save Alarms", "Init SubRoutine", "Next SubRoutine"]
                n407 = Select(t=w989, s=w990, f=w988) -> (s? t:f=w991:T14[])
              }
              frame True {
                w994 = T14[] [enum."Run Step"] items=["Main", "Init Files", "Init", "Save As", "Start Profile", "Check Step Time", "Alarm", "Run Step", "Stop Profile", "Cycle Reset", "Time Reset", "Time Reset All", "Time Set", "Tare CTs", "Save Profile", "Open Profile", "Get Profiles", "Update Screen", "Save Status", "Set Manual CMD", "Reset Restarts", "Reset Total Restarts", "Reset Cogs", "Disable Background", "Enable Background", "Get/Release Control", "Init AKLH", "Save AKLH", "Log Fuel Change", "Update Data Stream", "Init TenHz", "Read TenHz", "Remote Timer Reset", "Record Frequency Change", "Controller Change", "Get Alarms", "Init Alarms", "Save Alarms", "Init SubRoutine", "Next SubRoutine"]
                n408 = Increment(x=w993) -> (x+1=w992:i32)
              }
            }
          }
          frame True {
            w996 = T14[] [enum."Run Step"] items=["Main", "Init Files", "Init", "Save As", "Start Profile", "Check Step Time", "Alarm", "Run Step", "Stop Profile", "Cycle Reset", "Time Reset", "Time Reset All", "Time Set", "Tare CTs", "Save Profile", "Open Profile", "Get Profiles", "Update Screen", "Save Status", "Set Manual CMD", "Reset Restarts", "Reset Total Restarts", "Reset Cogs", "Disable Background", "Enable Background", "Get/Release Control", "Init AKLH", "Save AKLH", "Log Fuel Change", "Update Data Stream", "Init TenHz", "Read TenHz", "Remote Timer Reset", "Record Frequency Change", "Controller Change", "Get Alarms", "Init Alarms", "Save Alarms", "Init SubRoutine", "Next SubRoutine"]
            # "No time left.  Go to next step."
            n409 = Increment(x=w998) -> (x+1=w997:i32)
          }
        }
        n410 = Bundle By Name(cluster=w977, "Last Profile Time"=w970, "Step Time Left"=w975, "New Step"=w958, "Current Step"=w972, "Stagger Counter"=w969) -> (w976:T17)
      }
      frame "Run Step" {
        n411 = Unbundle By Name(w1021) -> ("App Config.VoltCtrlRef"=w1012:string, "Profile"=w1023:string[][], "Current Step"=w1002:i32, "# of Steps"=w1008:i32, "App Config.Stagger Time (ms)"=w1013:i32, "App Config.Cycles Completed"=w1000:u32, "App Config.PWM Freq (Hz)"=w1022:dbl, "App Config.Controller Type:"=w1016:T5, "Restarts Cluster"=w1019:T4, "Stagger Counter"=w1014:i32, "Last CMDs"=w1018:dbl[], "App Config.Pumps Present"=w1017:u32, "Step Start Time"=w1009:dbl, "New Step"=w1010:bool, "ReqCycles"=w1006:u32, "Run Subs"=w1007:bool)
        n412 = case shown="True" w1007 {
          tunnel: w1002 -> [w1085 w1093]
          tunnel: w1008 -> [_ w1092]
          tunnel: w1000 -> [w1084 w1091]
          tunnel: w1006 -> [_ w1090]
          tunnel: [TRUE ("Run Run Step") w1089] -> w1005
          tunnel: [w1085 w1088] -> w1001
          tunnel: [w1084 w1087] -> w999
          frame False {
          }
          frame True {
            n413 = call "SubRoutine Stepper.vi"("Current Step in"=w1093, "# of Steps"=w1092, "Cycles Completed in"=w1091, "Cycles Required"=w1090) -> ("Current Step out"=w1088:i32, "Cycles Completed out"=w1087:u32, "Run Run Step"=w1089:bool)  [unwired: 9 in]
          }
        }
        n414 = control-ref of="CAN CMD"() -> (w1015:refnum<vi>)
        n415 = case shown="True" w1005 {
          tunnel: w1023 -> [_ w1080]
          tunnel: w1022 -> [_ w1079]
          tunnel: w1021 -> [w1031 w1078]
          tunnel: [w1030 w1077] -> w1020
          tunnel: w1019 -> [_ w1073]
          tunnel: w1018 -> [_ w1072]
          tunnel: w1017 -> [_ w1070]
          tunnel: w1016 -> [_ w1069]
          tunnel: w1015 -> [_ w1068]
          tunnel: w1014 -> [_ w1066]
          tunnel: w1013 -> [_ w1065]
          tunnel: w1012 -> [_ w1062]
          tunnel: w1011 -> [_ w1050]
          tunnel: w1010 -> [_ w1047]
          tunnel: w1009 -> [_ w1046]
          tunnel: w1001 -> [w1025 w1039]
          tunnel: w1008 -> [_ w1038]
          tunnel: w999 -> [w1024 w1037]
          tunnel: w1004 -> [w1029 w1036]
          tunnel: [w1028 w1036] -> w1003
          frame False {
            w1026 = T14[] [enum."Next SubRoutine", enum."Run Step"] items=["Main", "Init Files", "Init", "Save As", "Start Profile", "Check Step Time", "Alarm", "Run Step", "Stop Profile", "Cycle Reset", "Time Reset", "Time Reset All", "Time Set", "Tare CTs", "Save Profile", "Open Profile", "Get Profiles", "Update Screen", "Save Status", "Set Manual CMD", "Reset Restarts", "Reset Total Restarts", "Reset Cogs", "Disable Background", "Enable Background", "Get/Release Control", "Init AKLH", "Save AKLH", "Log Fuel Change", "Update Data Stream", "Init TenHz", "Read TenHz", "Remote Timer Reset", "Record Frequency Change", "Controller Change", "Get Alarms", "Init Alarms", "Save Alarms", "Init SubRoutine", "Next SubRoutine"]
            n416 = Insert Into Array(array=w1029, index=0, new element=w1026) -> (w1028:T14[])
            n417 = Bundle By Name(cluster=w1031, "Current Step"=w1025, "App Config.Cycles Completed"=w1024) -> (w1030:T17)
          }
          frame True {
            n418 = call "Run Step.vi"("CAN Cmd Ref"=w1068, "FPGA Ref"=w1050, "Stagger Time (ms)"=w1065, "Cycles Completed in"=w1037, "PWM Freq (Hz)"=w1079, "Controller Type:"=w1069, "# of Steps"=w1038, "Restarts Cluster"=w1073, "VoltCtrlRef"=w1062, "Stagger Counter"=w1066, "Current Step in"=w1039, "Last CMDs"=w1072, "Profile"=w1080, "Pumps Present"=w1070) -> ("PS Cmd"=w1063:dbl, "Controls"=w1058:T36, "Ignition Relays"=w1059:T2, "Manual CMDs"=w1061:dbl[], "Current Step out"=w1075:i32, "Press Cmd"=w1064:dbl, "Cycles Completed out"=w1074:u32, "Step Time"=w1076:dbl, "Power Relays"=w1060:T2, "Restarts Cluster OUT"=w1071:T4)  [unwired: 4 in]
            n419 = Unbundle(w1058) -> (w1040:dbl, w1048:dbl, w1049:dbl, w1051:dbl, w1057:dbl, w1056:dbl, w1055:dbl, w1054:dbl, w1053:dbl, w1052:dbl)  [unwired: 2 out]
            n420 = local write "Power Supply Cmd (V):"(w1063) -> ()
            n421 = local write "PressureCMD"(w1064) -> ()
            n422 = local write "Manual\nCMD"(w1061) -> ()
            n423 = Not Equal To 0?(x=w1057) -> (x != 0?=w1044:bool)
            n424 = Not Equal To 0?(x=w1056) -> (x != 0?=w1035:bool)
            n425 = Not Equal To 0?(x=w1055) -> (x != 0?=w1034:bool)
            n426 = Not Equal To 0?(x=w1054) -> (x != 0?=w1033:bool)
            n427 = Not Equal To 0?(x=w1053) -> (x != 0?=w1032:bool)
            n428 = Not Equal To 0?(x=w1052) -> (x != 0?=w1045:bool)
            n429 = local write "Pulse Frequency"(w1040) -> ()
            n430 = local write "1 Pulse Duty%"(w1048) -> ()
            n431 = local write "2 Pulse Duty%"(w1049) -> ()
            n432 = local write "3 Pulse Duty%"(w1051) -> ()
            n433 = local write "1 Pulsing"(w1044) -> ()
            n434 = local write "2 Pulsing"(w1035) -> ()
            n435 = local write "3 Pulsing"(w1034) -> ()
            n436 = local write "Solenoid 1"(w1033) -> ()
            n437 = local write "Solenoid 2"(w1032) -> ()
            n438 = local write "Solenoid 3"(w1045) -> ()
            n439 = case shown="False" w1047 {
              tunnel: [w1081 w1082] -> w1067
              tunnel: w1046 -> [w1081 _]
              tunnel: w1061 -> [_ _]
              frame False {
              }
              frame True {
                n440 = Get Date/Time In Seconds() -> (seconds since 1Jan1904=w1083:timestamp)
                n441 = To Double Precision Float(number=w1083) -> (double precision float=w1082:dbl)
              }
            }
            n442 = To Word Integer(number=w1048) -> (16bit integer=w1041:i16)
            n443 = To Word Integer(number=w1049) -> (16bit integer=w1042:i16)
            n444 = To Word Integer(number=w1051) -> (16bit integer=w1043:i16)
            n445 = xnode "Read/Write Control"("FPGA VI Reference In"=w1050, "Pulse Frequency"=w1040, "Module 1 Pulse Duty"=w1041, "Module 2 Pulse Duty"=w1042, "Module 3 Pulse Duty"=w1043, "Mod1 Pulsing?"=w1044, "Mod1 On?"=w1035, "Mod2 Pulsing?"=w1034, "Mod2 On?"=w1033, "Mod3 Pulsing?"=w1032, "Mod3 On?"=w1045) -> ()  [unwired: 1 in, 2 out]
            n446 = local write "Power Relay"(w1060) -> ()
            n447 = local write "Ignition Relay"(w1059) -> ()
            n448 = Bundle By Name(cluster=w1078, "PS CMD"=w1063, "Press CMD"=w1064, "Current Step"=w1075, "App Config.Cycles Completed"=w1074, "Step Time"=w1076, "Restarts Cluster"=w1071, "Last CMDs"=w1061, "Step Start Time"=w1067, "Power Relay"=w1060, "Ignition Relay"=w1059, "Pulse Frequency"=w1040, "1 Pulse Duty%"=w1048, "2 Pulse Duty%"=w1049, "3 Pulse Duty%"=w1051, "1 Pulsing"=w1044, "Solenoid 1"=w1035, "2 Pulsing"=w1034, "Solenoid 2"=w1033, "3 Pulsing"=w1032, "Solenoid 3"=w1045) -> (w1077:T17)
          }
        }
      }
      frame "Update Screen" {
        w1125 = FALSE ("Update Screen")
        w1166 = bool[] [FALSE, FALSE, FALSE, FALSE, FALSE, FALSE] ("pb.Resets")
        # "there used to be a case structure\nover updating the main bundle it was off\nmaking sure that all elapsed times were\ngreater than or equal to the initial times\nthis should mean that it was just watching\nfor a rollover case but I feel that is probably\nunnecessary with a double"
        n449 = Unbundle By Name(w1167) -> ("SubRoutine Profile"=w1094:i32[][], "App Config.Stagger Time (ms)"=w1137:i32, "Update Profile"=w1138:bool, "Profile"=w1139:string[][], "App Config.Current Profile"=w1105:string, "App Config.Location"=→"Location:":string, "App Config.CA Number"=w1104:string, "App Config.Cycles Completed"=→"Cycles Completed:":u32, "Current Step"=→"Current Step:":i32, "Step Time Left"=→"Step Time Left:":dbl, "App Config.Controller Type:"=w1140:T5, "Restarts Cluster"=w1161:T4, "Restarts Limits"=w1160:T3, "Run Profile"=w1102:bool, "Actual Starts"=w1159:T15, "Cog Limits:"=w1135:i32[], "Cog Events"=w1134:i32[], "CogCounters"=w1130:i32[], "Manual CMDs"=w1103:dbl[], "Stop Cmd"=w1133:dbl, "App Config.Pumps Present"=w1132:u32, "Tank Data"=w1120:dbl[], "Intitial Times"=w1119:dbl[], "App Config.Tank 1 Fuel"=w1124:string, "App Config.Tank 2 Fuel"=w1123:string, "App Config.Serial Numbers"=w1122:T31, "Controller.Invert PWM"=w1101:bool, "PS CMD"=w1098:dbl, "Press CMD"=w1099:dbl)  [unwired: 1 out]
        n450 = disable-structure shown="Enabled" {
          disable-tunnel: w1100 -> [w1169 w1177]
          disable-tunnel: [w1168 w1176] -> w1144
          disable-tunnel: w1101 -> [_ w1175]
          disable-tunnel: w1099 -> [_ w1172]
          disable-tunnel: w1098 -> [_ w1173]
          frame Disabled {
            n451 = xnode "Read/Write Control"("FPGA VI Reference In"=w1169) -> ("Detected Starts"=w1168)  [unwired: 1 in, 2 out]
          }
          frame Enabled {
            n452 = Not Equal To 0?(x=w1173) -> (x != 0?=w1174:bool)
            n453 = Divide(x=w1172, y=160.0) -> (x/y=w1171:dbl)
            n454 = xnode "Read/Write Control"("FPGA VI Reference In"=w1177, "InvertPWM"=w1175, "PS Control"=w1174, "AO0"=w1171) -> ("Actual Pump Starts"=w1176:u32[])  [unwired: 1 in, 2 out]
          }
        }
        n455 = local write "SubRoutine Profile"(w1094) -> ()
        n456 = local write "Stagger Time (ms):"(w1137) -> ()
        n457 = local write "Profile Name:"(w1105) -> ()
        n458 = local write "CA Number:"(w1104) -> ()
        n459 = local write "Controller Type:"(w1140) -> ()
        n460 = local write "Tank 1 Fuel Type"(w1124) -> ()
        n461 = local write "Tank 2 Fuel Type"(w1123) -> ()
        n462 = local write "Serial Numbers"(w1122) -> ()
        n463 = Equal?(x=w1103, y=w1133) -> (x = y?=w1149:bool[])
        n464 = feedback-in #1(w1149) -> ()
        n465 = feedback #1(w1149) -> (w1150:bool[])
        n466 = Less?(x=w1149, y=w1150) -> (x < y?=w1129:bool[])
        n467 = Number To Boolean Array(number=w1132) -> (Boolean array=w1121:bool[])
        n468 = disable-structure shown="Disabled" {
          disable-tunnel: w1105 -> [w1180 _]
          disable-tunnel: w1102 -> [w1179 _]
          frame Disabled {
            n469 = Select(t="running", s=w1179, f="idle") -> (s? t:f=w1183:string)
            n470 = Bundle By Name(cluster=T28 {"number"=0, "building"="", "room"="", "ipAddress"="", "profileName"="", "caNumber"="", "ctrlType"="", "mode"="", "channels"=[], "pumps"=[]} ("tank"), "profileName"=w1180, "mode"=w1183) -> (w1184:T28)
            n471 = call "JSON Global.vi"("Write (F)"=TRUE, "JSON In"=w1184) -> ()  [unwired: 9 in, 1 out]
          }
          frame Enabled {
          }
        }
        n472 = call "Signal Breakout.vi"("Pumps Enabled"=w1121, "Tank Data"=w1120, "Intitial Times"=w1119) -> ("Pump Data"=w1108:T19, "Tank Data"=w1107:T37, "Elapsed Time:"=w1095:dbl[])  [unwired: 10 in]
        n473 = call "Calculate Restarts.vi"("Restarts Cluster"=w1161, "Restarts Limits"=w1160, "Run Profile"=w1102, "Actual Starts"=w1159, "Actual Pump Starts (FPGA)"=w1144) -> ("Restarts Cluster OUT"=w1136:T4, "Restarts Alarm"=w1146:bool, "Restarts Limits OUT"=w1163:T3, "Actual Starts OUT"=w1162:T15)  [unwired: 7 in]
        "Restarts Cluster" <- w1136
        n474 = case shown="True" w1138 {
          tunnel: w1139 -> [_ w1192]
          frame False {
          }
          frame True {
            n475 = local write "Profile:"(w1192) -> ()
          }
        }
        n476 = local write "Restarts Limits"(w1163) -> ()
        n477 = Unbundle(w1108) -> ("Voltages"=→"Voltages":dbl[], "PumpCurrent"=→"PumpCurrent":dbl[], "Speed"=w1116:dbl[], "ControllerCurrent"=→"ControllerCurrent":dbl[], "Pressure"=→"Pressure":dbl[], "Flow"=w1113:dbl[], "Elapsed Time:"=→"Elapsed Time:":dbl[])
        "Speed" <- w1116
        "Flow" <- w1113
        n478 = Unbundle(w1107) -> ("PS Actual (V):"=→"PS Actual (V):":dbl, "Temp1"=→"Temp1":dbl, "Temp2"=→"Temp2":dbl)
        n479 = disable-structure shown="Disabled" {
          disable-tunnel: w1095 -> [w1178 _]
          frame Disabled {
            n480 = call "Elapsed Time Global.vi"("Ticks IN"=w1178) -> ()  [unwired: 10 in, 1 out]
          }
          frame Enabled {
          }
        }
        n481 = Boolean To (0,1)(Boolean=w1121) -> (0, 1=w1151:i16[])
        n482 = To Double Precision Float(number=w1151) -> (double precision float=w1131:dbl[])
        n483 = call "Pump Manual Commands.vi"("Write (F)"=TRUE, "Pumps Enabled IN"=w1121, "Manual CMDs IN"=w1103) -> ()  [unwired: 7 in, 2 out]
        n484 = call "Cog Detector.vi"("Cog Limits:"=w1135, "Cogs IN"=w1134, "Counters IN"=w1130, "Started"=w1129, "Pump Present"=w1121, "Flow"=w1113, "Run Profile"=w1102) -> ("Cogs OUT"=w1147:i32[], "Cog Alarm"=w1145:bool, "Counters OUT"=w1148:i32[])  [unwired: 6 in]
        "Cog Events:" <- w1147
        n485 = Array To Cluster(array=w1121) -> (cluster=w1128:T33)
        n486 = case shown="True" w1102 {
          tunnel: [w1187 w1189] -> w1165
          tunnel: w1164 -> [w1187 w1188]
          frame False {
          }
          frame True {
            n487 = Insert Into Array(array=w1188, index=0, new element=Sequence_States."Save Status") -> (w1189:T14[])
          }
        }
        n488 = Add Array Elements(numeric array=w1116) -> (sum=w1157:dbl)
        n489 = Add Array Elements(numeric array=w1131) -> (sum=w1155:dbl)
        n490 = local write "Pumps Present"(w1128) -> ()
        n491 = Equal To 0?(x=w1155) -> (x = 0?=w1156:bool)
        n492 = Select(t=1.0, s=w1156, f=w1155) -> (s? t:f=w1153:dbl)
        n493 = Divide(x=w1157, y=w1153) -> (x/y=→"Ave. Speed":dbl)
        n494 = Or(x=w1146, y=w1145) -> (x .or. y?=w1096:bool)
        n495 = Get Date/Time In Seconds() -> (seconds since 1Jan1904=w1127:timestamp)
        n496 = To Double Precision Float(number=w1127) -> (double precision float=w1126:dbl)
        n497 = Bundle By Name(cluster=w1167, "Last Update"=w1126, "Update Screen"=w1125, "Update Profile"=w1125, "Restarts Cluster"=w1136, "Alarm"=w1096, "Restart Alarm"=w1096, "Actual Starts"=w1162, "Pumps Present"=w1128, "Elapsed Times"=w1095, "Cog Events"=w1147, "CogCounters"=w1148) -> (w1097:T17)
        n498 = local write "pb.Resets"(w1166) -> ()
        n499 = local write "pb.Sets"(w1166) -> ()
      }
      frame "Stop Profile" {
        w1202 = T2 {"Pump 1"=FALSE, "Pump 2"=FALSE, "Pump 3"=FALSE, "Pump 4"=FALSE, "Pump 5"=FALSE, "Pump 6"=FALSE} ("Power Relay")
        w1203 = FALSE ("Run Profile")
        n500 = Unbundle By Name(w1199) -> ("App Config.Controller Type:"=w1197:T5, "App Config.PWM Freq (Hz)"=w1198:dbl)
        n501 = Divide(x=400000.0 ("y"), y=w1198) -> (x/y=w1201:dbl)
        n502 = case shown="\"Kuhnke\"" w1197 {
          tunnel: w1201 -> [_ w1216 w1220 w1224 w1228]
          tunnel: [0 w1215 w1219 w1223 w1227] -> w1193
          tunnel: [0.0 w1213 w1217 w1221 w1225] -> w1196
          frame Default {
          }
          frame "Kuhnke" {
            w1213 = 10.0 ("y")
            n503 = Multiply(x=w1216, y=w1213) -> (x*y=w1214:dbl)
            n504 = To Long Integer(number=w1214) -> (32bit integer=w1215:i32)
          }
          frame "PSA" {
            w1217 = 5.0 ("y")
            n505 = Multiply(x=w1220, y=w1217) -> (x*y=w1218:dbl)
            n506 = To Long Integer(number=w1218) -> (32bit integer=w1219:i32)
          }
          frame "8 Comm Hella", "10 Comm Hella" {
            w1221 = 80.0 ("y")
            n507 = Multiply(x=w1224, y=w1221) -> (x*y=w1222:dbl)
            n508 = To Long Integer(number=w1222) -> (32bit integer=w1223:i32)
          }
          frame "8 Comm Omron", "10 Comm Omron" {
            w1225 = 75.0 ("y")
            n509 = Multiply(x=w1228, y=w1225) -> (x*y=w1226:dbl)
            n510 = To Long Integer(number=w1226) -> (32bit integer=w1227:i32)
          }
        }
        n511 = Initialize Array(w1196, 6 ("dimension size")) -> (w1194:dbl[])
        n512 = disable-structure shown="Disabled" {
          disable-tunnel: w1208 -> [w1231 w1235]
          disable-tunnel: w1193 -> [_ w1234]
          frame Disabled {
            w1229 = fxp<+/-,20,5> 0.0 ("AO0")
            w1230 = 0 ("Duty (Ticks) 1")
            # "This was disabled before I started"
            # "Solenoid"
            n513 = xnode "Read/Write Control"("FPGA VI Reference In"=w1231, "Duty (Ticks) 1"=w1230, "Duty (Ticks) 2"=w1230, "Duty (Ticks) 3"=w1230, "Duty (Ticks) 4"=w1230, "Duty (Ticks) 5"=w1230, "Duty (Ticks) 6"=w1230, "AO0"=w1229, "AO1"=w1229) -> ()  [unwired: 1 in, 2 out]
          }
          frame Enabled {
            n514 = xnode "Read/Write Control"("FPGA VI Reference In"=w1235, "Duty (Ticks) 1"=w1234, "Duty (Ticks) 2"=w1234, "Duty (Ticks) 3"=w1234, "Duty (Ticks) 4"=w1234, "Duty (Ticks) 5"=w1234, "Duty (Ticks) 6"=w1234, "AO0"=fxp<+/-,20,5> 0.0, "PS Control"=FALSE) -> ()  [unwired: 1 in, 2 out]
          }
        }
        n515 = local write "pb.Run Profile"(w1203) -> ()
        n516 = Bundle By Name(cluster=w1199, "Run Profile"=w1203, "Manual CMDs"=w1194, "Last CMDs"=w1194, "Power Relay"=w1202, "Ignition Relay"=w1202) -> (w1210:T17)
        n517 = local write "Power Relay"(w1202) -> ()
        n518 = local write "Ignition Relay"(w1202) -> ()
        n519 = local write "Manual\nCMD"(w1194) -> ()
        n520 = property on="Main Tab" class="TabCtl (strict)"("DisabledEnum"=T27."Enabled" ("Disabled")) -> ()  [unwired: 2 in, 2 out]
        n521 = Insert Into Array(array=w1206, index=0, new element=Sequence_States."Set Manual CMD") -> (w1204:T14[])
      }
      frame "Save As" {
        n522 = property on="Save As Tab" class="TabCtl (strict)"("Visible"=TRUE) -> (error out=w1236:errorcluster)  [unwired: 2 in, 1 out]
        n523 = while {
          tunnel: ["pb.Save As OK"] -> w1243
          tunnel: w1236 -> [_]
          stop <- w1245 stop-if-true
          n524 = Wait (ms)(milliseconds to wait=u32 10) -> ()  [unwired: 1 out]
          n525 = Or(x="pb.Save As OK", y="pb.Save As Cancel") -> (x .or. y?=w1245:bool)
        }
        n526 = Unbundle By Name(w1240) -> ("App Config.Profiles Path"=w1242:path, "Profile"=w1238:string[][])
        n527 = case shown="True" w1243 {
          tunnel: w1242 -> [_ w1253]
          tunnel: [w1248 w1250] -> w1241
          tunnel: w1240 -> [w1249 w1255]
          tunnel: [w1249 w1254] -> w1239
          tunnel: w1238 -> [_ w1252]
          frame False {
            w1248 = T14[] [enum."Enable Background"] items=["Main", "Init Files", "Init", "Save As", "Start Profile", "Check Step Time", "Alarm", "Run Step", "Stop Profile", "Cycle Reset", "Time Reset", "Time Reset All", "Time Set", "Tare CTs", "Save Profile", "Open Profile", "Get Profiles", "Update Screen", "Save Status", "Set Manual CMD", "Reset Restarts", "Reset Total Restarts", "Reset Cogs", "Disable Background", "Enable Background", "Get/Release Control", "Init AKLH", "Save AKLH", "Log Fuel Change", "Update Data Stream", "Init TenHz", "Read TenHz", "Remote Timer Reset", "Record Frequency Change", "Controller Change", "Get Alarms", "Init Alarms", "Save Alarms", "Init SubRoutine", "Next SubRoutine"]
          }
          frame True {
            w1250 = T14[] [enum."Enable Background", enum."Get Profiles"] items=["Main", "Init Files", "Init", "Save As", "Start Profile", "Check Step Time", "Alarm", "Run Step", "Stop Profile", "Cycle Reset", "Time Reset", "Time Reset All", "Time Set", "Tare CTs", "Save Profile", "Open Profile", "Get Profiles", "Update Screen", "Save Status", "Set Manual CMD", "Reset Restarts", "Reset Total Restarts", "Reset Cogs", "Disable Background", "Enable Background", "Get/Release Control", "Init AKLH", "Save AKLH", "Log Fuel Change", "Update Data Stream", "Init TenHz", "Read TenHz", "Remote Timer Reset", "Record Frequency Change", "Controller Change", "Get Alarms", "Init Alarms", "Save Alarms", "Init SubRoutine", "Next SubRoutine"]
            n528 = call "Save Profile.vi"("Profile"=w1252, "Current Profile"="New Profile Name:", "Profiles Path"=w1253) -> ()  [unwired: 8 in, 1 out]
            n529 = Bundle By Name(cluster=w1255, "App Config.Current Profile"="New Profile Name:") -> (w1254:T17)
          }
        }
      }
      frame "Save Status" {
        # "Was getting stuck in a loop where I had not set my frequency so had to\nmake sure I was not recording on startup, probably could remove this now"
        n530 = Unbundle By Name(w1262) -> ("App Config"=w1274:T16, "Restarts Cluster.CMD Starts:"=w1282:i32[], "Actual Starts.Actual Pump Starts"=w1281:i32[], "Restarts Limits.High Limits:"=w1280:i32[], "Restarts Limits.Low Limits:"=w1279:i32[], "Restarts Cluster.Total CMD:"=w1278:i32[], "Actual Starts.Tot Act Starts"=w1277:i32[], "Elapsed Times"=w1259:dbl[], "CT Offsets"=w1290:fxp<+/-,26,7>[], "Cog Events"=w1276:i32[], "Cog Limits:"=w1275:i32[], "SubRoutine Profile"=w1265:i32[][])
        n531 = Bundle By Name(cluster=w1274, "Record TenHz"=FALSE) -> (w1273:T16)
        n532 = call <vilib>:"Open Config Data.vi"("create file if necessary (T)"=TRUE, "configuration file path"=path "c:/App Config.ini") -> ("error out"=w1300:errorcluster, "refnum"=w1304:T35)  [unwired: 7 in, 1 out]
        n533 = Build Array(w1282, w1281, w1280, w1279, w1278, w1277, w1276, w1275) -> (w1298:i32[][])
        n534 = To Double Precision Float(number=w1290) -> (double precision float=w1289:dbl[])
        n535 = Delete From Array(array=w1265, length=20, index (col)=2 ("disabled index (col)")) -> (array with subset deleted=w1260:i32[][])  [unwired: 1 in, 1 out]
        n536 = call "Read Write App Config.vi"("Write (F)"=TRUE, "Error IN"=w1300, "App Config IN"=w1273, "Refnum in"=w1304) -> ("Error OUT"=w1302:errorcluster, "Refnum out"=w1303:T35)  [unwired: 5 in, 1 out]
        n537 = Array To Spreadsheet String(delimiter (Tab)=",", array=w1298, 3:"%d" ("format string")) -> (spreadsheet string=w1295:string)
        n538 = Array To Spreadsheet String(delimiter (Tab)=",", array=w1289, 3:"%.2f" ("format string")) -> (spreadsheet string=w1287:string)
        n539 = Array To Spreadsheet String(delimiter (Tab)=",", array=w1260, 3:"%g" ("format string")) -> (spreadsheet string=w1269:string)
        n540 = call <vilib>:"Close Config Data.vi"("error in (no error)"=w1302, "refnum"=w1303) -> ()  [unwired: 8 in, 2 out]
        n541 = Write to Text File(file (use dialog)=path "c:/Restarts", text=w1295) -> (refnum out=w1286:refnum<file>, error out=w1285:errorcluster)  [unwired: 2 in, 1 out]
        n542 = Write to Text File(file (use dialog)=path "c:/CT Offsets", text=w1287) -> (refnum out=w1284:refnum<file>, error out=w1283:errorcluster)  [unwired: 2 in, 1 out]
        n543 = Write to Text File(file (use dialog)=path "c:/SubRoutine", text=w1269) -> (refnum out=w1270:refnum<file>, error out=w1271:errorcluster)  [unwired: 2 in, 1 out]
        n544 = Array Size(array=w1259) -> (size(s)=w1258:i32)
        n545 = Close File(refnum=w1286, error in=w1285) -> ()  [unwired: 2 out]
        n546 = Close File(refnum=w1284, error in=w1283) -> ()  [unwired: 2 out]
        n547 = Close File(refnum=w1270, error in=w1271) -> ()  [unwired: 2 out]
        n548 = Equal?(x=w1258, y=6) -> (x = y?=w1256:bool)
        n549 = case shown="True" w1256 {
          tunnel: w1259 -> [_ w1306]
          frame False {
          }
          frame True {
            n550 = Write to Binary File(file (use dialog)=path "c:/ElapsedTimes", data=w1306) -> (refnum out=w1308:refnum<file>, error out=w1307:errorcluster)  [unwired: 4 in, 1 out]
            n551 = Close File(refnum=w1308, error in=w1307) -> ()  [unwired: 2 out]
          }
        }
        n552 = Bundle By Name(cluster=w1262, "SubRoutine Profile"=w1260) -> (w1261:T17)
      }
      frame "Disable Background" {
        w1310 = T27."Disabled and Grayed Out" ("Disabled")
        n553 = property on="Main Tab" class="TabCtl (strict)"("DisabledEnum"=w1310) -> ()  [unwired: 2 in, 2 out]
        n554 = property on="pb.Stop Profile" class="Bool"("DisabledEnum"=w1310) -> ()  [unwired: 2 in, 2 out]
        n555 = property on="Restarts Tab" class="TabCtl (strict)"("DisabledEnum"=w1310) -> ()  [unwired: 2 in, 2 out]
        n556 = property on="Monitoring Tab" class="TabCtl (strict)"("DisabledEnum"=w1310) -> ()  [unwired: 2 in, 2 out]
        n557 = property on="Title Tab" class="TabCtl (strict)"("DisabledEnum"=w1310) -> ()  [unwired: 2 in, 2 out]
        n558 = property on="CPU Usage:" class="DigNum (strict)"("DisabledEnum"=w1310) -> ()  [unwired: 2 in, 2 out]
      }
      frame "Enable Background" {
        w1313 = FALSE ("Visible")
        w1314 = T27."Enabled" ("Disabled")
        n559 = xnode "Read/Write Control"("FPGA VI Reference In"=w1320, "Timer Resets"=bool[] [FALSE, FALSE, FALSE, FALSE, FALSE, FALSE] ("array")) -> ()  [unwired: 1 in, 2 out]
        n560 = property on="Save As Tab" class="TabCtl (strict)"("Visible"=w1313) -> ()  [unwired: 2 in, 2 out]
        n561 = property on="Reset Tab" class="TabCtl (strict)"("Visible"=w1313) -> ()  [unwired: 2 in, 2 out]
        n562 = property on="Set Time Tab" class="TabCtl (strict)"("Visible"=w1313) -> ()  [unwired: 2 in, 2 out]
        n563 = property on="Alarm Tab" class="TabCtl (strict)"("Visible"=w1313) -> ()  [unwired: 2 in, 2 out]
        n564 = property on="Main Tab" class="TabCtl (strict)"("DisabledEnum"=w1314) -> ()  [unwired: 2 in, 2 out]
        n565 = property on="pb.Stop Profile" class="Bool"("DisabledEnum"=w1314) -> ()  [unwired: 2 in, 2 out]
        n566 = property on="Restarts Tab" class="TabCtl (strict)"("DisabledEnum"=w1314) -> ()  [unwired: 2 in, 2 out]
        n567 = property on="Monitoring Tab" class="TabCtl (strict)"("DisabledEnum"=w1314) -> ()  [unwired: 2 in, 2 out]
        n568 = property on="Title Tab" class="TabCtl (strict)"("DisabledEnum"=w1314) -> ()  [unwired: 2 in, 2 out]
        n569 = property on="CPU Usage:" class="DigNum (strict)"("DisabledEnum"=w1314) -> ()  [unwired: 2 in, 2 out]
        n570 = property on="Alarm Tab" class="TabCtl (strict)"("DisabledEnum"=w1314) -> ()  [unwired: 2 in, 2 out]
        n571 = Insert Into Array(array=w1318, index=0, new element=Sequence_States."Update Screen") -> (w1317:T14[])
      }
      frame "Cycle Reset".."Time Reset All", "Reset Restarts".."Reset Cogs" {
        w1324 = T14[] [enum."Enable Background"] items=["Main", "Init Files", "Init", "Save As", "Start Profile", "Check Step Time", "Alarm", "Run Step", "Stop Profile", "Cycle Reset", "Time Reset", "Time Reset All", "Time Set", "Tare CTs", "Save Profile", "Open Profile", "Get Profiles", "Update Screen", "Save Status", "Set Manual CMD", "Reset Restarts", "Reset Total Restarts", "Reset Cogs", "Disable Background", "Enable Background", "Get/Release Control", "Init AKLH", "Save AKLH", "Log Fuel Change", "Update Data Stream", "Init TenHz", "Read TenHz", "Remote Timer Reset", "Record Frequency Change", "Controller Change", "Get Alarms", "Init Alarms", "Save Alarms", "Init SubRoutine", "Next SubRoutine"]
        n572 = property on="Reset Tab" class="TabCtl (strict)"("Visible"=TRUE) -> (error out=w1325:errorcluster)  [unwired: 2 in, 1 out]
        n573 = while {
          tunnel: ["pb.Reset OK"] -> w1332
          tunnel: w1325 -> [_]
          stop <- w1335 stop-if-true
          n574 = Wait (ms)(milliseconds to wait=u32 10) -> ()  [unwired: 1 out]
          n575 = Or(x="pb.Reset Cancel", y="pb.Reset OK") -> (x .or. y?=w1335:bool)
        }
        n576 = Unbundle By Name(w1323) -> ("pb.Resets"=w1331:bool[], "Intitial Times"=w1328:dbl[])
        n577 = Search 1D Array(1D array=w1331, element=TRUE) -> (index of element=w1329:i32)  [unwired: 1 in]
        n578 = case shown="True" w1332 {
          tunnel: [w1338 w1345] -> w1333
          tunnel: w1323 -> [w1338 w1344]
          tunnel: w1329 -> [_ w1343]
          tunnel: w1328 -> [_ w1342]
          tunnel: w1327 -> [_ w1341]
          tunnel: w1323 -> [_ w1340]
          tunnel: w1322 -> [_ w1339]
          frame False {
          }
          frame True {
            n579 = case shown="\"Reset Restarts\"" w1339 {
              tunnel: w1344 -> [w1348 w1360 w1367 w1376 w1391 w1400]
              tunnel: [w1347 w1359 w1366 w1375 w1390 w1399] -> w1345
              tunnel: w1343 -> [_ w1355 _ _ _ _]
              tunnel: w1342 -> [_ w1358 _ _ _ _]
              tunnel: w1341 -> [_ w1353 w1365 w1374 w1389 _]
              tunnel: w1340 -> [_ _ _ w1372 w1387 _]
              frame "Cycle Reset", Default {
                n580 = Bundle By Name(cluster=w1348, "App Config.Cycles Completed"=u32 0) -> (w1347:T17)
              }
              frame "Time Reset" {
                n581 = Replace Array Subset(array=w1358, new element=0.0 ("new element/subarray"), index=w1355) -> (w1349:dbl[])
                n582 = Replace Array Subset(array=bool[] [FALSE, FALSE, FALSE, FALSE, FALSE, FALSE], new element=TRUE ("new element/subarray"), index=w1355) -> (w1356:bool[])
                n583 = xnode "Read/Write Control"("FPGA VI Reference In"=w1353, "Timer Resets"=w1356) -> ()  [unwired: 1 in, 2 out]
                n584 = Bundle By Name(cluster=w1360, "Intitial Times"=w1349) -> (w1359:T17)
                n585 = call "Elapsed Time Global.vi"("Write (F)"=TRUE, "Tick Divider"=1.0, "Initial Times IN"=w1349) -> ()  [unwired: 8 in, 1 out]
              }
              frame "Time Reset All" {
                w1361 = dbl[] [0.0, 0.0, 0.0, 0.0, 0.0, 0.0] ("Intitial Times")
                n586 = xnode "Read/Write Control"("FPGA VI Reference In"=w1365, "Timer Resets"=bool[] [TRUE, TRUE, TRUE, TRUE, TRUE, TRUE] ("array")) -> ()  [unwired: 1 in, 2 out]
                n587 = Bundle By Name(cluster=w1367, "Intitial Times"=w1361) -> (w1366:T17)
                n588 = call "Elapsed Time Global.vi"("Write (F)"=TRUE, "Tick Divider"=1.0, "Initial Times IN"=w1361) -> ()  [unwired: 8 in, 1 out]
              }
              frame "Reset Restarts" {
                w1373 = i32[] [0, 0, 0, 0, 0, 0] ("CMD Starts")
                n589 = disable-structure shown="Enabled" {
                  disable-tunnel: w1374 -> [w1379 w1382]
                  disable-tunnel: TRUE ("Reset") -> [w1378 w1380]
                  disable-tunnel: [w1377 w1381] -> w1368
                  frame Disabled {
                    n590 = xnode "Read/Write Control"("FPGA VI Reference In"=w1379, "Reset Starts"=w1378) -> ("Detected Starts"=w1377)  [unwired: 1 in, 2 out]
                  }
                  frame Enabled {
                    n591 = xnode "Read/Write Control"("FPGA VI Reference In"=w1382, "Reset"=w1380) -> ("Actual Pump Starts"=w1381:u32[])  [unwired: 1 in, 2 out]
                  }
                }
                n592 = Unbundle By Name(w1372) -> ("Actual Starts.Tot Init Act Starts"=w1369:i32[])
                n593 = Add(x=w1369, y=w1368) -> (x+y=w1371:u32[])
                n594 = Bundle By Name(cluster=w1376, "Restarts Cluster.CMD Starts:"=w1373, "Actual Starts.Actual Pump Starts"=w1373, "Actual Starts.Initial Actual Starts"=w1373, "Actual Starts.Tot Init Act Starts"=w1371) -> (w1375:T17)
              }
              frame "Reset Total Restarts" {
                w1388 = i32[] [0, 0, 0, 0, 0, 0] ("CMD Starts")
                n595 = Unbundle By Name(w1387) -> ("Actual Starts.Initial Actual Starts"=w1383:i32[])
                n596 = disable-structure shown="Enabled" {
                  disable-tunnel: w1389 -> [w1394 w1397]
                  disable-tunnel: TRUE ("Reset") -> [w1393 w1396]
                  disable-tunnel: [w1392 w1395] -> w1384
                  frame Disabled {
                    n597 = xnode "Read/Write Control"("FPGA VI Reference In"=w1394, "Reset Starts"=w1393) -> ("Detected Starts"=w1392)  [unwired: 1 in, 2 out]
                  }
                  frame Enabled {
                    n598 = xnode "Read/Write Control"("FPGA VI Reference In"=w1397, "Reset"=w1396) -> ("Actual Pump Starts"=w1395:u32[])  [unwired: 1 in, 2 out]
                  }
                }
                n599 = Add(x=w1383, y=w1384) -> (x+y=w1386:u32[])
                n600 = Bundle By Name(cluster=w1391, "Restarts Cluster.Total CMD:"=w1388, "Actual Starts.Tot Act Starts"=w1388, "Actual Starts.Tot Init Act Starts"=w1388, "Actual Starts.Initial Actual Starts"=w1386) -> (w1390:T17)
              }
              frame "Reset Cogs" {
                n601 = Bundle By Name(cluster=w1400, "Cog Events"=i32[] [0, 0, 0, 0, 0, 0]) -> (w1399:T17)
              }
            }
          }
        }
      }
      frame "Alarm" {
        w1418 = T14[] [enum."Enable Background"] items=["Main", "Init Files", "Init", "Save As", "Start Profile", "Check Step Time", "Alarm", "Run Step", "Stop Profile", "Cycle Reset", "Time Reset", "Time Reset All", "Time Set", "Tare CTs", "Save Profile", "Open Profile", "Get Profiles", "Update Screen", "Save Status", "Set Manual CMD", "Reset Restarts", "Reset Total Restarts", "Reset Cogs", "Disable Background", "Enable Background", "Get/Release Control", "Init AKLH", "Save AKLH", "Log Fuel Change", "Update Data Stream", "Init TenHz", "Read TenHz", "Remote Timer Reset", "Record Frequency Change", "Controller Change", "Get Alarms", "Init Alarms", "Save Alarms", "Init SubRoutine", "Next SubRoutine"]
        n602 = Unbundle By Name(w1402) -> ("Alarm Message"=w1413:string, "Restart Alarm"=w1412:bool, "App Config.Location"=w1405:string, "Restarts Cluster.CMD Starts:"=w1406:i32[], "Restarts Cluster.Restarts:"=w1407:i32[], "Restarts Limits.High Limits:"=w1408:i32[], "Restarts Limits.Low Limits:"=w1409:i32[], "Cog Events"=w1410:i32[], "Cog Limits:"=w1411:i32[], "App Config.Inform"=w1414:string)
        n603 = case shown="False" w1412 {
          tunnel: w1405 -> [w1421 w1432]
          tunnel: w1406 -> [_ w1431]
          tunnel: w1407 -> [_ w1430]
          tunnel: w1408 -> [_ w1429]
          tunnel: w1409 -> [_ w1428]
          tunnel: w1410 -> [_ w1427]
          tunnel: w1411 -> [_ w1426]
          tunnel: [w1422 "A pump event has occured.  Either a pump has had too many restarts, is cogging, or a fuse/breaker is tripped.  The test has been terminated.  Reset the restarts monitor in order to start the test again.  You may want to log the restarts before you reset!" ("Alarm Message")] -> w1404
          tunnel: w1413 -> [w1422 _]
          tunnel: [w1419 w1424] -> w1415
          tunnel: [w1422 w1423] -> w1416
          frame False {
            n604 = Concatenate Strings(w1421, " ALARM!" ("string")) -> (w1419:string)
          }
          frame True {
            n605 = call "Restart Alarm Message.vi"("Location"=w1432, "CMD Starts:"=w1431, "Restarts:"=w1430, "High Limits:"=w1429, "Low Limits:"=w1428, "Cog Events"=w1427, "Cog Limits:"=w1426) -> ("Subject:"=w1424:string, "Message:"=w1423:string)  [unwired: 11 in]
          }
        }
        n606 = call "Email to Handler.vi"("Email Handler IP"="34", "Message:"=w1416, "Subject:"=w1415, "To:"=w1414) -> ()  [unwired: 8 in]
        n607 = while {
          tunnel: w1404 -> [w1433]
          stop <- "pb.Alarm OK" stop-if-true
          n608 = flat-sequence {
            tunnel: w1433 -> [w1436]
            frame #0 {
              "Alarm Message" <- w1436
            }
            frame #1 {
              n609 = property on="Alarm Tab" class="TabCtl (strict)"("Visible"=TRUE) -> ()  [unwired: 2 in, 2 out]
            }
          }
          n610 = Wait (ms)(milliseconds to wait=u32 20) -> ()  [unwired: 1 out]
        }
        n611 = Bundle By Name(cluster=w1402, "Restart Alarm"=FALSE) -> (w1401:T17)
      }
      frame "Time Set" {
        w1438 = T14[] [enum."Enable Background"] items=["Main", "Init Files", "Init", "Save As", "Start Profile", "Check Step Time", "Alarm", "Run Step", "Stop Profile", "Cycle Reset", "Time Reset", "Time Reset All", "Time Set", "Tare CTs", "Save Profile", "Open Profile", "Get Profiles", "Update Screen", "Save Status", "Set Manual CMD", "Reset Restarts", "Reset Total Restarts", "Reset Cogs", "Disable Background", "Enable Background", "Get/Release Control", "Init AKLH", "Save AKLH", "Log Fuel Change", "Update Data Stream", "Init TenHz", "Read TenHz", "Remote Timer Reset", "Record Frequency Change", "Controller Change", "Get Alarms", "Init Alarms", "Save Alarms", "Init SubRoutine", "Next SubRoutine"]
        n612 = Unbundle By Name(w1448) -> ("pb.Sets"=w1447:bool[], "Intitial Times"=w1442:dbl[], "Elapsed Times"=w1445:dbl[])
        n613 = Search 1D Array(1D array=w1447, element=TRUE) -> (index of element=w1444:i32)  [unwired: 1 in]
        n614 = Index Array(array=w1445, index=w1444) -> (element=w1443:dbl)
        n615 = local write "New Time"(w1443) -> ()
        n616 = property on="Set Time Tab" class="TabCtl (strict)"("Visible"=TRUE) -> (error out=w1439:errorcluster)  [unwired: 2 in, 1 out]
        n617 = while {
          tunnel: ["pb.Set Time OK"] -> w1450
          tunnel: w1443 -> [_]
          tunnel: w1439 -> [_]
          stop <- w1453 stop-if-true
          n618 = Wait (ms)(milliseconds to wait=u32 10) -> ()  [unwired: 1 out]
          n619 = Or(x="pb.Set Time Cancel", y="pb.Set Time OK") -> (x .or. y?=w1453:bool)
        }
        n620 = case shown="True" w1450 {
          tunnel: w1448 -> [w1455 w1461]
          tunnel: [w1455 w1460] -> w1449
          tunnel: w1444 -> [_ w1457]
          tunnel: w1442 -> [_ w1459]
          tunnel: w1441 -> [_ w1458]
          frame False {
          }
          frame True {
            n621 = xnode "Read/Write Control"("FPGA VI Reference In"=w1458) -> ("FPGA VI Reference Out"=w1464:refnum<k20>, "Timer Resets"=w1465:bool[])  [unwired: 1 in, 1 out]
            n622 = Replace Array Subset(array=w1459, new element="New Time", index=w1457) -> (w1466:dbl[])
            n623 = Replace Array Subset(array=w1465, new element=TRUE ("new element/subarray"), index=w1457) -> (w1463:bool[])
            n624 = Bundle By Name(cluster=w1461, "Intitial Times"=w1466) -> (w1460:T17)
            n625 = xnode "Read/Write Control"("FPGA VI Reference In"=w1464, "Timer Resets"=w1463) -> ()  [unwired: 1 in, 2 out]
          }
        }
      }
      frame "Remote Timer Reset" {
        n626 = disable-structure shown="Enabled" {
          disable-tunnel: w1467 -> [w1487 _]
          disable-tunnel: [w1477 w1497] -> w1470
          disable-tunnel: w1469 -> [w1476 w1496]
          disable-tunnel: w1467 -> [w1471 w1492]
          frame Disabled {
            # "Reset individual timer."
            n627 = Unbundle By Name(w1487) -> ("Intitial Times"=w1483:dbl[], "pb.Resets"=w1485:bool[])
            n628 = Search 1D Array(1D array=w1485, element=TRUE) -> (index of element=w1479:i32)  [unwired: 1 in]
            n629 = Replace Array Subset(array=bool[] [FALSE, FALSE, FALSE, FALSE, FALSE, FALSE] ("pb.Resets"), new element=TRUE ("new element/subarray"), index=w1479) -> (w1475:bool[])
            n630 = Replace Array Subset(array=w1483, new element=0.0 ("new element/subarray"), index=w1479) -> (w1481:dbl[])
            n631 = xnode "Read/Write Control"("FPGA VI Reference In"=w1476, "Timer Resets"=w1475) -> ("FPGA VI Reference Out"=w1473:refnum<k20>)  [unwired: 1 in, 1 out]
            n632 = Bundle By Name(cluster=w1471, "pb.Resets"=bool[] [FALSE, FALSE, FALSE, FALSE, FALSE, FALSE], "Intitial Times"=w1481) -> (w1477:T17)
            n633 = flat-sequence {
              tunnel: w1473 -> [w1488]
              tunnel: [w1488] -> w1472
              frame #0 {
                n634 = Wait (ms)(milliseconds to wait=u32 20) -> ()  [unwired: 1 out]
              }
            }
            n635 = xnode "Read/Write Control"("FPGA VI Reference In"=w1472, "Timer Resets"=bool[] [FALSE, FALSE, FALSE, FALSE, FALSE, FALSE] ("pb.Resets")) -> ()  [unwired: 1 in, 2 out]
          }
          frame Enabled {
            n636 = xnode "Read/Write Control"("FPGA VI Reference In"=w1496, "Timer Resets"=bool[] [TRUE, TRUE, TRUE, TRUE, TRUE, TRUE] ("pb.Resets")) -> ("FPGA VI Reference Out"=w1494:refnum<k20>)  [unwired: 1 in, 1 out]
            n637 = Bundle By Name(cluster=w1492, "Intitial Times"=dbl[] [0.0, 0.0, 0.0, 0.0, 0.0, 0.0]) -> (w1497:T17)
            n638 = flat-sequence {
              tunnel: w1494 -> [w1498]
              tunnel: [w1498] -> w1493
              frame #0 {
                n639 = Wait (ms)(milliseconds to wait=u32 20) -> ()  [unwired: 1 out]
              }
            }
            n640 = xnode "Read/Write Control"("FPGA VI Reference In"=w1493, "Timer Resets"=bool[] [FALSE, FALSE, FALSE, FALSE, FALSE, FALSE] ("pb.Resets")) -> ()  [unwired: 1 in, 2 out]
          }
        }
      }
      frame "Set Manual CMD" {
        w1511 = 10.0 ("y")
        w1526 = fxp<+/-,20,5> 0.0 ("AO0")
        n641 = Unbundle By Name(w1525) -> ("App Config.Controller Type:"=w1531:T5, "App Config.PWM Freq (Hz)"=w1532:dbl, "Manual CMDs"=w1530:dbl[], "PS CMD"=w1517:dbl, "Press CMD"=w1520:dbl, "App Config.VoltCtrlRef"=w1516:string)  [unwired: 1 out]
        n642 = Divide(x=w1517, y=10.0) -> (x/y=w1524:dbl)
        n643 = Divide(x=w1520, y=165.0) -> (x/y=w1521:dbl)
        n644 = To Fixed-Point(fixed-point type=w1526, number=w1524) -> (fixed-point=w1527:fxp<+/-,20,5>)
        n645 = To Fixed-Point(fixed-point type=w1526, number=w1521) -> (fixed-point=w1528:fxp<+/-,20,5>)
        n646 = case shown="\"Kuhnke\", \"PSA\", Default" w1531 {
          selector: w1531 -> [w1543 _]
          tunnel: w1519 -> [w1557 _]
          tunnel: w1532 -> [w1541 _]
          tunnel: w1530 -> [w1556 w1564]
          frame "Kuhnke", "PSA", Default {
            n647 = disable-structure shown="Enabled" {
              disable-tunnel: w1543 -> [w1559 _]
              disable-tunnel: [w1558 w1562] -> w1542
              disable-tunnel: w1541 -> [_ w1562]
              frame Disabled {
                n648 = case shown="\"Kuhnke\", Default" w1559 {
                  tunnel: [100.0 ("y") 150.0 ("y")] -> w1558
                  frame "Kuhnke", Default {
                  }
                  frame "PSA" {
                  }
                }
              }
              frame Enabled {
              }
            }
            n649 = Divide(x=40000000.0 ("40 MHz"), y=w1542) -> (x/y=w1548:dbl)
            n650 = Multiply(x=w1548, y=w1556) -> (x*y=w1544:dbl[])
            n651 = Divide(x=w1544, y=100.0 ("%")) -> (x/y=w1546:dbl[])
            n652 = To Long Integer(number=w1546) -> (32bit integer=w1555:i32[])
            n653 = Index Array(array=w1555) -> (element #1=w1554:i32, element #2=w1553:i32, element #3=w1552:i32, element #4=w1551:i32, element #5=w1550:i32, element #6=w1549:i32)  [unwired: 6 in]
            n654 = xnode "Read/Write Control"("FPGA VI Reference In"=w1557, "Duty (Ticks) 1"=w1554, "Duty (Ticks) 2"=w1553, "Duty (Ticks) 3"=w1552, "Duty (Ticks) 4"=w1551, "Duty (Ticks) 5"=w1550, "Duty (Ticks) 6"=w1549) -> ()  [unwired: 1 in, 2 out]
          }
          frame "Conti" {
            n655 = Index Array(array=w1564) -> (element=→"CAN CMD":dbl)  [unwired: 1 in]
          }
        }
        n656 = Not Equal To 0?(x=w1527) -> (x != 0?=w1510:bool)
        n657 = Multiply(x="1 Pulse Duty%", y=w1511) -> (x*y=w1508:dbl)
        n658 = Multiply(x="2 Pulse Duty%", y=w1511) -> (x*y=w1507:dbl)
        n659 = Multiply(x="3 Pulse Duty%", y=w1511) -> (x*y=w1506:dbl)
        n660 = xnode "Read/Write Control"("FPGA VI Reference In"=w1519, "PS Control"=w1510, "AO0"=w1528, "Pulse Frequency"="Pulse Frequency", "Module 1 Pulse Duty"=w1508, "Module 2 Pulse Duty"=w1507, "Module 3 Pulse Duty"=w1506, "Mod1 Pulsing?"="1 Pulsing", "Mod1 On?"="Solenoid 1", "Mod2 Pulsing?"="2 Pulsing", "Mod2 On?"="Solenoid 2", "Mod3 Pulsing?"="3 Pulsing", "Mod3 On?"="Solenoid 3") -> ("error out"=w1518:errorcluster)  [unwired: 1 in, 1 out]
        n661 = Empty String/Path?(string/path=w1516) -> (empty?=w1515:bool)
        n662 = case shown="False" w1515 {
          tunnel: w1518 -> [_ w1536]
          tunnel: w1517 -> [_ w1534]
          tunnel: w1516 -> [_ w1533]
          frame True {
          }
          frame False {
            n663 = shared-variable-open(w1533, w1536, 0.0) -> (w1540:refnum<k21>, w1537:errorcluster)  [unwired: 1 in]
            n664 = shared-variable-write(w1540, w1537, w1534) -> (w1539:refnum<k21>, w1538:errorcluster)
            n665 = Close Variable Connection(8:w1538, 11:w1539) -> ()  [unwired: 1 out]
          }
        }
      }
      frame "Get/Release Control" {
        n666 = Unbundle By Name(w1569) -> ("Login"=w1566:bool)
        n667 = case shown="True" w1566 {
          tunnel: [T27."Disabled" ("Disabled") T27."Enabled" ("Disabled")] -> w1568
          frame False {
          }
          frame True {
          }
        }
        n668 = local write "Main Tab"(enum32{"Main", "Data Stream", "Alarms"}."Main" ("Main Tab")) -> ()
        n669 = property on="Main Tab" class="TabCtl (strict)"("DisabledEnum"=w1568) -> ()  [unwired: 2 in, 2 out]
        n670 = property on="pb.Stop Profile" class="Bool"("DisabledEnum"=w1568) -> ()  [unwired: 2 in, 2 out]
        n671 = property on="Restarts Tab" class="TabCtl (strict)"("DisabledEnum"=w1568) -> ()  [unwired: 2 in, 2 out]
        n672 = property on="Monitoring Tab" class="TabCtl (strict)"("DisabledEnum"=w1568) -> ()  [unwired: 2 in, 2 out]
      }
      frame "Init AKLH" {
        w1582 = " " ("string")
        n673 = Unbundle By Name(w1589) -> ("AKLH Path"=w1587:path, "App Config.Location"=w1584:string, "App Config.CA Number"=w1583:string)
        n674 = Get Date/Time In Seconds() -> (seconds since 1Jan1904=w1573:timestamp)
        n675 = call "Timestamp2DayofYear.vi"("time stamp"=w1573) -> ("time string"=w1581:string)  [unwired: 14 in]
        n676 = Concatenate Strings("Continuous Monitoring " ("string"), w1584, w1582, w1583, w1582, w1581) -> (w1576:string)
        n677 = Strip Path(path=w1587) -> (stripped path=w1586:path)  [unwired: 1 out]
        n678 = Concatenate Strings(w1576, ".csv" ("string")) -> (w1577:string)
        n679 = Build Path(base path=w1586, name or relative path=w1577) -> (appended path=w1580:path)
        n680 = for {
          N: 10 -> [_]
          shift-right: [w1603] -> w1574
          shift-left: w1580 -> [w1605]
          tunnel: w1576 -> [w1600]
          tunnel: [w1598] -> w1575
          i -> [w1602]
          stop <- w1598 continue-if-true
          n681 = call <vilib>:"Check if File or Folder Exists.vi"("path"=w1605) -> ("file or folder exists?"=w1598:bool, "dup path"=w1604:path)  [unwired: 8 in, 1 out]
          n682 = Add(x=2, y=w1602) -> (x+y=w1599:i32)
          n683 = case shown="True" w1598 {
            tunnel: w1604 -> [w1611 w1613]
            tunnel: [w1606 w1613] -> w1603
            tunnel: w1600 -> [w1609 _]
            tunnel: w1599 -> [w1608 _]
            frame True {
              n684 = Strip Path(path=w1611) -> (stripped path=w1612:path)  [unwired: 1 out]
              n685 = Format Into String(format string="%s_%d.csv", w1609, w1608) -> (resulting string=w1607:string)  [unwired: 2 in, 1 out]
              n686 = Build Path(base path=w1612, name or relative path=w1607) -> (appended path=w1606:path)
            }
            frame False {
            }
          }
        }
        n687 = To Double Precision Float(number=w1573) -> (double precision float=w1572:dbl)
        n688 = case shown="False" w1575 {
          tunnel: [w1592 w1597] -> w1590
          tunnel: w1574 -> [w1592 w1594]
          frame True {
          }
          frame False {
            w1593 = string[] ["Time", "Cycles Completed", "Current Step", "PS Voltage (V)", "Tank 1 Temp (C)", "Tank 1 Fuel Type", "Position 1 Serial Number", "Position 1 Elapsed On Time", "Position 1 Controller Current (Adc)", "Position 1 Pump Current (Arms)", "Position 1 Pressure (kPa)", "Position 1 Flow (L/H)", "Position 1 Speed (RPM)", "Position 2 Serial Number", "Position 2 Elapsed On Time", "Position 2 Controller Current (Adc)", "Position 2 Pump Current (Arms)", "Position 2 Pressure (kPa)", "Position 2 Flow (L/H)", "Position 2 Speed (RPM)", "Position 3 Serial Number", "Position 3 Elapsed On Time", "Position 3 Controller Current (Adc)", "Position 3 Pump Current (Arms)", "Position 3 Pressure (kPa)", "Position 3 Flow (L/H)", "Position 3 Speed (RPM)", "Tank 2 Temp (C)", "Tank 2 Fuel Type", "Position 4 Serial Number", "Position 4 Elapsed On Time", "Position 4 Controller Current (Adc)", "Position 4 Pump Current (Arms)", "Position 4 Pressure (kPa)", "Position 4 Flow (L/H)", "Position 4 Speed (RPM)", "Position 5 Serial Number", "Position 5 Elapsed On Time", "Position 5 Controller Current (Adc)", "Position 5 Pump Current (Arms)", "Position 5 Pressure (kPa)", "Position 5 Flow (L/H)", "Position 5 Speed (RPM)", "Position 6 Serial Number", "Position 6 Elapsed On Time", "Position 6 Controller Current (Adc)", "Position 6 Pump Current (Arms)", "Position 6 Pressure (kPa)", "Position 6 Flow (L/H)", "Position 6 Speed (RPM)"]  # AKLH Header
            n689 = call-poly <vilib>:"Write To Spreadsheet File.vi"("delimiter (\\t)"="," ("delimiter (\\t)"), "append to file? (new file:F)"=TRUE, "1D data"=w1593, "file path (dialog if empty)"=w1594) -> ("new file path (Not A Path if cancelled)"=w1597:path)  [unwired: 4 in]
          }
        }
        n690 = Bundle By Name(cluster=w1589, "AKLH Path"=w1590, "AKLH Timer"=w1572) -> (w1588:T17)
      }
      frame "Save AKLH" {
        n691 = Unbundle By Name(w1628) -> ("AKLH Timer"=w1617:dbl, "AKLH Path"=w1630:path, "App Config.Cycles Completed"=w1626:u32, "Current Step"=w1625:i32, "AKLH Last Hour"=w1619:i32)
        n692 = Get Date/Time In Seconds() -> (seconds since 1Jan1904=w1614:timestamp)
        n693 = Seconds To Date/Time(time stamp (now)=w1614) -> (date time rec=w1624:T34)  [unwired: 1 in]
        n694 = Unbundle By Name(w1624) -> ("hour"=w1615:i32)
        n695 = Format Date/Time String(time format string (%c)="%H:%M", seconds (now)=w1614) -> (date/time string=w1623:string)  [unwired: 1 in]
        n696 = Less Or Equal?(x=w1619, y=w1615) -> (x <= y?=w1618:bool)
        n697 = case shown="True" w1618 {
          tunnel: w1630 -> [w1636 w1679]
          tunnel: w1626 -> [_ w1661]
          tunnel: w1625 -> [_ w1660]
          tunnel: w1623 -> [_ w1645]
          tunnel: [w1636 w1644] -> w1622
          tunnel: w1621 -> [w1634 w1643]
          tunnel: [w1633 w1643] -> w1620
          tunnel: w1617 -> [w1631 _]
          tunnel: [w1631 w1637] -> w1616
          frame False {
            w1632 = T14[] [enum."Init AKLH", enum."Save AKLH"] items=["Main", "Init Files", "Init", "Save As", "Start Profile", "Check Step Time", "Alarm", "Run Step", "Stop Profile", "Cycle Reset", "Time Reset", "Time Reset All", "Time Set", "Tare CTs", "Save Profile", "Open Profile", "Get Profiles", "Update Screen", "Save Status", "Set Manual CMD", "Reset Restarts", "Reset Total Restarts", "Reset Cogs", "Disable Background", "Enable Background", "Get/Release Control", "Init AKLH", "Save AKLH", "Log Fuel Change", "Update Data Stream", "Init TenHz", "Read TenHz", "Remote Timer Reset", "Record Frequency Change", "Controller Change", "Get Alarms", "Init Alarms", "Save Alarms", "Init SubRoutine", "Next SubRoutine"]
            # "This case only happens when the previous read was before midnight and this reading is after midnight\n\nSo just want to get the file corrected to the proper date before saving this data set"
            n698 = Insert Into Array(array=w1634, index=0, new element=w1632) -> (w1633:T14[])
          }
          frame True {
            w1646 = "%d.1"
            # "Should possibly take the data from\nthe shift register and parse it out\nlike is done in the update screen case"
            n699 = local read "ControllerCurrent"() -> (w1675:dbl[])
            n700 = local read "Elapsed Time:"() -> (w1676:dbl[])
            n701 = local read "PumpCurrent"() -> (w1674:dbl[])
            n702 = local read "Pressure"() -> (w1673:dbl[])
            n703 = local read "Speed"() -> (w1671:dbl[])
            n704 = local read "Flow"() -> (w1672:dbl[])
            n705 = local read "Serial Numbers"() -> (w1642:T6)
            n706 = local read "PS Actual (V):"() -> (w1659:dbl)
            n707 = for {
              tunnel: w1676 -> [w1717] mode=indexing
              tunnel: w1675 -> [w1716] mode=indexing
              tunnel: w1674 -> [w1715] mode=indexing
              tunnel: w1673 -> [w1714] mode=indexing
              tunnel: w1672 -> [w1713] mode=indexing
              tunnel: w1671 -> [w1706] mode=indexing
              tunnel: [w1705] -> w1665 mode=indexing
              tunnel: [w1711] -> w1666 mode=indexing
              tunnel: [w1710] -> w1667 mode=indexing
              tunnel: [w1709] -> w1668 mode=indexing
              tunnel: [w1708] -> w1669 mode=indexing
              tunnel: [w1707] -> w1670 mode=indexing
              w1712 = "%d.2"
              n708 = Format Into String(format string="%<%H:%M:%S>t", w1717) -> (resulting string=w1707:string)  [unwired: 2 in, 1 out]
              n709 = Format Into String(format string=w1712, w1716) -> (resulting string=w1708:string)  [unwired: 2 in, 1 out]
              n710 = Format Into String(format string=w1712, w1715) -> (resulting string=w1709:string)  [unwired: 2 in, 1 out]
              n711 = Format Into String(format string=w1712, w1714) -> (resulting string=w1710:string)  [unwired: 2 in, 1 out]
              n712 = Format Into String(format string=w1712, w1713) -> (resulting string=w1711:string)  [unwired: 2 in, 1 out]
              n713 = Number To Decimal String(number=w1706) -> (decimal integer string=w1705:string)  [unwired: 1 in]
            }
            n714 = local read "Tank 1 Fuel Type"() -> (w1639:string)
            n715 = local read "Tank 2 Fuel Type"() -> (w1640:string)
            n716 = local read "Temp1"() -> (w1656:dbl)
            n717 = local read "Temp2"() -> (w1663:dbl)
            n718 = Number To Decimal String(number=w1661) -> (decimal integer string=w1648:string)  [unwired: 1 in]
            n719 = Number To Decimal String(number=w1660) -> (decimal integer string=w1649:string)  [unwired: 1 in]
            n720 = Format Into String(format string="%d.2", w1659) -> (resulting string=w1658:string)  [unwired: 2 in, 1 out]
            n721 = Format Into String(format string=w1646, w1656) -> (resulting string=w1657:string)  [unwired: 2 in, 1 out]
            n722 = Format Into String(format string=w1646, w1663) -> (resulting string=w1662:string)  [unwired: 2 in, 1 out]
            n723 = Cluster To Array(cluster=w1642) -> (array=w1641:string[])
            n724 = Build Array(w1662, w1640) -> (w1651:string[])
            n725 = Interleave 1D Arrays(w1641, w1670, w1669, w1668, w1667, w1666, w1665) -> (w1653:string[])
            n726 = Build Array(w1645, w1648, w1649, w1658, w1657, w1639) -> (w1655:string[])
            n727 = Insert Into Array(array=w1653, index=21, new element=w1651) -> (w1652:string[])
            n728 = disable-structure shown="Disabled" {
              frame Disabled {
                w1681 = 0 ("index")
                w1682 = i16 2 ("precision (6)")
                w1691 = i16 1 ("precision (6)")
                w1704 = 6 ("length")
                n729 = Array Subset(index=0, length=w1704) -> (array=w1699:dbl[], w1697:void[])
                n730 = Index Array(array=w1699, index=21) -> (element=w1698)
                n731 = Array Subset(array=w1699, index=22, length=w1704) -> (w1696:void[])
                n732 = Array Subset(array=w1699, index=28, length=w1704) -> (w1695:void[])
                n733 = Array Subset(array=w1699, index=w1704, length=w1704) -> (w1694:void[])
                n734 = Number To Fractional String(number=w1697, precision (6)=w1682) -> (F-format string=w1690:string[])  [unwired: 2 in]
                n735 = Number To Fractional String(number=w1696, precision (6)=w1691) -> (F-format string=w1689:string[])  [unwired: 2 in]
                n736 = Number To Fractional String(number=w1695, precision (6)=w1691) -> (F-format string=w1688:string[])  [unwired: 2 in]
                n737 = Number To Fractional String(number=w1694, width (-)=i16 4) -> (F-format string=w1687:string[])  [unwired: 2 in]
                n738 = Format Date/Time String(time format string (%c)="%H:%M:%S%2u") -> (seconds (now)=w1680:timestamp, date/time string=w1683:string)  [unwired: 1 in]
                n739 = Number To Fractional String(number=w1698, precision (6)=w1682) -> (F-format string=w1685:string)  [unwired: 2 in]
                n740 = Interleave 1D Arrays(w1690, w1689, w1688, w1687) -> (w1686:string[])
                n741 = Insert Into Array(array=w1686, index=w1681, new element=w1685) -> (w1684:string[])
                n742 = Insert Into Array(array=w1684, index=w1681, new element=w1683) -> ()  [unwired: 1 out]
              }
              frame Enabled {
              }
            }
            n743 = Insert Into Array(array=w1652, index=0, new element=w1655) -> (w1647:string[])
            n744 = Get Date/Time In Seconds() -> (seconds since 1Jan1904=w1638:timestamp)
            n745 = To Double Precision Float(number=w1638) -> (double precision float=w1637:dbl)
            n746 = call-poly <vilib>:"Write To Spreadsheet File.vi"("delimiter (\\t)"="," ("delimiter (\\t)"), "append to file? (new file:F)"=TRUE, "1D data"=w1647, "file path (dialog if empty)"=w1679) -> ("new file path (Not A Path if cancelled)"=w1644:path)  [unwired: 4 in]
          }
        }
        n747 = Bundle By Name(cluster=w1628, "AKLH Timer"=w1616, "AKLH Path"=w1622, "AKLH Last Hour"=w1615) -> (w1627:T17)
      }
      frame "Log Fuel Change" {
        n748 = Get Date/Time In Seconds() -> (seconds since 1Jan1904=w1726:timestamp)
        n749 = Format Date/Time String(time format string (%c)="%H:%M", seconds (now)=w1726) -> (date/time string=w1725:string)  [unwired: 1 in]
        n750 = Unbundle By Name(w1733) -> ("AKLH Path"=w1731:path)
        n751 = Replace Array Subset(array=string[] ["", "Fuel", "Changed"], new element=w1725, index=0) -> (w1722:string[])
        n752 = call-poly <vilib>:"Write To Spreadsheet File.vi"("delimiter (\\t)"="," ("delimiter (\\t)"), "append to file? (new file:F)"=TRUE, "1D data"=w1722, "file path (dialog if empty)"=w1731) -> ("new file path (Not A Path if cancelled)"=w1730:path)  [unwired: 4 in]
        n753 = Bundle By Name(cluster=w1733, "AKLH Path"=w1730) -> (w1732:T17)
        n754 = case shown="True" FALSE {
          tunnel: w1721 -> [w1734 w1738]
          tunnel: [w1734 w1737] -> w1720
          frame False {
          }
          frame True {
            w1735 = T14[] [enum."Remote Timer Reset"] items=["Main", "Init Files", "Init", "Save As", "Start Profile", "Check Step Time", "Alarm", "Run Step", "Stop Profile", "Cycle Reset", "Time Reset", "Time Reset All", "Time Set", "Tare CTs", "Save Profile", "Open Profile", "Get Profiles", "Update Screen", "Save Status", "Set Manual CMD", "Reset Restarts", "Reset Total Restarts", "Reset Cogs", "Disable Background", "Enable Background", "Get/Release Control", "Init AKLH", "Save AKLH", "Log Fuel Change", "Update Data Stream", "Init TenHz", "Read TenHz", "Remote Timer Reset", "Record Frequency Change", "Controller Change", "Get Alarms", "Init Alarms", "Save Alarms", "Init SubRoutine", "Next SubRoutine"]
            # "If tenhz is active I should have a way to insert\na line for fuel change... at the correct location"
            n755 = Insert Into Array(array=w1738, index=0, new element=w1735) -> (w1737:T14[])
          }
        }
      }
      frame "Update Data Stream" {
        # "...probably scrapping the idea of traces"
        # "UNACCESSIBLE"
        "Graph" <- dbl[] [] ("Waveform Graph 2")
      }
      frame "Init TenHz" {
        w1742 = string[] ["Time", "Position 1 Voltage (V)", "Position 2 Voltage (V)", "Position 3 Voltage (V)", "Position 4 Voltage (V)", "Position 5 Voltage (V)", "Position 6 Voltage (V)", "Power Supply Voltage (V)", "Position 1 Pump Current (A)", "Position 2 Pump Current (A)", "Position 3 Pump Current (A)", "Position 4 Pump Current (A)", "Position 5 Pump Current (A)", "Position 6 Pump Current (A)", "Position 1 Pump Speed (RPM)", "Position 2 Pump Speed (RPM)", "Position 3 Pump Speed (RPM)", "Position 4 Pump Speed (RPM)", "Position 5 Pump Speed (RPM)", "Position 6 Pump Speed (RPM)", "Position 1 Controller Current (A RMS)", "Position 2 Controller Current (A RMS)", "Position 3 Controller Current (A RMS)", "Position 4 Controller Current (A RMS)", "Position 5 Controller Current (A RMS)", "Position 6 Controller Current (A RMS)", "Tank 1 Temperature (Deg. C)", "Tank 2 Temperature (Deg. C)", "Position 1 Pressure (kPa)", "Position 2 Pressure (kPa)", "Position 3 Pressure (kPa)", "Position 4 Pressure (kPa)", "Position 5 Pressure (kPa)", "Position 6 Pressure (kPa)", "Position 1 Flow (L/H)", "Position 2 Flow (L/H)", "Position 3 Flow (L/H)", "Position 4 Flow (L/H)", "Position 5 Flow (L/H)", "Position 6 Flow (L/H)", "Position 1 Elapsed Time", "Position 2 Elapsed Time", "Position 3 Elapsed Time", "Position 4 Elapsed Time", "Position 5 Elapsed Time", "Position 6 Elapsed Time"]  # TenHz Header
        n756 = Unbundle By Name(w1757) -> ("TenHz Path"=w1767:path, "App Config.Location"=w1764:string, "App Config.CA Number"=w1763:string, "App Config.TenHzFrequency"=w1744:u32)
        n757 = Get Date/Time In Seconds() -> (seconds since 1Jan1904=w1761:timestamp)
        n758 = case shown="10, Default" w1744 {
          tunnel: ["One" "Two" "Three" "Four" "Five" "Six" "Seven" "Eight" "Nine" "Ten"] -> w1743
          frame 1 {
          }
          frame 2 {
          }
          frame 3 {
          }
          frame 4 {
          }
          frame 5 {
          }
          frame 6 {
          }
          frame 7 {
          }
          frame 8 {
          }
          frame 9 {
          }
          frame 10, Default {
          }
        }
        n759 = call "Timestamp2DayofYear.vi"("time stamp"=w1761) -> ("time string"=w1760:string)  [unwired: 14 in]
        n760 = Concatenate Strings(w1743, " Hertz Data " ("string"), w1764, " CA" ("string"), w1763, " " ("string"), w1760) -> (w1754:string)
        n761 = Strip Path(path=w1767) -> (stripped path=w1766:path)  [unwired: 1 out]
        n762 = Concatenate Strings(w1754, ".csv" ("string")) -> (w1758:string)
        n763 = Build Path(base path=w1766, name or relative path=w1758) -> (appended path=w1753:path)
        n764 = while {
          tunnel: w1754 -> [w1785]
          shift-right: [w1779] -> w1752
          shift-left: w1753 -> [w1778]
          i -> [w1784]
          stop <- w1780 continue-if-true
          n765 = call <vilib>:"Check if File or Folder Exists.vi"("path"=w1778) -> ("file or folder exists?"=w1782:bool, "dup path"=w1786:path)  [unwired: 8 in, 1 out]
          n766 = Add(x=2, y=w1784) -> (x+y=w1788:i32)
          n767 = Not Equal?(x=w1784, y=8) -> (x != y?=w1781:bool)
          n768 = case shown="True" w1782 {
            tunnel: w1786 -> [w1794 w1796]
            tunnel: [w1789 w1796] -> w1779
            tunnel: w1785 -> [w1792 _]
            tunnel: w1788 -> [w1791 _]
            frame True {
              n769 = Strip Path(path=w1794) -> (stripped path=w1795:path)  [unwired: 1 out]
              n770 = Format Into String(format string="%s_%d.csv", w1792, w1791) -> (resulting string=w1790:string)  [unwired: 2 in, 1 out]
              n771 = Build Path(base path=w1795, name or relative path=w1790) -> (appended path=w1789:path)
            }
            frame False {
            }
          }
          n772 = And(x=w1782, y=w1781) -> (x .and. y?=w1780:bool)
        }
        n773 = Get Date/Time In Seconds() -> (seconds since 1Jan1904=w1748:timestamp)
        n774 = Seconds To Date/Time(time stamp (now)=w1748) -> (date time rec=w1749:T34)  [unwired: 1 in]
        n775 = Unbundle By Name(w1749) -> ("day of month"=w1747:i32)
        n776 = call-poly <vilib>:"Write To Spreadsheet File.vi"("delimiter (\\t)"="," ("delimiter (\\t)"), "append to file? (new file:F)"=TRUE, "1D data"=w1742, "file path (dialog if empty)"=w1752) -> ("new file path (Not A Path if cancelled)"=w1746:path)  [unwired: 4 in]
        n777 = Bundle By Name(cluster=w1757, "TenHz Day"=w1747, "TenHz Path"=w1746) -> (w1756:T17)
        n778 = local write "TenHz Path"(w1746) -> ()
      }
      frame "Read TenHz" {
        (unwired) string[] ["AI-00/08_Voltage_1", "AI-01/09_Voltage_2", "AI-02/10_Voltage_3", "AI-03/11_Voltage_4", "AI-04/12_Voltage_5", "AI-05/13_Voltage_6", "AI-06_Spare", "AI-14_Spare", "AI-07_Spare", "AI-15_PS_Sense", "AI-16_Pump_Current_1", "AI-17_Pump_Current_2", "AI-18_Pump_Current_3", "AI-19_Pump_Current_4", "AI-20_Pump_Current_5", "AI-21_Pump_Current_6", "AI-16_Pump_Speed_1", "AI-17_Pump_Speed_2", "AI-18_Pump_Speed_3", "AI-19_Pump_Speed_4", "AI-20_Pump_Speed_5", "AI-21_Pump_Speed_6", "AI-22_Controller_Current_1", "AI-23_Controller_Current_2", "AI-24_Controller_Current_3", "AI-25_Controller_Current_4", "AI-26_Controller_Current_5", "AI-27_Controller_Current_6", "AI-28_Temperature_1", "AI-29_Temperature_2", "AI-30_Pump_Pressure_1", "AI-31_Pump_Pressure_2", "AI-32_Pump_Pressure_3", "AI-33_Pump_Pressure_4", "AI-34_Pump_Pressure_5", "AI-35_Pump_Pressure_6", "AI-36_Pump_Flow_1", "AI-37_Pump_Flow_2", "AI-38_Pump_Flow_3", "AI-39_Pump_Flow_4", "AI-40_Pump_Flow_5", "AI-41_Pump_Flow_6", "AI-42_Spare", "AI-43_Spare", "AI-44_Spare", "AI-45_Spare", "AI-46_Spare", "AI-47_Spare", "Pump_Elapsed_Time_1", "Pump_Elapsed_Time_2", "Pump_Elapsed_Time_3", "Pump_Elapsed_Time_4", "Pump_Elapsed_Time_5", "Pump_Elapsed_Time_6"]  # Channel Reference
        n779 = Unbundle By Name(w1819) -> ("Controller List"=w1807:T10, "Trip Counters"=w1804:i32[], "Previous Times"=w1803:u32[], "Alarm Config"=w1808:T7, "App Config.Pumps Present"=w1809:u32, "Intitial Times"=w1830:dbl[], "Power Relay"=w1826:T2, "Manual CMDs"=w1810:dbl[], "App Config.Location"=w1825:string, "App Config.Current Profile"=w1824:string, "App Config.CA Number"=w1823:string, "PS CMD"=w1822:dbl, "Press CMD"=w1821:dbl, "Temp CMD"=w1820:dbl, "Run Profile"=w1811:bool, "App Config.Controller Type:"=w1806:T5)
        n780 = disable-structure shown="Enabled" {
          disable-tunnel: [w1837 w1839] -> w1797
          disable-tunnel: w1798 -> [_ w1844]
          frame Disabled {
            n781 = call "Tank Data Global.vi"() -> ("Tank Data OUT"=w1837:dbl[])  [unwired: 11 in]
          }
          frame Enabled {
            n782 = xnode "Read/Write Control"("FPGA VI Reference In"=w1844) -> ("Currents (RMS)"=w1858:fxp<+,26,7>[], "Speed (RPM)"=w1859:fxp<+,32,18>[], "Temp"=w1860:fxp<+/-,20,12>, "Temp 2"=w1861:fxp<+/-,20,12>, "Elapsed Times"=w1862:u64[])  [unwired: 1 in, 2 out]
            n783 = To Double Precision Float(number=w1858) -> (double precision float=w1840:dbl[])
            n784 = To Double Precision Float(number=w1859) -> (double precision float=w1852:dbl[])
            n785 = To Double Precision Float(number=w1860) -> (double precision float=w1851:dbl)
            n786 = To Double Precision Float(number=w1861) -> (double precision float=w1850:dbl)
            n787 = To Double Precision Float(number=w1862) -> (double precision float=w1843:dbl[])
            n788 = Replace Array Subset(array=dbl[] [0.0, 0.0, 0.0, 0.0, 0.0, 0.0, 0.0, 0.0, 0.0, 0.0, 0.0, 0.0, 0.0, 0.0, 0.0, 0.0, 0.0, 0.0, 0.0, 0.0, 0.0, 0.0, 0.0, 0.0, 0.0, 0.0, 0.0, 0.0, 0.0, 0.0, 0.0, 0.0, 0.0, 0.0, 0.0, 0.0, 0.0, 0.0, 0.0, 0.0, 0.0, 0.0, 0.0, 0.0, 0.0, 0.0, 0.0, 0.0, 0.0, 0.0, 0.0, 0.0, 0.0, 0.0], new element=w1840, index=10) -> (w1856:dbl[])
            n789 = Replace Array Subset(array=w1856, new element=w1852, index=16) -> (w1855:dbl[])
            n790 = Divide(x=w1843, y=10000) -> (x/y=w1841:dbl[])
            n791 = Replace Array Subset(array=w1855, new element=w1851, index=28) -> (w1854:dbl[])
            n792 = Replace Array Subset(array=w1854, new element=w1850, index=29) -> (w1853:dbl[])
            n793 = Replace Array Subset(array=w1853, new element=w1841, index=48) -> (w1839:dbl[])
            n794 = call "Tank Data Global.vi"("Pump Data Mode"=Pump_Data_Mode."Write Data", "Tank Data IN"=w1839) -> ()  [unwired: 9 in, 1 out]
          }
        }
        n795 = Index Array(array=w1807, index=w1806) -> (element=w1805:T11)
        n796 = case shown="\"Kuhnke\", Default" w1806 {
          tunnel: [100 ("CMD Max") 1000 ("CMD Max")] -> w1814
          tunnel: [1 ("CMD Max") 10 ("CMD Max")] -> w1813
          frame "Kuhnke", Default {
          }
          frame "Conti" {
          }
        }
        n797 = Number To Boolean Array(number=w1809) -> (Boolean array=w1829:bool[])
        n798 = call "Signal Breakout.vi"("Pumps Enabled"=w1829, "Tank Data"=w1797, "Intitial Times"=w1830) -> ("Pump Data"=w1828:T19, "Tank Data"=w1827:T37)  [unwired: 10 in, 1 out]
        n799 = Bundle("Location"=w1825, "Current Profile"=w1824, "CA Number"=w1823) -> (w1832:T38)  [unwired: 1 in]
        n800 = Bundle("PS CMD"=w1822, "Press CMD"=w1821, "Temp CMD"=w1820) -> (w1831:T39)  [unwired: 1 in]
        n801 = Bundle By Name(cluster=T23 {"Controller List"="", "Controller Type:"=enum."Kuhnke", "CMD Max"=0, "CMD Inc"=0} ("Controller Config"), "Controller Type:"=w1806, "CMD Max"=w1814, "CMD Inc"=w1813) -> (w1815:T23)
        n802 = call "Evaluate Alarms.vi"("In Test"=w1811, "Controller"=w1805, "Alarm Config"=w1808, "Data"=w1797, "Pumps Present"=w1809, "Trip Counter"=w1804, "Previous Times"=w1803, "Manual CMDs"=w1810) -> ("Trip Counter OUT"=w1802:i32[], "Previous Times OUT"=w1801:u32[], "Alarm Tripped"=w1800:bool, "Alarm Message"=w1799:string)  [unwired: 16 in]
        n803 = Bundle By Name(cluster=T22 {"Start Test"=FALSE, "Toggle Spare 1"=FALSE, "Toggle Spare 2"=FALSE, "Toggle Spare 3"=FALSE, "Toggle Spare 4"=FALSE, "Toggle Spare 5"=FALSE} ("HMI Tog Buttons"), "Start Test"=w1811) -> (w1817:T22)
        n804 = call "RPi HMI Com.vi"("Pump Data"=w1828, "Tank Data"=w1827, "Power Relays"=w1826, "Pump CMDs"=w1810, "HMI Header"=w1832, "Tank CMDs"=w1831, "HMI Tog Buttons"=w1817, "RPi HMI Mode"=RPi_HMI_Mode."Write Data", "In Test"=w1811, "Controller Config"=w1815) -> ()  [unwired: 9 in, 1 out]
        n805 = Get Date/Time In Seconds() -> (seconds since 1Jan1904=w1836:timestamp)
        n806 = To Double Precision Float(number=w1836) -> (double precision float=w1812:dbl)
        n807 = Bundle By Name(cluster=w1819, "TenHz Timer"=w1812, "Tank Data"=w1797, "Trip Counters"=w1802, "Previous Times"=w1801, "Alarm"=w1800, "Alarm Message"=w1799) -> (w1835:T17)
      }
      frame "Record Frequency Change" {
        # "was switching in the globals for controlling the logging of \"tenhz\""
        # "60 seconds times 7 min recording period and decremented to point at the correct index"
        n808 = local read "Record Frequency:"() -> (w1872:i32)
        n809 = Multiply(x=w1872, y=420) -> (x*y=w1869:i32)
        n810 = case shown="10, Default" w1872 {
          tunnel: [u32 1000 ("milliseconds to wait") u32 500 ("milliseconds to wait") u32 333 ("milliseconds to wait") u32 250 ("milliseconds to wait") u32 200 ("milliseconds to wait") u32 167 ("milliseconds to wait") u32 143 ("milliseconds to wait") u32 125 ("milliseconds to wait") u32 111 ("milliseconds to wait") u32 100 ("milliseconds to wait")] -> w1867
          frame 1 {
          }
          frame 2 {
          }
          frame 3 {
            # "0.1% slow"
          }
          frame 4 {
          }
          frame 5 {
          }
          frame 6 {
            # "0.2% fast"
          }
          frame 7 {
            # "0.1% fast"
          }
          frame 8 {
          }
          frame 9 {
            # "0.1% slow"
          }
          frame 10, Default {
          }
        }
        n811 = Decrement(x=w1869) -> (x-1=w1868:i32)
        n812 = global write "Record Period (global).vi" "Record Period (ms)"(w1867) -> ()
        n813 = global write "Record Samples (global).vi" "Record Samples"(w1868) -> ()
      }
      frame "Controller Change" {
        n814 = flat-sequence {
          tunnel: [w1913] -> w1888
          tunnel: [w1912] -> w1887
          tunnel: [w1898] -> w1884
          tunnel: w1885 -> [w1899]
          tunnel: w1886 -> [w1907]
          tunnel: w1885 -> [w1911]
          tunnel: w1888 -> [w1940]
          tunnel: w1887 -> [w1929]
          frame #0 {
            w1894 = dbl[] [0.0, 0.0, 0.0, 0.0, 0.0, 0.0] ("ControllerCurrent")
            n815 = Unbundle By Name(w1911) -> ("Controller List"=w1891:T10, "App Config.Controller Type:"=w1897:T5)
            n816 = Index Array(array=w1891, index=w1897) -> (element=w1893:T11)
            n817 = Unbundle By Name(w1893) -> ("Frequency"=w1895:i32, "CommSeg"=w1896:i32, "Controller?"=w1912:bool, "High Command"=w1901:dbl, "Low Command"=w1902:dbl, "Command Step"=w1903:dbl, "Stop Command"=w1904:dbl, "Invert PWM"=w1892:bool, "Controller Name"=w1890:T5)
            n818 = Equal?(x=2, y=w1896) -> (x = y?=w1913:bool)
            n819 = case shown="False" w1913 {
              tunnel: [w1924 fxp<+,32,16> 1.0 ("CommFactor")] -> w1909
              tunnel: w1896 -> [w1925 _]
              frame False {
                n820 = case shown="10, Default" w1925 {
                  tunnel: [fxp<+,32,16> 4.0 ("CommFactor") fxp<+,32,16> 5.0 ("CommFactor")] -> w1924
                  frame 8 {
                  }
                  frame 10, Default {
                  }
                }
              }
              frame True {
              }
            }
            n821 = property on="ControllerCurrent" class="Arr (strict)"("Value"=w1894) -> ()  [unwired: 2 in, 2 out]
            n822 = local write "ControllerCurrent"(w1894) -> ()
            n823 = Divide(x=40000000.0 ("40 MHz"), y=w1895) -> (x/y=w1906:dbl)
            n824 = To Unsigned Long Integer(number=w1906) -> (unsigned 32bit integer=w1900:u32)
            n825 = disable-structure shown="Enabled" {
              disable-tunnel: w1913 -> [w1919 _]
              disable-tunnel: w1909 -> [w1918 _]
              disable-tunnel: "RPMhyst" -> [w1917 w1920]
              disable-tunnel: w1907 -> [w1916 w1923]
              disable-tunnel: w1900 -> [w1915 w1922]
              disable-tunnel: w1892 -> [w1914 _]
              disable-tunnel: w1890 -> [_ w1921]
              frame Disabled {
                n826 = xnode "Read/Write Control"("FPGA VI Reference In"=w1916, "Brushless"=w1919, "CommFactor"=w1918, "RPMhyst"=w1917, "PWM Period (Ticks)"=w1915, "InvertPWM?"=w1914) -> ()  [unwired: 1 in, 2 out]
              }
              frame Enabled {
                n827 = xnode "Read/Write Control"("FPGA VI Reference In"=w1923, "Speed Hysteresis"=w1920, "PWM Period (Ticks)"=w1922, "Controller Type:"=w1921) -> ()  [unwired: 2 in, 2 out]
              }
            }
            n828 = property on="Numeric" class="DigNum (strict)"("Maximum"=w1901, "Minimum"=w1902, "Increment"=w1903) -> ()  [unwired: 2 in, 2 out]
            n829 = Bundle By Name(cluster=w1899, "Stop Cmd"=w1904, "Controller"=w1893) -> (w1898:T17)
          }
          frame #1 {
            # "This should be controlled by the\nDip switch and chosen as the\ndata set not set by pump type"
            n830 = Select(t="Controller\nVoltage\n(V)" ("Caption.Text"), s=FALSE, f="Pump\nVoltage\n(V)" ("Caption.Text")) -> (s? t:f=w1933:string)
            n831 = Select(t="Pump\nCurrent\n(RMS)" ("Label.Text"), s=w1940, f="Pump\nCurrent\n(DC)" ("Label.Text")) -> (s? t:f=w1935:string)
            n832 = Select(t=T27."Enabled" ("Disabled"), s=w1929, f=T27."Disabled and Grayed Out" ("Disabled")) -> (s? t:f=w1936:T27)
            n833 = property on="Voltages" class="Arr (strict)"("Caption.Text"=w1933) -> ()  [unwired: 2 in, 2 out]
            n834 = property on="PumpCurrent" class="Arr (strict)"("Caption.Text"=w1935) -> ()  [unwired: 2 in, 2 out]
            n835 = property on="ControllerCurrent" class="Arr (strict)"("DisabledEnum"=w1936) -> ()  [unwired: 2 in, 2 out]
          }
        }
      }
      frame "Init SubRoutine" {
        w1947 = u32 0 ("t")
        n836 = Unbundle By Name(w1946) -> ("App Config.Profiles Path"=w1961:path, "SubRoutine Profile"=w1952:i32[][])
        n837 = property on="Profile Name:" class="CmbBox"() -> ("Strings[]"=w1942:string[])  [unwired: 2 in, 2 out]
        n838 = Index Array(array=w1952, index (row)=w1947) -> (element=w1951:i32[])  [unwired: 1 in]
        n839 = Index Array(array=w1951) -> (element #1=w1950:i32, element #2=w1948:i32)  [unwired: 2 in]
        n840 = Decrement(x=w1950) -> (x-1=w1949:i32)
        n841 = Index Array(array=w1942, index=w1949) -> (element=w1943:string)
        n842 = Build Path(base path=w1961, name or relative path=w1943) -> (appended path=w1959:path)
        n843 = local write "Profile Name:"(w1943) -> ()
        n844 = Read from Text File(file (use dialog)=w1959) -> (refnum out=w1957:refnum<file>, text=w1958:string, error out=w1956:errorcluster)  [unwired: 3 in, 1 out]
        n845 = Close File(refnum=w1957, error in=w1956) -> (error out=w1955:errorcluster)  [unwired: 1 out]
        n846 = case shown="No Error" w1955 {
          tunnel: w1958 -> [w1963 _]
          tunnel: [w1964 string[][] []] -> w1944
          frame No Error {
            n847 = Spreadsheet String To Array(delimiter (Tab)=",", format string="%s", spreadsheet string=w1963, array type (2D Dbl)=string[][] []) -> (array=w1964:string[][])
          }
          frame Error {
          }
        }
        n848 = Array Size(array=w1944) -> (size(s)=w1960:i32[])
        n849 = local write "Profile:"(w1944) -> ()
        n850 = Index Array(array=w1960) -> (element=w1953:i32)  [unwired: 1 in]
        n851 = Bundle By Name(cluster=w1946, "Profile"=w1944, "# of Steps"=w1953, "Update Profile"=TRUE, "App Config.Current Profile"=w1943, "ReqCycles"=w1948, "SR Step"=w1947) -> (w1945:T17)
      }
      frame "Next SubRoutine" {
        n852 = Unbundle By Name(w1973) -> ("App Config.Profiles Path"=w1994:path, "SubRoutine Profile"=w1979:i32[][], "SR Step"=w1984:u32)
        n853 = Increment(x=w1984) -> (x+1=w1981:u32)
        n854 = Array Size(array=w1979) -> (size(s)=w1985:i32[])
        n855 = Index Array(array=w1985) -> (element=w1982:i32)  [unwired: 1 in]
        n856 = Less Or Equal?(x=w1982, y=w1981) -> (x <= y?=w1980:bool)
        n857 = Select(t=u32 0, s=w1980, f=w1981) -> (s? t:f=w1974:u32)
        n858 = Index Array(array=w1979, index (row)=w1974) -> (element=w1978:i32[])  [unwired: 1 in]
        n859 = property on="Profile Name:" class="CmbBox"() -> ("Strings[]"=w1970:string[])  [unwired: 2 in, 2 out]
        n860 = Index Array(array=w1978) -> (element #1=w1977:i32, element #2=w1975:i32)  [unwired: 2 in]
        n861 = Decrement(x=w1977) -> (x-1=w1976:i32)
        n862 = Index Array(array=w1970, index=w1976) -> (element=w1969:string)
        n863 = Build Path(base path=w1994, name or relative path=w1969) -> (appended path=w1992:path)
        n864 = local write "Profile Name:"(w1969) -> ()
        n865 = Read from Text File(file (use dialog)=w1992) -> (refnum out=w1990:refnum<file>, text=w1991:string, error out=w1989:errorcluster)  [unwired: 3 in, 1 out]
        n866 = Close File(refnum=w1990, error in=w1989) -> (error out=w1988:errorcluster)  [unwired: 1 out]
        n867 = case shown="No Error" w1988 {
          tunnel: w1991 -> [w1996 _]
          tunnel: [w1997 string[][] []] -> w1971
          frame No Error {
            n868 = Spreadsheet String To Array(delimiter (Tab)=",", format string="%s", spreadsheet string=w1996, array type (2D Dbl)=string[][] []) -> (array=w1997:string[][])
          }
          frame Error {
          }
        }
        n869 = Array Size(array=w1971) -> (size(s)=w1993:i32[])
        n870 = local write "Profile:"(w1971) -> ()
        n871 = Index Array(array=w1993) -> (element=w1986:i32)  [unwired: 1 in]
        n872 = Bundle By Name(cluster=w1973, "Profile"=w1971, "# of Steps"=w1986, "Update Profile"=TRUE, "App Config.Current Profile"=w1969, "ReqCycles"=w1975, "SR Step"=w1974) -> (w1972:T17)
      }
    }
  }
  n873 = while {
    shift-right: [w2008] -> _
    shift-left: w38 -> [w2009]
    shift-right: [w2006] -> _
    shift-left: dbl[] [0.0, 0.0, 0.0, 0.0, 0.0, 0.0, 0.0, 0.0, 0.0, 0.0, 0.0, 0.0, 0.0, 0.0, 0.0, 0.0, 0.0, 0.0, 0.0, 0.0, 0.0, 0.0, 0.0, 0.0, 0.0, 0.0, 0.0, 0.0, 0.0, 0.0, 0.0, 0.0, 0.0, 0.0, 0.0, 0.0, 0.0, 0.0, 0.0, 0.0, 0.0, 0.0, 0.0, 0.0, 0.0, 0.0, 0.0] -> [w2004]
    shift-right: [w2007] -> _
    shift-left: 0 -> [w2005]
    tunnel: w45 -> [_]
    shift-right: [w2002] -> _
    shift-left: _ -> [w2001]
    stop <- FALSE stop-if-true
    n874 = local read "pb.TenHzSave"() -> (w2003:bool)
    n875 = case shown="True" w2003 {
      tunnel: w2009 -> [w2017 w2051]
      tunnel: [w2017 w2049] -> w2008
      tunnel: [0 w2048] -> w2007
      tunnel: [w2015 w2018] -> w2006
      tunnel: w2005 -> [_ w2047]
      tunnel: w2004 -> [w2015 w2046]
      tunnel: [w2012 w2037] -> w2002
      tunnel: w2001 -> [_ w2036]
      frame False {
        n876 = Get Date/Time In Seconds() -> (seconds since 1Jan1904=w2011:timestamp)
        n877 = Seconds To Date/Time(time stamp (now)=w2011) -> (date time rec=w2013:T34)  [unwired: 1 in]
        n878 = Wait (ms)(milliseconds to wait=u32 10000) -> ()  [unwired: 1 out]
        n879 = Unbundle By Name(w2013) -> ("day of month"=w2012:i32)
      }
      frame True {
        n880 = Get Date/Time In Seconds() -> (seconds since 1Jan1904=w2040:timestamp)
        n881 = global read "Record Period (global).vi" "Record Period (ms)"() -> (w2042:u32)
        n882 = To Double Precision Float(number=w2040) -> (double precision float=w2044:dbl)
        n883 = Seconds To Date/Time(time stamp (now)=w2040) -> (date time rec=w2041:T34)  [unwired: 1 in]
        n884 = Replace Array Subset(array=w2046, new element=w2044, index=0) -> (w2020:dbl[])
        n885 = Unbundle By Name(w2041) -> ("day of month"=w2037:i32)
        n886 = call "Tank Data Global.vi"() -> ("Tank Data OUT"=w2019:dbl[])  [unwired: 11 in]
        n887 = Wait (ms)(milliseconds to wait=w2042) -> ()  [unwired: 1 out]
        n888 = Array Subset(array=w2019, index=0, length=6) -> (w2023:dbl[])
        n889 = Not Equal?(x=w2037, y=w2036) -> (x != y?=w2035:bool)
        n890 = Replace Array Subset(array=w2020, new element=w2023, index=1) -> (w2033:dbl[])
        n891 = Array Subset(array=w2019, index=9, length=33) -> (w2024:dbl[])
        n892 = global read "Record Samples (global).vi" "Record Samples"() -> (w2043:i32)
        n893 = Replace Array Subset(array=w2033, new element=w2024, index=7) -> (w2034:dbl[])
        n894 = Array Subset(array=w2019, index=48, length=6) -> (w2029:dbl[])
        n895 = Replace Array Subset(array=w2034, new element=w2029, index=40) -> (w2018:dbl[])
        n896 = Equal?(x=w2047, y=w2043) -> (x = y?=w2039:bool)
        n897 = Replace Array Subset(array=w2051, new element=w2018, index (row)=w2047) -> (w2050:dbl[][])  [unwired: 1 in]
        n898 = Or(x=w2039, y=w2035) -> (x .or. y?=w2038:bool)
        n899 = case shown="True" w2038 {
          tunnel: w2050 -> [w2054 w2055]
          tunnel: [w2054 dbl[][] array4200x47[197400 elements]] -> w2049
          tunnel: [w2053 0] -> w2048
          tunnel: w2047 -> [w2052 w2058]
          tunnel: w2035 -> [_ w2060]
          frame False {
            n900 = Increment(x=w2052) -> (x+1=w2053:i32)
          }
          frame True {
            n901 = Boolean To (0,1)(Boolean=w2060) -> (0, 1=w2059:i16)
            n902 = Negate(x=w2059) -> (-x=w2057:i16)
            n903 = Add(x=w2058, y=w2057) -> (x+y=w2056:i32)
            n904 = stacked-sequence {
              tunnel: w2056 -> [w2063 _]
              tunnel: w2055 -> [_ w2064]
              frame #0 {
                "TenHzPts" <- w2063
              }
              frame #1 {
                n905 = global write "TenHzDataArray(Global).vi" "TenHzDataArray"(w2064) -> ()
              }
            }
          }
        }
      }
    }
  }
  n906 = global write "TenHzDataArray(Global).vi" "TenHzDataArray"(w38) -> ()
  n907 = while {
    stop <- FALSE stop-if-true
    n908 = property class="App"() -> ("RemotePanel.ConnToClients"=w2069:T40)  [unwired: 2 in, 2 out]
    n909 = Array Size(array=w2069) -> (size(s)=w2072:i32)
    n910 = Greater Than 0?(x=w2072) -> (x > 0?=w2065:bool)
    "Client?" <- w2065
    n911 = Wait (ms)(milliseconds to wait=u32 500) -> ()  [unwired: 1 out]
    n912 = feedback #2() -> (w2071:bool)  [unwired: 1 in]
    n913 = feedback-in #2(w2065) -> ()
    n914 = Greater?(x=w2071, y=w2065) -> (0:w2070:bool)
    n915 = call <vilib>:"RT Get CPU Loads.vi"() -> ("CPU loads"=w2067:T41[])  [unwired: 10 in, 1 out]
    n916 = case shown="True" w2070 {
      frame False {
      }
      frame True {
        n917 = local write "Login"(FALSE ("Login")) -> ()
      }
    }
    n918 = Index Array(array=w2067) -> (element=w2068:T41)  [unwired: 1 in]
    n919 = Unbundle By Name(w2068) -> ("Total (%)"=→"CPU Usage:":dbl)
    n920 = case shown="True" w2065 {
      frame False {
        n921 = property class="App"("WebSrvr.TCPAccessList"=string[] ["c+*"] ("Web Server:TCP/IP Access List")) -> ()  [unwired: 2 in, 2 out]
      }
      frame True {
        n922 = property class="App"("WebSrvr.TCPAccessList"=string[] ["-*"] ("Web Server:TCP/IP Access List")) -> ()  [unwired: 2 in, 2 out]
      }
    }
  }
  n923 = while {
    shift-right: [w2084] -> _
    shift-left: _ -> [w2085]
    tunnel: w45 -> [_]
    stop <- FALSE stop-if-true
    w2082 = 0 ("index (row)")
    n924 = global read "TenHzDataArray(Global).vi" "TenHzDataArray"() -> (w2081:dbl[][])
    n925 = local read "pb.TenHzSave"() -> (w2080:bool)
    n926 = Wait (ms)(milliseconds to wait=u32 10000) -> ()  [unwired: 1 out]
    n927 = Index Array(array=w2081, index (row)=w2082, index (col)=w2082) -> (element=w2084:dbl)
    n928 = Not Equal?(x=w2084, y=w2085) -> (x != y?=w2079:bool)
    n929 = And(x=w2079, y=w2080) -> (x .and. y?=w2078:bool)
    n930 = case shown="True" w2078 {
      tunnel: w2081 -> [_ w2089]
      frame False {
      }
      frame True {
        n931 = local read "TenHzPts"() -> (w2087:i32)
        n932 = Increment(x=w2087) -> (x+1=w2088:i32)
        n933 = Array Subset(array=w2089, index (row)=0 ("index"), length (row)=w2088) -> (w2090:dbl[][])  [unwired: 2 in]
        n934 = call-poly <vilib>:"Write To Spreadsheet File.vi"("delimiter (\\t)"="," ("delimiter (\\t)"), "append to file? (new file:F)"=TRUE, "2D data"=w2090, "file path (dialog if empty)"="TenHz Path") -> ()  [unwired: 4 in, 1 out]
      }
    }
  }
  n935 = disable-structure shown="Disabled" {
    frame Disabled {
      w2095 = dbl[] [0.0, 0.0, 0.0, 0.0, 0.0, 0.0]  # Manual PWMs
      # "Don't know why this was sitting here"
      n936 = local write "Manual\nCMD"(w2095) -> ()
    }
    frame Enabled {
    }
  }
